vi "Variant_KVP to Strict Variant (Standard).vi"(6 "KVP":variant, 8 "Strict type matching? (F)":bool, 9 "Default Value Name (empty: label)":string, 10 "Default Value":variant, 11 "Parent Name":string) -> (0 "all found?":bool, 1 "any found?":bool, 2 "Value":variant, 3 "name out":string)   [LabVIEW 2020, in "OpenVariant.lvlib"]
doc: "This VI takes a default value as the input and replaces it recursively (cluster, array) with values found in key value pair arrays."
uses:
  OpenVariant.lvlib
  Variant_EmptyCluster.vi
  _built_ppls/OpenDescriptor.lvlibp/TypeDescriptor_SetName.vi
  <vilib>/Utility/GetType.llb/TD_Create Cluster.vi
  <vilib>/Utility/GetType.llb/TD_Get Array Information.vi
  <vilib>/Utility/GetType.llb/Get Type Code from I16 Array And Pos.vi
  _built_ppls/OpenConvert.lvlibp
  _built_ppls/OpenScalar.lvlibp
  _built_ppls/OpenDescriptor.lvlibp
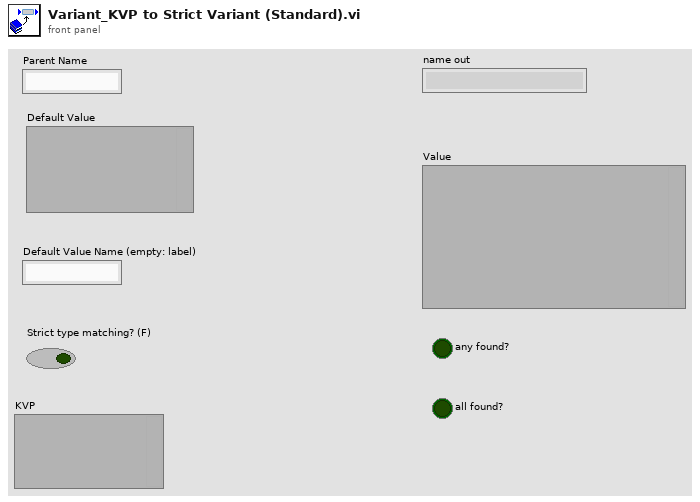
[diagram p1: front panel]
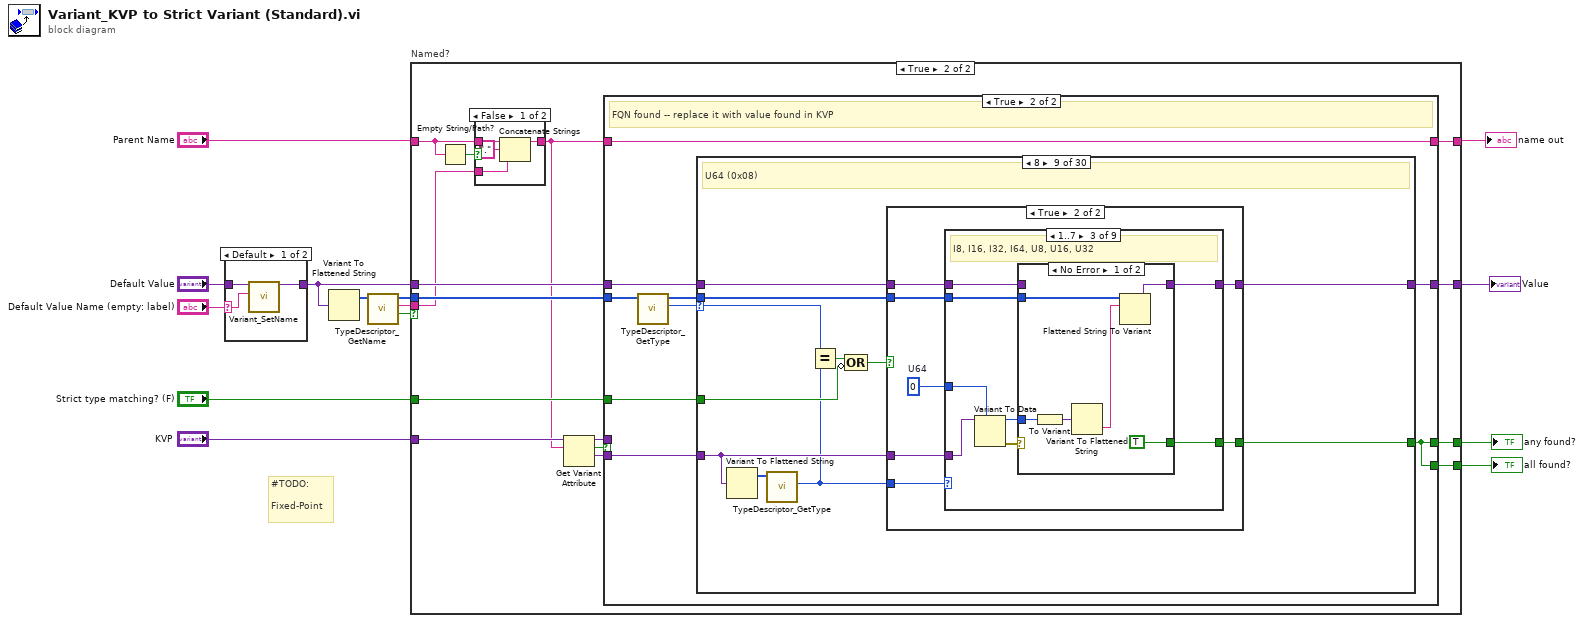
[diagram p0: block diagram]
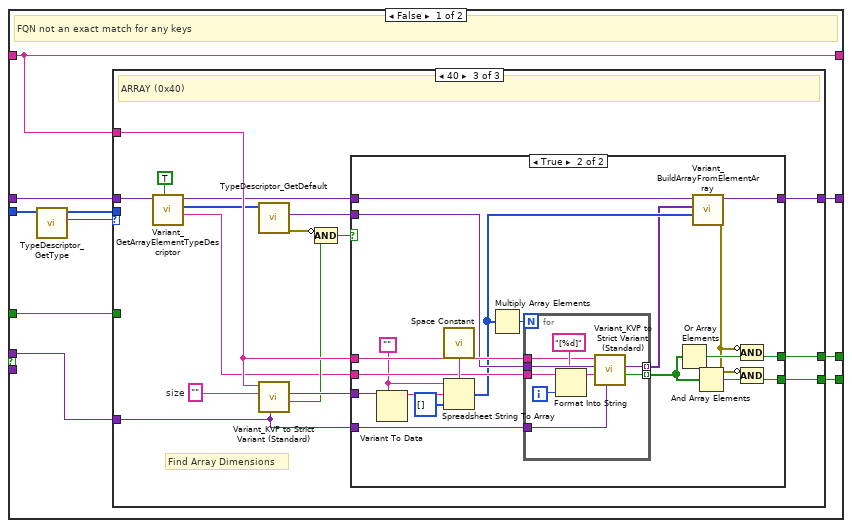
[diagram p5: hidden frame]
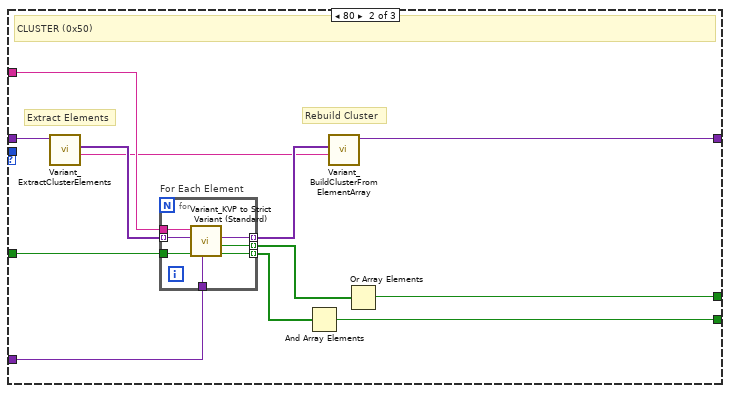
[diagram p7: hidden frame]
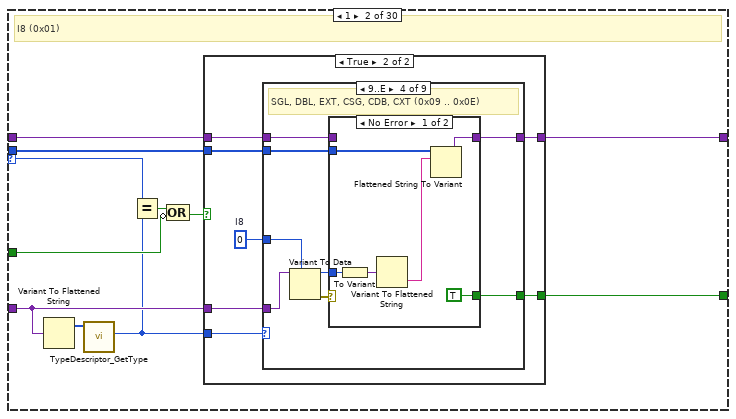
[diagram p10: hidden frame]
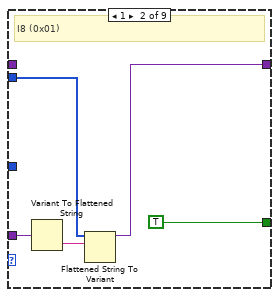
[diagram p13: hidden frame]
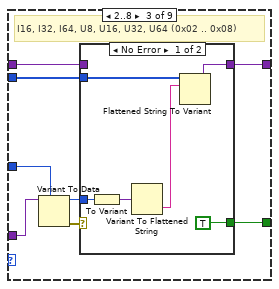
[diagram p14: hidden frame]
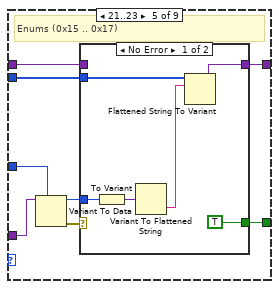
[diagram p17: hidden frame]
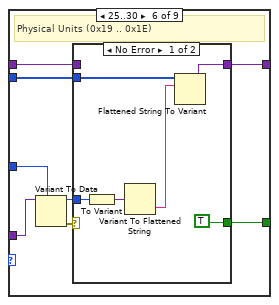
[diagram p19: hidden frame]
diagram:
  # "#TODO: \n\nFixed-Point"
  n1 = case shown="Default" "Default Value Name (empty: label)" {
    selector: "Default Value Name (empty: label)" -> [w16 _]
    tunnel: "Default Value" -> [w17 w18]
    tunnel: [w15 w18] -> w6
    frame Default {
      n2 = call "Variant_SetName.vi"("Name"=w16, "Variant"=w17) -> ("Named Variant"=w15:variant)  [unwired: 9 in]
    }
    frame "" {
    }
  }
  n3 = Variant To Flattened String(Variant=w6) -> (1:w4:i16[])  [unwired: 1 out]
  n4 = call "TypeDescriptor_GetName.vi"("type descriptor"=w4) -> ("found"=w1:bool, "name"=w2:string, "type descriptor dup"=w3:i16[])  [unwired: 8 in]
  n5 = case "Named?" shown="True" w1 {
    tunnel: [w20 w35] -> w13
    tunnel: w6 -> [w20 w34]
    tunnel: w3 -> [_ w30]
    tunnel: w2 -> [_ w26]
    tunnel: "Parent Name" -> [w19 w31]
    tunnel: [w19 w33] -> w14
    tunnel: "Strict type matching? (F)" -> [_ w29]
    tunnel: [_ w28] -> w10
    tunnel: [_ w27] -> w9
    tunnel: "KVP" -> [_ w25]
    frame False {
      # "No Name Found -- no value to replace"
    }
    frame True {
      # "Has Name?"
      n6 = Empty String/Path?(string/path=w31) -> (empty?=w32:bool)
      n7 = case shown="False" w32 {
        tunnel: w26 -> [w37 w40]
        tunnel: [w38 w40] -> w22
        tunnel: w31 -> [w39 _]
        frame False {
          n8 = Concatenate Strings(w39, "." ("string"), w37) -> (w38:string)
        }
        frame True {
        }
      }
      n9 = Get Variant Attribute(Variant=w25, name=w22) -> (duplicate Variant=w24:variant, found=w21:bool, value=w23:variant)  [unwired: 2 in, 1 out]
      n10 = case shown="True" w21 {
        tunnel: [w49 w125] -> w35
        tunnel: w34 -> [w48 w124]
        tunnel: w30 -> [w50 w123]
        tunnel: w22 -> [w46 w120]
        tunnel: [w46 w120] -> w33
        tunnel: w29 -> [w45 w119]
        tunnel: [w44 w118] -> w28
        tunnel: [w43 w118] -> w27
        tunnel: w24 -> [w41 _]
        tunnel: w23 -> [_ w117]
        frame False {
          # "FQN not an exact match for any keys"
          n11 = call "TypeDescriptor_GetType.vi"("type descriptor"=w50) -> ("Type"=w47:u8, "type descriptor dup"=w42:i16[])  [unwired: 9 in]
          n12 = case shown="40" w47 {
            tunnel: [w51 w54 w84] -> w49
            tunnel: w48 -> [w51 w63 w74]
            tunnel: w46 -> [_ w62 w81]
            tunnel: w45 -> [_ w61 _]
            tunnel: [_ w59 w86] -> w44
            tunnel: [_ w57 w85] -> w43
            tunnel: w42 -> [_ _ _]
            tunnel: w41 -> [_ w52 w71]
            frame Default {
              # "No Match"
            }
            frame 80 {
              # "Rebuild Cluster"
              # "Extract Elements"
              # "CLUSTER (0x50)"
              n13 = call "Variant_ExtractClusterElements.vi"("Cluster"=w63) -> ("name"=w53:string, "Elements"=w55:variant[])  [unwired: 8 in, 1 out]
              n14 = for "For Each Element" {
                tunnel: [w70] -> w56 mode=indexing
                tunnel: w52 -> [w69]
                tunnel: w55 -> [w68] mode=indexing
                tunnel: w62 -> [w67]
                tunnel: [w66] -> w60 mode=indexing
                tunnel: [w65] -> w58 mode=indexing
                tunnel: w61 -> [w64]
                n15 = call "Variant_KVP to Strict Variant (Standard).vi"("KVP"=w69, "Strict type matching? (F)"=w64, "Default Value"=w68, "Parent Name"=w67) -> ("all found?"=w66:bool, "any found?"=w65:bool, "Value"=w70:variant)  [unwired: 4 in, 1 out]
              }
              n16 = And Array Elements(Boolean array=w60) -> (logical AND=w59:bool)
              n17 = call "Variant_BuildClusterFromElementArray.vi"("name"=w53, "Elements"=w56) -> ("Cluster"=w54:variant)  [unwired: 9 in]
              n18 = Or Array Elements(Boolean array=w58) -> (logical OR=w57:bool)
            }
            frame 64 {
              w82 = ""  # size
              # "Find Array Dimensions"
              # "ARRAY (0x40)"
              n19 = call "Variant_GetArrayElementTypeDescriptor.vi"("Name Element if empty string (F)"=TRUE, "Array"=w74) -> ("Element Name"=w76:string, "Element Descriptor"=w75:i16[], "Array dup"=w73:variant)  [unwired: 7 in]
              n20 = call "TypeDescriptor_GetDefault.vi"("type descriptor"=w75) -> ("error out"=w72:errorcluster, "Default"=w79:variant)  [unwired: 8 in, 1 out]
              n21 = call "Variant_KVP to Strict Variant (Standard).vi"("KVP"=w71, "Default Value"=w82, "Parent Name"=w81) -> ("any found?"=w78:bool, "Value"=w83:variant)  [unwired: 5 in, 2 out]
              n22 = Compound Arithmetic op=AND(invert w72, w78) -> (w77:bool)
              n23 = case shown="True" w77 {
                tunnel: [_ w91] -> w86
                tunnel: [_ w94] -> w85
                tunnel: [w87 w96] -> w84
                tunnel: w71 -> [_ w103]
                tunnel: w83 -> [_ w102]
                tunnel: w81 -> [_ w100]
                tunnel: w76 -> [_ w99]
                tunnel: w73 -> [w87 w97]
                tunnel: w79 -> [_ w90]
                frame False {
                  # "No Array Dimensions Found in the key value pairs"
                }
                frame True {
                  w98 = "" ("format string")
                  n24 = Variant To Data(type=w98, Variant=w102) -> (data=w101:string)  [unwired: 1 in, 1 out]
                  n25 = call <vilib>:"Space Constant.vi"() -> ("String"=w104:string)
                  n26 = Spreadsheet String To Array(delimiter (Tab)=w104, format string=w98, spreadsheet string=w101, array type (2D Dbl)=u32[] [] ("Dimensions")) -> (array=w89:u32[])
                  n27 = Multiply Array Elements(1:w89) -> (0:w107:u32)
                  n28 = for {
                    N: w107 -> [_]
                    tunnel: w90 -> [w116]
                    tunnel: w103 -> [w113]
                    tunnel: w100 -> [w112]
                    tunnel: [w111] -> w106 mode=indexing
                    tunnel: w99 -> [w110]
                    tunnel: [w108] -> w88 mode=indexing
                    i -> [w109]
                    n29 = Format Into String(format string="[%d]", initial string=w110, w109) -> (resulting string=w114:string)  [unwired: 1 in, 1 out]
                    n30 = call "Variant_KVP to Strict Variant (Standard).vi"("KVP"=w113, "Default Value Name (empty: label)"=w114, "Default Value"=w116, "Parent Name"=w112) -> ("any found?"=w111:bool, "Value"=w108:variant)  [unwired: 4 in, 2 out]
                  }
                  n31 = Or Array Elements(Boolean array=w106) -> (logical OR=w95:bool)
                  n32 = call "Variant_BuildArrayFromElementArray.vi"("Dimensions"=w89, "Elements"=w88, "Default Array"=w97) -> ("error out"=w93:errorcluster, "Output Array"=w96:variant)  [unwired: 7 in]
                  n33 = And Array Elements(Boolean array=w106) -> (logical AND=w92:bool)
                  n34 = Compound Arithmetic op=AND(invert w93, w95) -> (w94:bool)
                  n35 = Compound Arithmetic op=AND(invert w93, w92) -> (w91:bool)
                }
              }
            }
          }
        }
        frame True {
          # "FQN found -- replace it with value found in KVP"
          n36 = call "TypeDescriptor_GetType.vi"("type descriptor"=w123) -> ("Type"=w121:u8, "type descriptor dup"=w122:i16[])  [unwired: 9 in]
          n37 = case shown="8" w121 {
            selector: w121 -> [_ w128 w260 w390 w522 w653 w784 w915 w1046 w1176 w1263 w1350 w1437 w1523 w1608 w1694 w1799 w1903 w2005 w2077 w2146 w2217 w2287 w2356 w2426 w2484 w2779 w2837 _ w2880]
            tunnel: w117 -> [_ w133 w264 w395 w526 w657 w788 w919 w1050 w1181 w1268 w1354 w1441 w1528 w1613 w1699 w1804 w1908 w2011 w2081 w2151 w2221 w2291 w2361 w2431 w2490 w2788 w2828 w2857 w2894]
            tunnel: [w126 w135 w266 w397 w528 w659 w790 w921 w1052 w1183 w1270 w1356 w1443 w1530 w1615 w1701 w1806 w1910 w2013 w2083 w2153 w2223 w2293 w2363 w2433 w2493 w2784 w2840 w2866 w2890] -> w125
            tunnel: w124 -> [w126 w136 w267 w398 w529 w660 w791 w922 w1053 w1184 w1271 w1357 w1444 w1526 w1616 w1702 w1807 w1911 w2014 w2084 w2154 w2224 w2294 w2364 w2434 w2494 w2785 w2841 w2868 w2891]
            tunnel: w122 -> [_ w134 w265 w396 w527 w658 w789 w920 w1051 w1182 w1269 w1355 w1442 w1529 w1614 w1700 w1805 w1909 w2012 w2082 w2152 w2222 w2292 w2362 w2432 w2492 w2783 w2827 _ w2887]
            tunnel: [_ w132 w263 w394 w525 w656 w787 w918 w1049 w1180 w1267 w1353 w1440 w1527 w1612 w1698 w1803 w1907 w2010 w2080 w2150 w2220 w2290 w2360 w2430 w2487 w2781 w2839 w2867 w2885] -> w118
            tunnel: w119 -> [_ w129 w258 w391 w520 w651 w783 w913 w1045 w1177 w1264 w1348 w1435 w1522 w1609 w1695 w1800 w1904 w2007 w2075 w2147 w2216 w2285 w2357 w2427 w2482 w2777 w2830 w2865 w2882]
            frame Default {
            }
            frame 1 {
              # "I8 (0x01)"
              n38 = Variant To Flattened String(Variant=w133) -> (1:w137:i16[])  [unwired: 1 out]
              n39 = call "TypeDescriptor_GetType.vi"("type descriptor"=w137) -> ("Type"=w127:u8)  [unwired: 9 in, 1 out]
              n40 = Equal?(x=w128, y=w127) -> (x = y?=w131:bool)
              n41 = Compound Arithmetic op=OR(w131, invert w129) -> (w130:bool)
              n42 = case shown="True" w130 {
                tunnel: w136 -> [w138 w145]
                tunnel: [w138 w144] -> w135
                tunnel: w134 -> [_ w143]
                tunnel: w127 -> [_ w142]
                tunnel: w133 -> [_ w140]
                tunnel: [_ w139] -> w132
                frame False {
                }
                frame True {
                  w141 = i8 0  # I8
                  n43 = case shown="9..E" w142 {
                    tunnel: w145 -> [w146 _ w156 w171 w186 w201 w213 w235 _]
                    tunnel: [w146 w148 w158 w173 w188 w203 w219 w237 w256] -> w144
                    tunnel: w143 -> [_ w149 w159 w174 w189 w204 w220 w239 w257]
                    tunnel: w141 -> [_ _ w154 w169 w184 w199 w214 w233 w255]
                    tunnel: w140 -> [_ w151 w153 w168 w183 w198 w218 w232 w251]
                    tunnel: [_ TRUE w152 w167 w182 w197 w212 w231 TRUE] -> w139
                    frame Default {
                      # "INCOMPATIBLE DATATYPES"
                    }
                    frame 1 {
                      # "I8 (0x01)"
                      n44 = Variant To Flattened String(Variant=w151) -> (data string=w150:string)  [unwired: 1 out]
                      n45 = Flattened String To Variant(6:w150, 7:w149) -> (3:w148:variant)  [unwired: 1 in, 1 out]
                    }
                    frame 2..8 {
                      # "I16, I32, I64, U8, U16, U32, U64 (0x02 .. 0x08)"
                      n46 = Variant To Data(type=w154, Variant=w153) -> (data=w155:i8, error out=w157:errorcluster)  [unwired: 1 in]
                      n47 = case shown="No Error" w157 {
                        tunnel: w159 -> [w165 _]
                        tunnel: [w164 w166] -> w158
                        tunnel: w156 -> [_ w166]
                        tunnel: w155 -> [w162 _]
                        tunnel: [TRUE _] -> w152
                        frame No Error {
                          n48 = To Variant(anything=w162) -> (Variant=w161:variant)
                          n49 = Variant To Flattened String(Variant=w161) -> (data string=w163:string)  [unwired: 1 out]
                          n50 = Flattened String To Variant(6:w163, 7:w165) -> (3:w164:variant)  [unwired: 1 in, 1 out]
                        }
                        frame Error {
                        }
                      }
                    }
                    frame 9..14 {
                      # "SGL, DBL, EXT, CSG, CDB, CXT (0x09 .. 0x0E)"
                      n51 = Variant To Data(type=w169, Variant=w168) -> (data=w170:i8, error out=w172:errorcluster)  [unwired: 1 in]
                      n52 = case shown="No Error" w172 {
                        tunnel: w174 -> [w180 _]
                        tunnel: [w179 w181] -> w173
                        tunnel: w171 -> [_ w181]
                        tunnel: w170 -> [w177 _]
                        tunnel: [TRUE _] -> w167
                        frame No Error {
                          n53 = To Variant(anything=w177) -> (Variant=w176:variant)
                          n54 = Variant To Flattened String(Variant=w176) -> (data string=w178:string)  [unwired: 1 out]
                          n55 = Flattened String To Variant(6:w178, 7:w180) -> (3:w179:variant)  [unwired: 1 in, 1 out]
                        }
                        frame Error {
                        }
                      }
                    }
                    frame 21..23 {
                      # "Enums (0x15 .. 0x17)"
                      n56 = Variant To Data(type=w184, Variant=w183) -> (data=w185:i8, error out=w187:errorcluster)  [unwired: 1 in]
                      n57 = case shown="No Error" w187 {
                        tunnel: w189 -> [w195 _]
                        tunnel: [w194 w196] -> w188
                        tunnel: w186 -> [_ w196]
                        tunnel: w185 -> [w192 _]
                        tunnel: [TRUE _] -> w182
                        frame No Error {
                          n58 = To Variant(anything=w192) -> (Variant=w191:variant)
                          n59 = Variant To Flattened String(Variant=w191) -> (data string=w193:string)  [unwired: 1 out]
                          n60 = Flattened String To Variant(6:w193, 7:w195) -> (3:w194:variant)  [unwired: 1 in, 1 out]
                        }
                        frame Error {
                        }
                      }
                    }
                    frame 25..30 {
                      # "Physical Units (0x19 .. 0x1E)"
                      n61 = Variant To Data(type=w199, Variant=w198) -> (data=w200:i8, error out=w202:errorcluster)  [unwired: 1 in]
                      n62 = case shown="No Error" w202 {
                        tunnel: w204 -> [w210 _]
                        tunnel: [w209 w211] -> w203
                        tunnel: w201 -> [_ w211]
                        tunnel: w200 -> [w207 _]
                        tunnel: [TRUE _] -> w197
                        frame No Error {
                          n63 = To Variant(anything=w207) -> (Variant=w206:variant)
                          n64 = Variant To Flattened String(Variant=w206) -> (data string=w208:string)  [unwired: 1 out]
                          n65 = Flattened String To Variant(6:w208, 7:w210) -> (3:w209:variant)  [unwired: 1 in, 1 out]
                        }
                        frame Error {
                        }
                      }
                    }
                    frame 33 {
                      # "Boolean (0x21)"
                      n66 = Variant To Data(type=FALSE, Variant=w218) -> (data=w215:bool, error out=w216:errorcluster)  [unwired: 1 in]
                      n67 = case shown="No Error" w216 {
                        tunnel: w220 -> [w229 _]
                        tunnel: [w228 w230] -> w219
                        tunnel: w215 -> [w225 _]
                        tunnel: w214 -> [w223 _]
                        tunnel: w213 -> [_ w230]
                        tunnel: [TRUE _] -> w212
                        frame No Error {
                          n68 = Boolean To (0,1)(Boolean=w225) -> (0, 1=w224:i16)
                          n69 = Variant To Data(type=w223, Variant=w224) -> (data=w222:i8)  [unwired: 1 in, 1 out]
                          n70 = To Variant(anything=w222) -> (Variant=w226:variant)
                          n71 = Variant To Flattened String(Variant=w226) -> (data string=w227:string)  [unwired: 1 out]
                          n72 = Flattened String To Variant(6:w227, 7:w229) -> (3:w228:variant)  [unwired: 1 in, 1 out]
                        }
                        frame Error {
                        }
                      }
                    }
                    frame 48 {
                      # "STRING (0x30)"
                      n73 = Variant To Data(type="", Variant=w232) -> (data=w234:string, error out=w236:errorcluster)  [unwired: 1 in]
                      n74 = case shown="No Error" w236 {
                        tunnel: w239 -> [w247 _]
                        tunnel: [w246 w248] -> w237
                        tunnel: w235 -> [_ w248]
                        tunnel: w234 -> [w243 _]
                        tunnel: w233 -> [w241 _]
                        tunnel: [TRUE _] -> w231
                        frame No Error {
                          n75 = Fract/Exp String To Number(string=w243, default (0 dbl)=w241) -> (number=w242:i8)  [unwired: 2 in, 1 out]
                          n76 = To Variant(anything=w242) -> (Variant=w245:variant)
                          n77 = Variant To Flattened String(Variant=w245) -> (data string=w244:string)  [unwired: 1 out]
                          n78 = Flattened String To Variant(6:w244, 7:w247) -> (3:w246:variant)  [unwired: 1 in, 1 out]
                        }
                        frame Error {
                        }
                      }
                    }
                    frame 112 {
                      # "Refnum (0x70)"
                      n79 = Variant To Flattened String(Variant=w251) -> (data string=w250:string)  [unwired: 1 out]
                      n80 = Type Cast(type=w255, x=w250) -> (*(type *) &x=w254:i8)
                      n81 = To Variant(anything=w254) -> (Variant=w253:variant)
                      n82 = Variant To Flattened String(Variant=w253) -> (data string=w252:string)  [unwired: 1 out]
                      n83 = Flattened String To Variant(6:w252, 7:w257) -> (3:w256:variant)  [unwired: 1 in, 1 out]
                    }
                  }
                }
              }
            }
            frame 2 {
              # "I16 (0x02)"
              n84 = Variant To Flattened String(Variant=w264) -> (1:w268:i16[])  [unwired: 1 out]
              n85 = call "TypeDescriptor_GetType.vi"("type descriptor"=w268) -> ("Type"=w259:u8)  [unwired: 9 in, 1 out]
              n86 = Equal?(x=w260, y=w259) -> (x = y?=w262:bool)
              n87 = Compound Arithmetic op=OR(w262, invert w258) -> (w261:bool)
              n88 = case shown="True" w261 {
                tunnel: w267 -> [w269 w276]
                tunnel: [w269 w275] -> w266
                tunnel: w265 -> [_ w274]
                tunnel: w259 -> [_ w273]
                tunnel: w264 -> [_ w271]
                tunnel: [_ w270] -> w263
                frame False {
                }
                frame True {
                  w272 = i16 0  # I16
                  n89 = case shown="2" w273 {
                    tunnel: w276 -> [w277 _ w287 w302 w317 w332 w344 w366 _]
                    tunnel: [w277 w279 w289 w304 w319 w334 w350 w368 w387] -> w275
                    tunnel: w274 -> [_ w280 w290 w305 w320 w335 w351 w370 w388]
                    tunnel: w272 -> [_ _ w285 w300 w315 w330 w345 w364 w386]
                    tunnel: w271 -> [_ w282 w284 w299 w314 w329 w349 w363 w382]
                    tunnel: [_ TRUE w283 w298 w313 w328 w343 w362 TRUE] -> w270
                    frame Default {
                      # "INCOMPATIBLE DATATYPES"
                    }
                    frame 2 {
                      # "I16 (0x02)"
                      n90 = Variant To Flattened String(Variant=w282) -> (data string=w281:string)  [unwired: 1 out]
                      n91 = Flattened String To Variant(6:w281, 7:w280) -> (3:w279:variant)  [unwired: 1 in, 1 out]
                    }
                    frame 1, 3..8 {
                      # "I8, I32, I64, U8, U16, U32, U64 (0x02 .. 0x08)"
                      n92 = Variant To Data(type=w285, Variant=w284) -> (data=w286:i16, error out=w288:errorcluster)  [unwired: 1 in]
                      n93 = case shown="No Error" w288 {
                        tunnel: w290 -> [w296 _]
                        tunnel: [w295 w297] -> w289
                        tunnel: w287 -> [_ w297]
                        tunnel: w286 -> [w293 _]
                        tunnel: [TRUE _] -> w283
                        frame No Error {
                          n94 = To Variant(anything=w293) -> (Variant=w292:variant)
                          n95 = Variant To Flattened String(Variant=w292) -> (data string=w294:string)  [unwired: 1 out]
                          n96 = Flattened String To Variant(6:w294, 7:w296) -> (3:w295:variant)  [unwired: 1 in, 1 out]
                        }
                        frame Error {
                        }
                      }
                    }
                    frame 9..14 {
                      # "SGL, DBL, EXT, CSG, CDB, CXT (0x09 .. 0x0E)"
                      n97 = Variant To Data(type=w300, Variant=w299) -> (data=w301:i16, error out=w303:errorcluster)  [unwired: 1 in]
                      n98 = case shown="No Error" w303 {
                        tunnel: w305 -> [w311 _]
                        tunnel: [w310 w312] -> w304
                        tunnel: w302 -> [_ w312]
                        tunnel: w301 -> [w308 _]
                        tunnel: [TRUE _] -> w298
                        frame No Error {
                          n99 = To Variant(anything=w308) -> (Variant=w307:variant)
                          n100 = Variant To Flattened String(Variant=w307) -> (data string=w309:string)  [unwired: 1 out]
                          n101 = Flattened String To Variant(6:w309, 7:w311) -> (3:w310:variant)  [unwired: 1 in, 1 out]
                        }
                        frame Error {
                        }
                      }
                    }
                    frame 21..23 {
                      # "Enums (0x15 .. 0x17)"
                      n102 = Variant To Data(type=w315, Variant=w314) -> (data=w316:i16, error out=w318:errorcluster)  [unwired: 1 in]
                      n103 = case shown="No Error" w318 {
                        tunnel: w320 -> [w326 _]
                        tunnel: [w325 w327] -> w319
                        tunnel: w317 -> [_ w327]
                        tunnel: w316 -> [w323 _]
                        tunnel: [TRUE _] -> w313
                        frame No Error {
                          n104 = To Variant(anything=w323) -> (Variant=w322:variant)
                          n105 = Variant To Flattened String(Variant=w322) -> (data string=w324:string)  [unwired: 1 out]
                          n106 = Flattened String To Variant(6:w324, 7:w326) -> (3:w325:variant)  [unwired: 1 in, 1 out]
                        }
                        frame Error {
                        }
                      }
                    }
                    frame 25..30 {
                      # "Physical Units (0x19 .. 0x1E)"
                      n107 = Variant To Data(type=w330, Variant=w329) -> (data=w331:i16, error out=w333:errorcluster)  [unwired: 1 in]
                      n108 = case shown="No Error" w333 {
                        tunnel: w335 -> [w341 _]
                        tunnel: [w340 w342] -> w334
                        tunnel: w332 -> [_ w342]
                        tunnel: w331 -> [w338 _]
                        tunnel: [TRUE _] -> w328
                        frame No Error {
                          n109 = To Variant(anything=w338) -> (Variant=w337:variant)
                          n110 = Variant To Flattened String(Variant=w337) -> (data string=w339:string)  [unwired: 1 out]
                          n111 = Flattened String To Variant(6:w339, 7:w341) -> (3:w340:variant)  [unwired: 1 in, 1 out]
                        }
                        frame Error {
                        }
                      }
                    }
                    frame 33 {
                      # "Boolean (0x21)"
                      n112 = Variant To Data(type=FALSE, Variant=w349) -> (data=w346:bool, error out=w347:errorcluster)  [unwired: 1 in]
                      n113 = case shown="No Error" w347 {
                        tunnel: w351 -> [w360 _]
                        tunnel: [w359 w361] -> w350
                        tunnel: w346 -> [w356 _]
                        tunnel: w345 -> [w354 _]
                        tunnel: w344 -> [_ w361]
                        tunnel: [TRUE _] -> w343
                        frame No Error {
                          n114 = Boolean To (0,1)(Boolean=w356) -> (0, 1=w355:i16)
                          n115 = Variant To Data(type=w354, Variant=w355) -> (data=w353:i16)  [unwired: 1 in, 1 out]
                          n116 = To Variant(anything=w353) -> (Variant=w357:variant)
                          n117 = Variant To Flattened String(Variant=w357) -> (data string=w358:string)  [unwired: 1 out]
                          n118 = Flattened String To Variant(6:w358, 7:w360) -> (3:w359:variant)  [unwired: 1 in, 1 out]
                        }
                        frame Error {
                        }
                      }
                    }
                    frame 48 {
                      # "STRING (0x30)"
                      n119 = Variant To Data(type="", Variant=w363) -> (data=w365:string, error out=w367:errorcluster)  [unwired: 1 in]
                      n120 = case shown="No Error" w367 {
                        tunnel: w370 -> [w378 _]
                        tunnel: [w377 w379] -> w368
                        tunnel: w366 -> [_ w379]
                        tunnel: w365 -> [w374 _]
                        tunnel: w364 -> [w372 _]
                        tunnel: [TRUE _] -> w362
                        frame No Error {
                          n121 = Fract/Exp String To Number(string=w374, default (0 dbl)=w372) -> (number=w373:i16)  [unwired: 2 in, 1 out]
                          n122 = To Variant(anything=w373) -> (Variant=w376:variant)
                          n123 = Variant To Flattened String(Variant=w376) -> (data string=w375:string)  [unwired: 1 out]
                          n124 = Flattened String To Variant(6:w375, 7:w378) -> (3:w377:variant)  [unwired: 1 in, 1 out]
                        }
                        frame Error {
                        }
                      }
                    }
                    frame 112 {
                      # "Refnum (0x70)"
                      n125 = Variant To Flattened String(Variant=w382) -> (data string=w381:string)  [unwired: 1 out]
                      n126 = Type Cast(type=w386, x=w381) -> (*(type *) &x=w385:i16)
                      n127 = To Variant(anything=w385) -> (Variant=w384:variant)
                      n128 = Variant To Flattened String(Variant=w384) -> (data string=w383:string)  [unwired: 1 out]
                      n129 = Flattened String To Variant(6:w383, 7:w388) -> (3:w387:variant)  [unwired: 1 in, 1 out]
                    }
                  }
                }
              }
            }
            frame 3 {
              # "I32 (0x03)"
              n130 = Variant To Flattened String(Variant=w395) -> (1:w399:i16[])  [unwired: 1 out]
              n131 = call "TypeDescriptor_GetType.vi"("type descriptor"=w399) -> ("Type"=w389:u8)  [unwired: 9 in, 1 out]
              n132 = Equal?(x=w390, y=w389) -> (x = y?=w393:bool)
              n133 = Compound Arithmetic op=OR(w393, invert w391) -> (w392:bool)
              n134 = case shown="True" w392 {
                tunnel: w398 -> [w400 w407]
                tunnel: [w400 w406] -> w397
                tunnel: w396 -> [_ w405]
                tunnel: w389 -> [_ w404]
                tunnel: w395 -> [_ w402]
                tunnel: [_ w401] -> w394
                frame False {
                }
                frame True {
                  w403 = 0  # I32
                  n135 = case shown="21" w404 {
                    tunnel: w407 -> [w408 _ w418 w433 w448 w463 w475 w497 _]
                    tunnel: [w408 w410 w420 w435 w450 w465 w481 w499 w518] -> w406
                    tunnel: w405 -> [_ w411 w421 w436 w451 w466 w482 w501 w519]
                    tunnel: w403 -> [_ _ w416 w431 w446 w461 w476 w495 w517]
                    tunnel: w402 -> [_ w413 w415 w430 w445 w460 w480 w494 w513]
                    tunnel: [_ TRUE w414 w429 w444 w459 w474 w493 TRUE] -> w401
                    frame Default {
                      # "INCOMPATIBLE DATATYPES"
                    }
                    frame 3 {
                      # "I32 (0x03)"
                      n136 = Variant To Flattened String(Variant=w413) -> (data string=w412:string)  [unwired: 1 out]
                      n137 = Flattened String To Variant(6:w412, 7:w411) -> (3:w410:variant)  [unwired: 1 in, 1 out]
                    }
                    frame 1, 2, 4..8 {
                      # "I8, I16, I64, U8, U16, U32, U64 (0x02 .. 0x08)"
                      n138 = Variant To Data(type=w416, Variant=w415) -> (data=w417:i32, error out=w419:errorcluster)  [unwired: 1 in]
                      n139 = case shown="No Error" w419 {
                        tunnel: w421 -> [w427 _]
                        tunnel: [w426 w428] -> w420
                        tunnel: w418 -> [_ w428]
                        tunnel: w417 -> [w424 _]
                        tunnel: [TRUE _] -> w414
                        frame No Error {
                          n140 = To Variant(anything=w424) -> (Variant=w423:variant)
                          n141 = Variant To Flattened String(Variant=w423) -> (data string=w425:string)  [unwired: 1 out]
                          n142 = Flattened String To Variant(6:w425, 7:w427) -> (3:w426:variant)  [unwired: 1 in, 1 out]
                        }
                        frame Error {
                        }
                      }
                    }
                    frame 9..14 {
                      # "SGL, DBL, EXT, CSG, CDB, CXT (0x09 .. 0x0E)"
                      n143 = Variant To Data(type=w431, Variant=w430) -> (data=w432:i32, error out=w434:errorcluster)  [unwired: 1 in]
                      n144 = case shown="No Error" w434 {
                        tunnel: w436 -> [w442 _]
                        tunnel: [w441 w443] -> w435
                        tunnel: w433 -> [_ w443]
                        tunnel: w432 -> [w439 _]
                        tunnel: [TRUE _] -> w429
                        frame No Error {
                          n145 = To Variant(anything=w439) -> (Variant=w438:variant)
                          n146 = Variant To Flattened String(Variant=w438) -> (data string=w440:string)  [unwired: 1 out]
                          n147 = Flattened String To Variant(6:w440, 7:w442) -> (3:w441:variant)  [unwired: 1 in, 1 out]
                        }
                        frame Error {
                        }
                      }
                    }
                    frame 21..23 {
                      # "Enums (0x15 .. 0x17)"
                      n148 = Variant To Data(type=w446, Variant=w445) -> (data=w447:i32, error out=w449:errorcluster)  [unwired: 1 in]
                      n149 = case shown="No Error" w449 {
                        tunnel: w451 -> [w457 _]
                        tunnel: [w456 w458] -> w450
                        tunnel: w448 -> [_ w458]
                        tunnel: w447 -> [w454 _]
                        tunnel: [TRUE _] -> w444
                        frame No Error {
                          n150 = To Variant(anything=w454) -> (Variant=w453:variant)
                          n151 = Variant To Flattened String(Variant=w453) -> (data string=w455:string)  [unwired: 1 out]
                          n152 = Flattened String To Variant(6:w455, 7:w457) -> (3:w456:variant)  [unwired: 1 in, 1 out]
                        }
                        frame Error {
                        }
                      }
                    }
                    frame 25..30 {
                      # "Physical Units (0x19 .. 0x1E)"
                      n153 = Variant To Data(type=w461, Variant=w460) -> (data=w462:i32, error out=w464:errorcluster)  [unwired: 1 in]
                      n154 = case shown="No Error" w464 {
                        tunnel: w466 -> [w472 _]
                        tunnel: [w471 w473] -> w465
                        tunnel: w463 -> [_ w473]
                        tunnel: w462 -> [w469 _]
                        tunnel: [TRUE _] -> w459
                        frame No Error {
                          n155 = To Variant(anything=w469) -> (Variant=w468:variant)
                          n156 = Variant To Flattened String(Variant=w468) -> (data string=w470:string)  [unwired: 1 out]
                          n157 = Flattened String To Variant(6:w470, 7:w472) -> (3:w471:variant)  [unwired: 1 in, 1 out]
                        }
                        frame Error {
                        }
                      }
                    }
                    frame 33 {
                      # "Boolean (0x21)"
                      n158 = Variant To Data(type=FALSE, Variant=w480) -> (data=w477:bool, error out=w478:errorcluster)  [unwired: 1 in]
                      n159 = case shown="No Error" w478 {
                        tunnel: w482 -> [w491 _]
                        tunnel: [w490 w492] -> w481
                        tunnel: w477 -> [w487 _]
                        tunnel: w476 -> [w485 _]
                        tunnel: w475 -> [_ w492]
                        tunnel: [TRUE _] -> w474
                        frame No Error {
                          n160 = Boolean To (0,1)(Boolean=w487) -> (0, 1=w486:i16)
                          n161 = Variant To Data(type=w485, Variant=w486) -> (data=w484:i32)  [unwired: 1 in, 1 out]
                          n162 = To Variant(anything=w484) -> (Variant=w488:variant)
                          n163 = Variant To Flattened String(Variant=w488) -> (data string=w489:string)  [unwired: 1 out]
                          n164 = Flattened String To Variant(6:w489, 7:w491) -> (3:w490:variant)  [unwired: 1 in, 1 out]
                        }
                        frame Error {
                        }
                      }
                    }
                    frame 48 {
                      # "STRING (0x30)"
                      n165 = Variant To Data(type="", Variant=w494) -> (data=w496:string, error out=w498:errorcluster)  [unwired: 1 in]
                      n166 = case shown="No Error" w498 {
                        tunnel: w501 -> [w509 _]
                        tunnel: [w508 w510] -> w499
                        tunnel: w497 -> [_ w510]
                        tunnel: w496 -> [w505 _]
                        tunnel: w495 -> [w503 _]
                        tunnel: [TRUE _] -> w493
                        frame No Error {
                          n167 = Fract/Exp String To Number(string=w505, default (0 dbl)=w503) -> (number=w504:i32)  [unwired: 2 in, 1 out]
                          n168 = To Variant(anything=w504) -> (Variant=w507:variant)
                          n169 = Variant To Flattened String(Variant=w507) -> (data string=w506:string)  [unwired: 1 out]
                          n170 = Flattened String To Variant(6:w506, 7:w509) -> (3:w508:variant)  [unwired: 1 in, 1 out]
                        }
                        frame Error {
                        }
                      }
                    }
                    frame 112 {
                      # "Refnum (0x70)"
                      n171 = Variant To Flattened String(Variant=w513) -> (data string=w512:string)  [unwired: 1 out]
                      n172 = Type Cast(type=w517, x=w512) -> (*(type *) &x=w516:i32)
                      n173 = To Variant(anything=w516) -> (Variant=w515:variant)
                      n174 = Variant To Flattened String(Variant=w515) -> (data string=w514:string)  [unwired: 1 out]
                      n175 = Flattened String To Variant(6:w514, 7:w519) -> (3:w518:variant)  [unwired: 1 in, 1 out]
                    }
                  }
                }
              }
            }
            frame 4 {
              # "I64 (0x04)"
              n176 = Variant To Flattened String(Variant=w526) -> (1:w530:i16[])  [unwired: 1 out]
              n177 = call "TypeDescriptor_GetType.vi"("type descriptor"=w530) -> ("Type"=w521:u8)  [unwired: 9 in, 1 out]
              n178 = Equal?(x=w522, y=w521) -> (x = y?=w524:bool)
              n179 = Compound Arithmetic op=OR(w524, invert w520) -> (w523:bool)
              n180 = case shown="True" w523 {
                tunnel: w529 -> [w531 w538]
                tunnel: [w531 w537] -> w528
                tunnel: w527 -> [_ w536]
                tunnel: w521 -> [_ w535]
                tunnel: w526 -> [_ w533]
                tunnel: [_ w532] -> w525
                frame False {
                }
                frame True {
                  w534 = i64 0  # I64
                  n181 = case shown="1..3, 5..8" w535 {
                    tunnel: w538 -> [w539 _ w549 w564 w579 w594 w606 w628 _]
                    tunnel: [w539 w541 w551 w566 w581 w596 w612 w630 w649] -> w537
                    tunnel: w536 -> [_ w542 w552 w567 w582 w597 w613 w632 w650]
                    tunnel: w534 -> [_ _ w547 w562 w577 w592 w607 w626 w648]
                    tunnel: w533 -> [_ w544 w546 w561 w576 w591 w611 w625 w644]
                    tunnel: [_ TRUE w545 w560 w575 w590 w605 w624 TRUE] -> w532
                    frame Default {
                      # "INCOMPATIBLE DATATYPES"
                    }
                    frame 4 {
                      # "I64 (0x04)"
                      n182 = Variant To Flattened String(Variant=w544) -> (data string=w543:string)  [unwired: 1 out]
                      n183 = Flattened String To Variant(6:w543, 7:w542) -> (3:w541:variant)  [unwired: 1 in, 1 out]
                    }
                    frame 1..3, 5..8 {
                      # "I8, I16, I32, U8, U16, U32, U64"
                      n184 = Variant To Data(type=w547, Variant=w546) -> (data=w548:i64, error out=w550:errorcluster)  [unwired: 1 in]
                      n185 = case shown="No Error" w550 {
                        tunnel: w552 -> [w558 _]
                        tunnel: [w557 w559] -> w551
                        tunnel: w549 -> [_ w559]
                        tunnel: w548 -> [w555 _]
                        tunnel: [TRUE _] -> w545
                        frame No Error {
                          n186 = To Variant(anything=w555) -> (Variant=w554:variant)
                          n187 = Variant To Flattened String(Variant=w554) -> (data string=w556:string)  [unwired: 1 out]
                          n188 = Flattened String To Variant(6:w556, 7:w558) -> (3:w557:variant)  [unwired: 1 in, 1 out]
                        }
                        frame Error {
                        }
                      }
                    }
                    frame 9..14 {
                      # "SGL, DBL, EXT, CSG, CDB, CXT (0x09 .. 0x0E)"
                      n189 = Variant To Data(type=w562, Variant=w561) -> (data=w563:i64, error out=w565:errorcluster)  [unwired: 1 in]
                      n190 = case shown="No Error" w565 {
                        tunnel: w567 -> [w573 _]
                        tunnel: [w572 w574] -> w566
                        tunnel: w564 -> [_ w574]
                        tunnel: w563 -> [w570 _]
                        tunnel: [TRUE _] -> w560
                        frame No Error {
                          n191 = To Variant(anything=w570) -> (Variant=w569:variant)
                          n192 = Variant To Flattened String(Variant=w569) -> (data string=w571:string)  [unwired: 1 out]
                          n193 = Flattened String To Variant(6:w571, 7:w573) -> (3:w572:variant)  [unwired: 1 in, 1 out]
                        }
                        frame Error {
                        }
                      }
                    }
                    frame 21..23 {
                      # "Enums (0x15 .. 0x17)"
                      n194 = Variant To Data(type=w577, Variant=w576) -> (data=w578:i64, error out=w580:errorcluster)  [unwired: 1 in]
                      n195 = case shown="No Error" w580 {
                        tunnel: w582 -> [w588 _]
                        tunnel: [w587 w589] -> w581
                        tunnel: w579 -> [_ w589]
                        tunnel: w578 -> [w585 _]
                        tunnel: [TRUE _] -> w575
                        frame No Error {
                          n196 = To Variant(anything=w585) -> (Variant=w584:variant)
                          n197 = Variant To Flattened String(Variant=w584) -> (data string=w586:string)  [unwired: 1 out]
                          n198 = Flattened String To Variant(6:w586, 7:w588) -> (3:w587:variant)  [unwired: 1 in, 1 out]
                        }
                        frame Error {
                        }
                      }
                    }
                    frame 25..30 {
                      # "Physical Units (0x19 .. 0x1E)"
                      n199 = Variant To Data(type=w592, Variant=w591) -> (data=w593:i64, error out=w595:errorcluster)  [unwired: 1 in]
                      n200 = case shown="No Error" w595 {
                        tunnel: w597 -> [w603 _]
                        tunnel: [w602 w604] -> w596
                        tunnel: w594 -> [_ w604]
                        tunnel: w593 -> [w600 _]
                        tunnel: [TRUE _] -> w590
                        frame No Error {
                          n201 = To Variant(anything=w600) -> (Variant=w599:variant)
                          n202 = Variant To Flattened String(Variant=w599) -> (data string=w601:string)  [unwired: 1 out]
                          n203 = Flattened String To Variant(6:w601, 7:w603) -> (3:w602:variant)  [unwired: 1 in, 1 out]
                        }
                        frame Error {
                        }
                      }
                    }
                    frame 33 {
                      # "Boolean (0x21)"
                      n204 = Variant To Data(type=FALSE, Variant=w611) -> (data=w608:bool, error out=w609:errorcluster)  [unwired: 1 in]
                      n205 = case shown="No Error" w609 {
                        tunnel: w613 -> [w622 _]
                        tunnel: [w621 w623] -> w612
                        tunnel: w608 -> [w618 _]
                        tunnel: w607 -> [w616 _]
                        tunnel: w606 -> [_ w623]
                        tunnel: [TRUE _] -> w605
                        frame No Error {
                          n206 = Boolean To (0,1)(Boolean=w618) -> (0, 1=w617:i16)
                          n207 = Variant To Data(type=w616, Variant=w617) -> (data=w615:i64)  [unwired: 1 in, 1 out]
                          n208 = To Variant(anything=w615) -> (Variant=w619:variant)
                          n209 = Variant To Flattened String(Variant=w619) -> (data string=w620:string)  [unwired: 1 out]
                          n210 = Flattened String To Variant(6:w620, 7:w622) -> (3:w621:variant)  [unwired: 1 in, 1 out]
                        }
                        frame Error {
                        }
                      }
                    }
                    frame 48 {
                      # "STRING (0x30)"
                      n211 = Variant To Data(type="", Variant=w625) -> (data=w627:string, error out=w629:errorcluster)  [unwired: 1 in]
                      n212 = case shown="No Error" w629 {
                        tunnel: w632 -> [w640 _]
                        tunnel: [w639 w641] -> w630
                        tunnel: w628 -> [_ w641]
                        tunnel: w627 -> [w636 _]
                        tunnel: w626 -> [w634 _]
                        tunnel: [TRUE _] -> w624
                        frame No Error {
                          n213 = Fract/Exp String To Number(string=w636, default (0 dbl)=w634) -> (number=w635:i64)  [unwired: 2 in, 1 out]
                          n214 = To Variant(anything=w635) -> (Variant=w638:variant)
                          n215 = Variant To Flattened String(Variant=w638) -> (data string=w637:string)  [unwired: 1 out]
                          n216 = Flattened String To Variant(6:w637, 7:w640) -> (3:w639:variant)  [unwired: 1 in, 1 out]
                        }
                        frame Error {
                        }
                      }
                    }
                    frame 112 {
                      # "Refnum (0x70)"
                      n217 = Variant To Flattened String(Variant=w644) -> (data string=w643:string)  [unwired: 1 out]
                      n218 = Type Cast(type=w648, x=w643) -> (*(type *) &x=w647:i64)
                      n219 = To Variant(anything=w647) -> (Variant=w646:variant)
                      n220 = Variant To Flattened String(Variant=w646) -> (data string=w645:string)  [unwired: 1 out]
                      n221 = Flattened String To Variant(6:w645, 7:w650) -> (3:w649:variant)  [unwired: 1 in, 1 out]
                    }
                  }
                }
              }
            }
            frame 5 {
              # "U8 (0x05)"
              n222 = Variant To Flattened String(Variant=w657) -> (1:w661:i16[])  [unwired: 1 out]
              n223 = call "TypeDescriptor_GetType.vi"("type descriptor"=w661) -> ("Type"=w652:u8)  [unwired: 9 in, 1 out]
              n224 = Equal?(x=w653, y=w652) -> (x = y?=w655:bool)
              n225 = Compound Arithmetic op=OR(w655, invert w651) -> (w654:bool)
              n226 = case shown="True" w654 {
                tunnel: w660 -> [w662 w669]
                tunnel: [w662 w668] -> w659
                tunnel: w658 -> [_ w667]
                tunnel: w652 -> [_ w666]
                tunnel: w657 -> [_ w664]
                tunnel: [_ w663] -> w656
                frame False {
                }
                frame True {
                  w665 = u8 0  # U8
                  n227 = case shown="1..4, 6..8" w666 {
                    tunnel: w669 -> [w670 _ w680 w695 w710 w725 w737 w759 _]
                    tunnel: [w670 w672 w682 w697 w712 w727 w743 w761 w780] -> w668
                    tunnel: w667 -> [_ w673 w683 w698 w713 w728 w744 w763 w781]
                    tunnel: w665 -> [_ _ w678 w693 w708 w723 w738 w757 w779]
                    tunnel: w664 -> [_ w675 w677 w692 w707 w722 w742 w756 w775]
                    tunnel: [_ TRUE w676 w691 w706 w721 w736 w755 TRUE] -> w663
                    frame Default {
                      # "INCOMPATIBLE DATATYPES"
                    }
                    frame 5 {
                      # "U8 (0x05)"
                      n228 = Variant To Flattened String(Variant=w675) -> (data string=w674:string)  [unwired: 1 out]
                      n229 = Flattened String To Variant(6:w674, 7:w673) -> (3:w672:variant)  [unwired: 1 in, 1 out]
                    }
                    frame 1..4, 6..8 {
                      # "I8, I16, I32, I64, U16, U32, U64"
                      n230 = Variant To Data(type=w678, Variant=w677) -> (data=w679:u8, error out=w681:errorcluster)  [unwired: 1 in]
                      n231 = case shown="No Error" w681 {
                        tunnel: w683 -> [w689 _]
                        tunnel: [w688 w690] -> w682
                        tunnel: w680 -> [_ w690]
                        tunnel: w679 -> [w686 _]
                        tunnel: [TRUE _] -> w676
                        frame No Error {
                          n232 = To Variant(anything=w686) -> (Variant=w685:variant)
                          n233 = Variant To Flattened String(Variant=w685) -> (data string=w687:string)  [unwired: 1 out]
                          n234 = Flattened String To Variant(6:w687, 7:w689) -> (3:w688:variant)  [unwired: 1 in, 1 out]
                        }
                        frame Error {
                        }
                      }
                    }
                    frame 9..14 {
                      # "SGL, DBL, EXT, CSG, CDB, CXT (0x09 .. 0x0E)"
                      n235 = Variant To Data(type=w693, Variant=w692) -> (data=w694:u8, error out=w696:errorcluster)  [unwired: 1 in]
                      n236 = case shown="No Error" w696 {
                        tunnel: w698 -> [w704 _]
                        tunnel: [w703 w705] -> w697
                        tunnel: w695 -> [_ w705]
                        tunnel: w694 -> [w701 _]
                        tunnel: [TRUE _] -> w691
                        frame No Error {
                          n237 = To Variant(anything=w701) -> (Variant=w700:variant)
                          n238 = Variant To Flattened String(Variant=w700) -> (data string=w702:string)  [unwired: 1 out]
                          n239 = Flattened String To Variant(6:w702, 7:w704) -> (3:w703:variant)  [unwired: 1 in, 1 out]
                        }
                        frame Error {
                        }
                      }
                    }
                    frame 21..23 {
                      # "Enums (0x15 .. 0x17)"
                      n240 = Variant To Data(type=w708, Variant=w707) -> (data=w709:u8, error out=w711:errorcluster)  [unwired: 1 in]
                      n241 = case shown="No Error" w711 {
                        tunnel: w713 -> [w719 _]
                        tunnel: [w718 w720] -> w712
                        tunnel: w710 -> [_ w720]
                        tunnel: w709 -> [w716 _]
                        tunnel: [TRUE _] -> w706
                        frame No Error {
                          n242 = To Variant(anything=w716) -> (Variant=w715:variant)
                          n243 = Variant To Flattened String(Variant=w715) -> (data string=w717:string)  [unwired: 1 out]
                          n244 = Flattened String To Variant(6:w717, 7:w719) -> (3:w718:variant)  [unwired: 1 in, 1 out]
                        }
                        frame Error {
                        }
                      }
                    }
                    frame 25..30 {
                      # "Physical Units (0x19 .. 0x1E)"
                      n245 = Variant To Data(type=w723, Variant=w722) -> (data=w724:u8, error out=w726:errorcluster)  [unwired: 1 in]
                      n246 = case shown="No Error" w726 {
                        tunnel: w728 -> [w734 _]
                        tunnel: [w733 w735] -> w727
                        tunnel: w725 -> [_ w735]
                        tunnel: w724 -> [w731 _]
                        tunnel: [TRUE _] -> w721
                        frame No Error {
                          n247 = To Variant(anything=w731) -> (Variant=w730:variant)
                          n248 = Variant To Flattened String(Variant=w730) -> (data string=w732:string)  [unwired: 1 out]
                          n249 = Flattened String To Variant(6:w732, 7:w734) -> (3:w733:variant)  [unwired: 1 in, 1 out]
                        }
                        frame Error {
                        }
                      }
                    }
                    frame 33 {
                      # "Boolean (0x21)"
                      n250 = Variant To Data(type=FALSE, Variant=w742) -> (data=w739:bool, error out=w740:errorcluster)  [unwired: 1 in]
                      n251 = case shown="No Error" w740 {
                        tunnel: w744 -> [w753 _]
                        tunnel: [w752 w754] -> w743
                        tunnel: w739 -> [w749 _]
                        tunnel: w738 -> [w747 _]
                        tunnel: w737 -> [_ w754]
                        tunnel: [TRUE _] -> w736
                        frame No Error {
                          n252 = Boolean To (0,1)(Boolean=w749) -> (0, 1=w748:i16)
                          n253 = Variant To Data(type=w747, Variant=w748) -> (data=w746:u8)  [unwired: 1 in, 1 out]
                          n254 = To Variant(anything=w746) -> (Variant=w750:variant)
                          n255 = Variant To Flattened String(Variant=w750) -> (data string=w751:string)  [unwired: 1 out]
                          n256 = Flattened String To Variant(6:w751, 7:w753) -> (3:w752:variant)  [unwired: 1 in, 1 out]
                        }
                        frame Error {
                        }
                      }
                    }
                    frame 48 {
                      # "STRING (0x30)"
                      n257 = Variant To Data(type="", Variant=w756) -> (data=w758:string, error out=w760:errorcluster)  [unwired: 1 in]
                      n258 = case shown="No Error" w760 {
                        tunnel: w763 -> [w771 _]
                        tunnel: [w770 w772] -> w761
                        tunnel: w759 -> [_ w772]
                        tunnel: w758 -> [w767 _]
                        tunnel: w757 -> [w765 _]
                        tunnel: [TRUE _] -> w755
                        frame No Error {
                          n259 = Fract/Exp String To Number(string=w767, default (0 dbl)=w765) -> (number=w766:u8)  [unwired: 2 in, 1 out]
                          n260 = To Variant(anything=w766) -> (Variant=w769:variant)
                          n261 = Variant To Flattened String(Variant=w769) -> (data string=w768:string)  [unwired: 1 out]
                          n262 = Flattened String To Variant(6:w768, 7:w771) -> (3:w770:variant)  [unwired: 1 in, 1 out]
                        }
                        frame Error {
                        }
                      }
                    }
                    frame 112 {
                      # "Refnum (0x70)"
                      n263 = Variant To Flattened String(Variant=w775) -> (data string=w774:string)  [unwired: 1 out]
                      n264 = Type Cast(type=w779, x=w774) -> (*(type *) &x=w778:u8)
                      n265 = To Variant(anything=w778) -> (Variant=w777:variant)
                      n266 = Variant To Flattened String(Variant=w777) -> (data string=w776:string)  [unwired: 1 out]
                      n267 = Flattened String To Variant(6:w776, 7:w781) -> (3:w780:variant)  [unwired: 1 in, 1 out]
                    }
                  }
                }
              }
            }
            frame 6 {
              # "U16 (0x06)"
              n268 = Variant To Flattened String(Variant=w788) -> (1:w792:i16[])  [unwired: 1 out]
              n269 = call "TypeDescriptor_GetType.vi"("type descriptor"=w792) -> ("Type"=w782:u8)  [unwired: 9 in, 1 out]
              n270 = Equal?(x=w784, y=w782) -> (x = y?=w786:bool)
              n271 = Compound Arithmetic op=OR(w786, invert w783) -> (w785:bool)
              n272 = case shown="True" w785 {
                tunnel: w791 -> [w793 w800]
                tunnel: [w793 w799] -> w790
                tunnel: w789 -> [_ w798]
                tunnel: w782 -> [_ w797]
                tunnel: w788 -> [_ w795]
                tunnel: [_ w794] -> w787
                frame False {
                }
                frame True {
                  w796 = u16 0  # U16
                  n273 = case shown="1..5, 7, 8" w797 {
                    tunnel: w800 -> [w801 _ w811 w826 w841 w856 w868 w890 _]
                    tunnel: [w801 w803 w813 w828 w843 w858 w874 w892 w911] -> w799
                    tunnel: w798 -> [_ w804 w814 w829 w844 w859 w875 w894 w912]
                    tunnel: w796 -> [_ _ w809 w824 w839 w854 w869 w888 w910]
                    tunnel: w795 -> [_ w806 w808 w823 w838 w853 w873 w887 w906]
                    tunnel: [_ TRUE w807 w822 w837 w852 w867 w886 TRUE] -> w794
                    frame Default {
                      # "INCOMPATIBLE DATATYPES"
                    }
                    frame 6 {
                      # "U16 (0x06)"
                      n274 = Variant To Flattened String(Variant=w806) -> (data string=w805:string)  [unwired: 1 out]
                      n275 = Flattened String To Variant(6:w805, 7:w804) -> (3:w803:variant)  [unwired: 1 in, 1 out]
                    }
                    frame 1..5, 7, 8 {
                      # "I8, I16, I32, I64, U8, U32, U64"
                      n276 = Variant To Data(type=w809, Variant=w808) -> (data=w810:u16, error out=w812:errorcluster)  [unwired: 1 in]
                      n277 = case shown="No Error" w812 {
                        tunnel: w814 -> [w820 _]
                        tunnel: [w819 w821] -> w813
                        tunnel: w811 -> [_ w821]
                        tunnel: w810 -> [w817 _]
                        tunnel: [TRUE _] -> w807
                        frame No Error {
                          n278 = To Variant(anything=w817) -> (Variant=w816:variant)
                          n279 = Variant To Flattened String(Variant=w816) -> (data string=w818:string)  [unwired: 1 out]
                          n280 = Flattened String To Variant(6:w818, 7:w820) -> (3:w819:variant)  [unwired: 1 in, 1 out]
                        }
                        frame Error {
                        }
                      }
                    }
                    frame 9..14 {
                      # "SGL, DBL, EXT, CSG, CDB, CXT (0x09 .. 0x0E)"
                      n281 = Variant To Data(type=w824, Variant=w823) -> (data=w825:u16, error out=w827:errorcluster)  [unwired: 1 in]
                      n282 = case shown="No Error" w827 {
                        tunnel: w829 -> [w835 _]
                        tunnel: [w834 w836] -> w828
                        tunnel: w826 -> [_ w836]
                        tunnel: w825 -> [w832 _]
                        tunnel: [TRUE _] -> w822
                        frame No Error {
                          n283 = To Variant(anything=w832) -> (Variant=w831:variant)
                          n284 = Variant To Flattened String(Variant=w831) -> (data string=w833:string)  [unwired: 1 out]
                          n285 = Flattened String To Variant(6:w833, 7:w835) -> (3:w834:variant)  [unwired: 1 in, 1 out]
                        }
                        frame Error {
                        }
                      }
                    }
                    frame 21..23 {
                      # "Enums (0x15 .. 0x17)"
                      n286 = Variant To Data(type=w839, Variant=w838) -> (data=w840:u16, error out=w842:errorcluster)  [unwired: 1 in]
                      n287 = case shown="No Error" w842 {
                        tunnel: w844 -> [w850 _]
                        tunnel: [w849 w851] -> w843
                        tunnel: w841 -> [_ w851]
                        tunnel: w840 -> [w847 _]
                        tunnel: [TRUE _] -> w837
                        frame No Error {
                          n288 = To Variant(anything=w847) -> (Variant=w846:variant)
                          n289 = Variant To Flattened String(Variant=w846) -> (data string=w848:string)  [unwired: 1 out]
                          n290 = Flattened String To Variant(6:w848, 7:w850) -> (3:w849:variant)  [unwired: 1 in, 1 out]
                        }
                        frame Error {
                        }
                      }
                    }
                    frame 25..30 {
                      # "Physical Units (0x19 .. 0x1E)"
                      n291 = Variant To Data(type=w854, Variant=w853) -> (data=w855:u16, error out=w857:errorcluster)  [unwired: 1 in]
                      n292 = case shown="No Error" w857 {
                        tunnel: w859 -> [w865 _]
                        tunnel: [w864 w866] -> w858
                        tunnel: w856 -> [_ w866]
                        tunnel: w855 -> [w862 _]
                        tunnel: [TRUE _] -> w852
                        frame No Error {
                          n293 = To Variant(anything=w862) -> (Variant=w861:variant)
                          n294 = Variant To Flattened String(Variant=w861) -> (data string=w863:string)  [unwired: 1 out]
                          n295 = Flattened String To Variant(6:w863, 7:w865) -> (3:w864:variant)  [unwired: 1 in, 1 out]
                        }
                        frame Error {
                        }
                      }
                    }
                    frame 33 {
                      # "Boolean (0x21)"
                      n296 = Variant To Data(type=FALSE, Variant=w873) -> (data=w870:bool, error out=w871:errorcluster)  [unwired: 1 in]
                      n297 = case shown="No Error" w871 {
                        tunnel: w875 -> [w884 _]
                        tunnel: [w883 w885] -> w874
                        tunnel: w870 -> [w880 _]
                        tunnel: w869 -> [w878 _]
                        tunnel: w868 -> [_ w885]
                        tunnel: [TRUE _] -> w867
                        frame No Error {
                          n298 = Boolean To (0,1)(Boolean=w880) -> (0, 1=w879:i16)
                          n299 = Variant To Data(type=w878, Variant=w879) -> (data=w877:u16)  [unwired: 1 in, 1 out]
                          n300 = To Variant(anything=w877) -> (Variant=w881:variant)
                          n301 = Variant To Flattened String(Variant=w881) -> (data string=w882:string)  [unwired: 1 out]
                          n302 = Flattened String To Variant(6:w882, 7:w884) -> (3:w883:variant)  [unwired: 1 in, 1 out]
                        }
                        frame Error {
                        }
                      }
                    }
                    frame 48 {
                      # "STRING (0x30)"
                      n303 = Variant To Data(type="", Variant=w887) -> (data=w889:string, error out=w891:errorcluster)  [unwired: 1 in]
                      n304 = case shown="No Error" w891 {
                        tunnel: w894 -> [w902 _]
                        tunnel: [w901 w903] -> w892
                        tunnel: w890 -> [_ w903]
                        tunnel: w889 -> [w898 _]
                        tunnel: w888 -> [w896 _]
                        tunnel: [TRUE _] -> w886
                        frame No Error {
                          n305 = Fract/Exp String To Number(string=w898, default (0 dbl)=w896) -> (number=w897:u16)  [unwired: 2 in, 1 out]
                          n306 = To Variant(anything=w897) -> (Variant=w900:variant)
                          n307 = Variant To Flattened String(Variant=w900) -> (data string=w899:string)  [unwired: 1 out]
                          n308 = Flattened String To Variant(6:w899, 7:w902) -> (3:w901:variant)  [unwired: 1 in, 1 out]
                        }
                        frame Error {
                        }
                      }
                    }
                    frame 112 {
                      # "Refnum (0x70)"
                      n309 = Variant To Flattened String(Variant=w906) -> (data string=w905:string)  [unwired: 1 out]
                      n310 = Type Cast(type=w910, x=w905) -> (*(type *) &x=w909:u16)
                      n311 = To Variant(anything=w909) -> (Variant=w908:variant)
                      n312 = Variant To Flattened String(Variant=w908) -> (data string=w907:string)  [unwired: 1 out]
                      n313 = Flattened String To Variant(6:w907, 7:w912) -> (3:w911:variant)  [unwired: 1 in, 1 out]
                    }
                  }
                }
              }
            }
            frame 7 {
              # "U32 (0x07)"
              n314 = Variant To Flattened String(Variant=w919) -> (1:w923:i16[])  [unwired: 1 out]
              n315 = call "TypeDescriptor_GetType.vi"("type descriptor"=w923) -> ("Type"=w914:u8)  [unwired: 9 in, 1 out]
              n316 = Equal?(x=w915, y=w914) -> (x = y?=w917:bool)
              n317 = Compound Arithmetic op=OR(w917, invert w913) -> (w916:bool)
              n318 = case shown="True" w916 {
                tunnel: w922 -> [w924 w931]
                tunnel: [w924 w930] -> w921
                tunnel: w920 -> [_ w929]
                tunnel: w914 -> [_ w928]
                tunnel: w919 -> [_ w926]
                tunnel: [_ w925] -> w918
                frame False {
                }
                frame True {
                  w927 = u32 0  # U32
                  n319 = case shown="1..6, 8" w928 {
                    tunnel: w931 -> [w932 _ w942 w957 w972 w987 w999 w1021 _]
                    tunnel: [w932 w934 w944 w959 w974 w989 w1005 w1023 w1042] -> w930
                    tunnel: w929 -> [_ w935 w945 w960 w975 w990 w1006 w1025 w1043]
                    tunnel: w927 -> [_ _ w940 w955 w970 w985 w1000 w1019 w1041]
                    tunnel: w926 -> [_ w937 w939 w954 w969 w984 w1004 w1018 w1037]
                    tunnel: [_ TRUE w938 w953 w968 w983 w998 w1017 TRUE] -> w925
                    frame Default {
                      # "INCOMPATIBLE DATATYPES"
                    }
                    frame 7 {
                      # "U32 (0x07)"
                      n320 = Variant To Flattened String(Variant=w937) -> (data string=w936:string)  [unwired: 1 out]
                      n321 = Flattened String To Variant(6:w936, 7:w935) -> (3:w934:variant)  [unwired: 1 in, 1 out]
                    }
                    frame 1..6, 8 {
                      # "I8, I16, I32, I64, U8, U16, U64"
                      n322 = Variant To Data(type=w940, Variant=w939) -> (data=w941:u32, error out=w943:errorcluster)  [unwired: 1 in]
                      n323 = case shown="No Error" w943 {
                        tunnel: w945 -> [w951 _]
                        tunnel: [w950 w952] -> w944
                        tunnel: w942 -> [_ w952]
                        tunnel: w941 -> [w948 _]
                        tunnel: [TRUE _] -> w938
                        frame No Error {
                          n324 = To Variant(anything=w948) -> (Variant=w947:variant)
                          n325 = Variant To Flattened String(Variant=w947) -> (data string=w949:string)  [unwired: 1 out]
                          n326 = Flattened String To Variant(6:w949, 7:w951) -> (3:w950:variant)  [unwired: 1 in, 1 out]
                        }
                        frame Error {
                        }
                      }
                    }
                    frame 9..14 {
                      # "SGL, DBL, EXT, CSG, CDB, CXT (0x09 .. 0x0E)"
                      n327 = Variant To Data(type=w955, Variant=w954) -> (data=w956:u32, error out=w958:errorcluster)  [unwired: 1 in]
                      n328 = case shown="No Error" w958 {
                        tunnel: w960 -> [w966 _]
                        tunnel: [w965 w967] -> w959
                        tunnel: w957 -> [_ w967]
                        tunnel: w956 -> [w963 _]
                        tunnel: [TRUE _] -> w953
                        frame No Error {
                          n329 = To Variant(anything=w963) -> (Variant=w962:variant)
                          n330 = Variant To Flattened String(Variant=w962) -> (data string=w964:string)  [unwired: 1 out]
                          n331 = Flattened String To Variant(6:w964, 7:w966) -> (3:w965:variant)  [unwired: 1 in, 1 out]
                        }
                        frame Error {
                        }
                      }
                    }
                    frame 21..23 {
                      # "Enums (0x15 .. 0x17)"
                      n332 = Variant To Data(type=w970, Variant=w969) -> (data=w971:u32, error out=w973:errorcluster)  [unwired: 1 in]
                      n333 = case shown="No Error" w973 {
                        tunnel: w975 -> [w981 _]
                        tunnel: [w980 w982] -> w974
                        tunnel: w972 -> [_ w982]
                        tunnel: w971 -> [w978 _]
                        tunnel: [TRUE _] -> w968
                        frame No Error {
                          n334 = To Variant(anything=w978) -> (Variant=w977:variant)
                          n335 = Variant To Flattened String(Variant=w977) -> (data string=w979:string)  [unwired: 1 out]
                          n336 = Flattened String To Variant(6:w979, 7:w981) -> (3:w980:variant)  [unwired: 1 in, 1 out]
                        }
                        frame Error {
                        }
                      }
                    }
                    frame 25..30 {
                      # "Physical Units (0x19 .. 0x1E)"
                      n337 = Variant To Data(type=w985, Variant=w984) -> (data=w986:u32, error out=w988:errorcluster)  [unwired: 1 in]
                      n338 = case shown="No Error" w988 {
                        tunnel: w990 -> [w996 _]
                        tunnel: [w995 w997] -> w989
                        tunnel: w987 -> [_ w997]
                        tunnel: w986 -> [w993 _]
                        tunnel: [TRUE _] -> w983
                        frame No Error {
                          n339 = To Variant(anything=w993) -> (Variant=w992:variant)
                          n340 = Variant To Flattened String(Variant=w992) -> (data string=w994:string)  [unwired: 1 out]
                          n341 = Flattened String To Variant(6:w994, 7:w996) -> (3:w995:variant)  [unwired: 1 in, 1 out]
                        }
                        frame Error {
                        }
                      }
                    }
                    frame 33 {
                      # "Boolean (0x21)"
                      n342 = Variant To Data(type=FALSE, Variant=w1004) -> (data=w1001:bool, error out=w1002:errorcluster)  [unwired: 1 in]
                      n343 = case shown="No Error" w1002 {
                        tunnel: w1006 -> [w1015 _]
                        tunnel: [w1014 w1016] -> w1005
                        tunnel: w1001 -> [w1011 _]
                        tunnel: w1000 -> [w1009 _]
                        tunnel: w999 -> [_ w1016]
                        tunnel: [TRUE _] -> w998
                        frame No Error {
                          n344 = Boolean To (0,1)(Boolean=w1011) -> (0, 1=w1010:i16)
                          n345 = Variant To Data(type=w1009, Variant=w1010) -> (data=w1008:u32)  [unwired: 1 in, 1 out]
                          n346 = To Variant(anything=w1008) -> (Variant=w1012:variant)
                          n347 = Variant To Flattened String(Variant=w1012) -> (data string=w1013:string)  [unwired: 1 out]
                          n348 = Flattened String To Variant(6:w1013, 7:w1015) -> (3:w1014:variant)  [unwired: 1 in, 1 out]
                        }
                        frame Error {
                        }
                      }
                    }
                    frame 48 {
                      # "STRING (0x30)"
                      n349 = Variant To Data(type="", Variant=w1018) -> (data=w1020:string, error out=w1022:errorcluster)  [unwired: 1 in]
                      n350 = case shown="No Error" w1022 {
                        tunnel: w1025 -> [w1033 _]
                        tunnel: [w1032 w1034] -> w1023
                        tunnel: w1021 -> [_ w1034]
                        tunnel: w1020 -> [w1029 _]
                        tunnel: w1019 -> [w1027 _]
                        tunnel: [TRUE _] -> w1017
                        frame No Error {
                          n351 = Fract/Exp String To Number(string=w1029, default (0 dbl)=w1027) -> (number=w1028:u32)  [unwired: 2 in, 1 out]
                          n352 = To Variant(anything=w1028) -> (Variant=w1031:variant)
                          n353 = Variant To Flattened String(Variant=w1031) -> (data string=w1030:string)  [unwired: 1 out]
                          n354 = Flattened String To Variant(6:w1030, 7:w1033) -> (3:w1032:variant)  [unwired: 1 in, 1 out]
                        }
                        frame Error {
                        }
                      }
                    }
                    frame 112 {
                      # "Refnum (0x70)"
                      n355 = Variant To Flattened String(Variant=w1037) -> (data string=w1036:string)  [unwired: 1 out]
                      n356 = Type Cast(type=w1041, x=w1036) -> (*(type *) &x=w1040:u32)
                      n357 = To Variant(anything=w1040) -> (Variant=w1039:variant)
                      n358 = Variant To Flattened String(Variant=w1039) -> (data string=w1038:string)  [unwired: 1 out]
                      n359 = Flattened String To Variant(6:w1038, 7:w1043) -> (3:w1042:variant)  [unwired: 1 in, 1 out]
                    }
                  }
                }
              }
            }
            frame 8 {
              # "U64 (0x08)"
              n360 = Variant To Flattened String(Variant=w1050) -> (1:w1054:i16[])  [unwired: 1 out]
              n361 = call "TypeDescriptor_GetType.vi"("type descriptor"=w1054) -> ("Type"=w1044:u8)  [unwired: 9 in, 1 out]
              n362 = Equal?(x=w1046, y=w1044) -> (x = y?=w1048:bool)
              n363 = Compound Arithmetic op=OR(w1048, invert w1045) -> (w1047:bool)
              n364 = case shown="True" w1047 {
                tunnel: w1053 -> [w1055 w1062]
                tunnel: [w1055 w1061] -> w1052
                tunnel: w1051 -> [_ w1060]
                tunnel: w1044 -> [_ w1059]
                tunnel: w1050 -> [_ w1057]
                tunnel: [_ w1056] -> w1049
                frame False {
                }
                frame True {
                  w1058 = u64 0  # U64
                  n365 = case shown="1..7" w1059 {
                    tunnel: w1062 -> [w1063 _ w1073 w1088 w1103 w1118 w1130 w1152 _]
                    tunnel: [w1063 w1065 w1075 w1090 w1105 w1120 w1136 w1154 w1173] -> w1061
                    tunnel: w1060 -> [_ w1066 w1076 w1091 w1106 w1121 w1137 w1156 w1174]
                    tunnel: w1058 -> [_ _ w1071 w1086 w1101 w1116 w1131 w1150 w1172]
                    tunnel: w1057 -> [_ w1068 w1070 w1085 w1100 w1115 w1135 w1149 w1168]
                    tunnel: [_ TRUE w1069 w1084 w1099 w1114 w1129 w1148 TRUE] -> w1056
                    frame Default {
                      # "INCOMPATIBLE DATATYPES"
                    }
                    frame 8 {
                      # "U64 (0x08)"
                      n366 = Variant To Flattened String(Variant=w1068) -> (data string=w1067:string)  [unwired: 1 out]
                      n367 = Flattened String To Variant(6:w1067, 7:w1066) -> (3:w1065:variant)  [unwired: 1 in, 1 out]
                    }
                    frame 1..7 {
                      # "I8, I16, I32, I64, U8, U16, U32"
                      n368 = Variant To Data(type=w1071, Variant=w1070) -> (data=w1072:u64, error out=w1074:errorcluster)  [unwired: 1 in]
                      n369 = case shown="No Error" w1074 {
                        tunnel: w1076 -> [w1082 _]
                        tunnel: [w1081 w1083] -> w1075
                        tunnel: w1073 -> [_ w1083]
                        tunnel: w1072 -> [w1079 _]
                        tunnel: [TRUE _] -> w1069
                        frame No Error {
                          n370 = To Variant(anything=w1079) -> (Variant=w1078:variant)
                          n371 = Variant To Flattened String(Variant=w1078) -> (data string=w1080:string)  [unwired: 1 out]
                          n372 = Flattened String To Variant(6:w1080, 7:w1082) -> (3:w1081:variant)  [unwired: 1 in, 1 out]
                        }
                        frame Error {
                        }
                      }
                    }
                    frame 9..14 {
                      # "SGL, DBL, EXT, CSG, CDB, CXT (0x09 .. 0x0E)"
                      n373 = Variant To Data(type=w1086, Variant=w1085) -> (data=w1087:u64, error out=w1089:errorcluster)  [unwired: 1 in]
                      n374 = case shown="No Error" w1089 {
                        tunnel: w1091 -> [w1097 _]
                        tunnel: [w1096 w1098] -> w1090
                        tunnel: w1088 -> [_ w1098]
                        tunnel: w1087 -> [w1094 _]
                        tunnel: [TRUE _] -> w1084
                        frame No Error {
                          n375 = To Variant(anything=w1094) -> (Variant=w1093:variant)
                          n376 = Variant To Flattened String(Variant=w1093) -> (data string=w1095:string)  [unwired: 1 out]
                          n377 = Flattened String To Variant(6:w1095, 7:w1097) -> (3:w1096:variant)  [unwired: 1 in, 1 out]
                        }
                        frame Error {
                        }
                      }
                    }
                    frame 21..23 {
                      # "Enums (0x15 .. 0x17)"
                      n378 = Variant To Data(type=w1101, Variant=w1100) -> (data=w1102:u64, error out=w1104:errorcluster)  [unwired: 1 in]
                      n379 = case shown="No Error" w1104 {
                        tunnel: w1106 -> [w1112 _]
                        tunnel: [w1111 w1113] -> w1105
                        tunnel: w1103 -> [_ w1113]
                        tunnel: w1102 -> [w1109 _]
                        tunnel: [TRUE _] -> w1099
                        frame No Error {
                          n380 = To Variant(anything=w1109) -> (Variant=w1108:variant)
                          n381 = Variant To Flattened String(Variant=w1108) -> (data string=w1110:string)  [unwired: 1 out]
                          n382 = Flattened String To Variant(6:w1110, 7:w1112) -> (3:w1111:variant)  [unwired: 1 in, 1 out]
                        }
                        frame Error {
                        }
                      }
                    }
                    frame 25..30 {
                      # "Physical Units (0x19 .. 0x1E)"
                      n383 = Variant To Data(type=w1116, Variant=w1115) -> (data=w1117:u64, error out=w1119:errorcluster)  [unwired: 1 in]
                      n384 = case shown="No Error" w1119 {
                        tunnel: w1121 -> [w1127 _]
                        tunnel: [w1126 w1128] -> w1120
                        tunnel: w1118 -> [_ w1128]
                        tunnel: w1117 -> [w1124 _]
                        tunnel: [TRUE _] -> w1114
                        frame No Error {
                          n385 = To Variant(anything=w1124) -> (Variant=w1123:variant)
                          n386 = Variant To Flattened String(Variant=w1123) -> (data string=w1125:string)  [unwired: 1 out]
                          n387 = Flattened String To Variant(6:w1125, 7:w1127) -> (3:w1126:variant)  [unwired: 1 in, 1 out]
                        }
                        frame Error {
                        }
                      }
                    }
                    frame 33 {
                      # "Boolean (0x21)"
                      n388 = Variant To Data(type=FALSE, Variant=w1135) -> (data=w1132:bool, error out=w1133:errorcluster)  [unwired: 1 in]
                      n389 = case shown="No Error" w1133 {
                        tunnel: w1137 -> [w1146 _]
                        tunnel: [w1145 w1147] -> w1136
                        tunnel: w1132 -> [w1142 _]
                        tunnel: w1131 -> [w1140 _]
                        tunnel: w1130 -> [_ w1147]
                        tunnel: [TRUE _] -> w1129
                        frame No Error {
                          n390 = Boolean To (0,1)(Boolean=w1142) -> (0, 1=w1141:i16)
                          n391 = Variant To Data(type=w1140, Variant=w1141) -> (data=w1139:u64)  [unwired: 1 in, 1 out]
                          n392 = To Variant(anything=w1139) -> (Variant=w1143:variant)
                          n393 = Variant To Flattened String(Variant=w1143) -> (data string=w1144:string)  [unwired: 1 out]
                          n394 = Flattened String To Variant(6:w1144, 7:w1146) -> (3:w1145:variant)  [unwired: 1 in, 1 out]
                        }
                        frame Error {
                        }
                      }
                    }
                    frame 48 {
                      # "STRING (0x30)"
                      n395 = Variant To Data(type="", Variant=w1149) -> (data=w1151:string, error out=w1153:errorcluster)  [unwired: 1 in]
                      n396 = case shown="No Error" w1153 {
                        tunnel: w1156 -> [w1164 _]
                        tunnel: [w1163 w1165] -> w1154
                        tunnel: w1152 -> [_ w1165]
                        tunnel: w1151 -> [w1160 _]
                        tunnel: w1150 -> [w1158 _]
                        tunnel: [TRUE _] -> w1148
                        frame No Error {
                          n397 = Fract/Exp String To Number(string=w1160, default (0 dbl)=w1158) -> (number=w1159:u64)  [unwired: 2 in, 1 out]
                          n398 = To Variant(anything=w1159) -> (Variant=w1162:variant)
                          n399 = Variant To Flattened String(Variant=w1162) -> (data string=w1161:string)  [unwired: 1 out]
                          n400 = Flattened String To Variant(6:w1161, 7:w1164) -> (3:w1163:variant)  [unwired: 1 in, 1 out]
                        }
                        frame Error {
                        }
                      }
                    }
                    frame 112 {
                      # "Refnum (0x70)"
                      n401 = Variant To Flattened String(Variant=w1168) -> (data string=w1167:string)  [unwired: 1 out]
                      n402 = Type Cast(type=w1172, x=w1167) -> (*(type *) &x=w1171:u64)
                      n403 = To Variant(anything=w1171) -> (Variant=w1170:variant)
                      n404 = Variant To Flattened String(Variant=w1170) -> (data string=w1169:string)  [unwired: 1 out]
                      n405 = Flattened String To Variant(6:w1169, 7:w1174) -> (3:w1173:variant)  [unwired: 1 in, 1 out]
                    }
                  }
                }
              }
            }
            frame 9 {
              # "SGL (0x09)"
              n406 = Variant To Flattened String(Variant=w1181) -> (1:w1185:i16[])  [unwired: 1 out]
              n407 = call "TypeDescriptor_GetType.vi"("type descriptor"=w1185) -> ("Type"=w1175:u8)  [unwired: 9 in, 1 out]
              n408 = Equal?(x=w1176, y=w1175) -> (x = y?=w1179:bool)
              n409 = Compound Arithmetic op=OR(w1179, invert w1177) -> (w1178:bool)
              n410 = case shown="True" w1178 {
                tunnel: w1184 -> [w1186 w1193]
                tunnel: [w1186 w1192] -> w1183
                tunnel: w1182 -> [_ w1191]
                tunnel: w1175 -> [_ w1190]
                tunnel: w1181 -> [_ w1188]
                tunnel: [_ w1187] -> w1180
                frame False {
                }
                frame True {
                  w1189 = sgl 0.0  # SGL
                  n411 = case shown="30" w1190 {
                    tunnel: w1193 -> [w1194 _ w1204 w1219 w1234 w1249]
                    tunnel: [w1194 w1195 w1206 w1221 w1236 w1251] -> w1192
                    tunnel: w1191 -> [_ w1197 w1207 w1222 w1237 w1253]
                    tunnel: w1189 -> [_ _ w1202 w1217 w1232 w1247]
                    tunnel: w1188 -> [_ w1199 w1201 w1216 w1231 w1246]
                    tunnel: [_ TRUE w1200 w1215 w1230 w1245] -> w1187
                    frame Default {
                      # "INCOMPATIBLE DATATYPES"
                    }
                    frame 9 {
                      # "SGL (0x09)"
                      n412 = Variant To Flattened String(Variant=w1199) -> (data string=w1198:string)  [unwired: 1 out]
                      n413 = Flattened String To Variant(6:w1198, 7:w1197) -> (3:w1195:variant)  [unwired: 1 in, 1 out]
                    }
                    frame 1..8 {
                      # "I8, I16, I32, I64, U8, U16, U32, U64"
                      n414 = Variant To Data(type=w1202, Variant=w1201) -> (data=w1203:sgl, error out=w1205:errorcluster)  [unwired: 1 in]
                      n415 = case shown="No Error" w1205 {
                        tunnel: w1207 -> [w1213 _]
                        tunnel: [w1212 w1214] -> w1206
                        tunnel: w1204 -> [_ w1214]
                        tunnel: w1203 -> [w1210 _]
                        tunnel: [TRUE _] -> w1200
                        frame No Error {
                          n416 = To Variant(anything=w1210) -> (Variant=w1209:variant)
                          n417 = Variant To Flattened String(Variant=w1209) -> (data string=w1211:string)  [unwired: 1 out]
                          n418 = Flattened String To Variant(6:w1211, 7:w1213) -> (3:w1212:variant)  [unwired: 1 in, 1 out]
                        }
                        frame Error {
                        }
                      }
                    }
                    frame 10..14 {
                      # "DBL, EXT, CSG, CDB, CXT (0x10 .. 0x0E)"
                      n419 = Variant To Data(type=w1217, Variant=w1216) -> (data=w1218:sgl, error out=w1220:errorcluster)  [unwired: 1 in]
                      n420 = case shown="No Error" w1220 {
                        tunnel: w1222 -> [w1228 _]
                        tunnel: [w1227 w1229] -> w1221
                        tunnel: w1219 -> [_ w1229]
                        tunnel: w1218 -> [w1225 _]
                        tunnel: [TRUE _] -> w1215
                        frame No Error {
                          n421 = To Variant(anything=w1225) -> (Variant=w1224:variant)
                          n422 = Variant To Flattened String(Variant=w1224) -> (data string=w1226:string)  [unwired: 1 out]
                          n423 = Flattened String To Variant(6:w1226, 7:w1228) -> (3:w1227:variant)  [unwired: 1 in, 1 out]
                        }
                        frame Error {
                        }
                      }
                    }
                    frame 25..30 {
                      # "Physical Units (0x19 .. 0x1E)"
                      n424 = Variant To Data(type=w1232, Variant=w1231) -> (data=w1233:sgl, error out=w1235:errorcluster)  [unwired: 1 in]
                      n425 = case shown="No Error" w1235 {
                        tunnel: w1237 -> [w1243 _]
                        tunnel: [w1242 w1244] -> w1236
                        tunnel: w1234 -> [_ w1244]
                        tunnel: w1233 -> [w1240 _]
                        tunnel: [TRUE _] -> w1230
                        frame No Error {
                          n426 = To Variant(anything=w1240) -> (Variant=w1239:variant)
                          n427 = Variant To Flattened String(Variant=w1239) -> (data string=w1241:string)  [unwired: 1 out]
                          n428 = Flattened String To Variant(6:w1241, 7:w1243) -> (3:w1242:variant)  [unwired: 1 in, 1 out]
                        }
                        frame Error {
                        }
                      }
                    }
                    frame 48 {
                      # "STRING (0x30)"
                      n429 = Variant To Data(type="", Variant=w1246) -> (data=w1248:string, error out=w1250:errorcluster)  [unwired: 1 in]
                      n430 = case shown="No Error" w1250 {
                        tunnel: w1253 -> [w1260 _]
                        tunnel: [w1259 w1261] -> w1251
                        tunnel: w1249 -> [_ w1261]
                        tunnel: w1248 -> [w1255 _]
                        tunnel: w1247 -> [_ _]
                        tunnel: [TRUE _] -> w1245
                        frame No Error {
                          n431 = call "String to SingleFloat (Scalar).vi"("Value (String)"=w1255) -> ("Value (Single)"=w1254:sgl)  [unwired: 8 in, 2 out]
                          n432 = To Variant(anything=w1254) -> (Variant=w1258:variant)
                          n433 = Variant To Flattened String(Variant=w1258) -> (data string=w1257:string)  [unwired: 1 out]
                          n434 = Flattened String To Variant(6:w1257, 7:w1260) -> (3:w1259:variant)  [unwired: 1 in, 1 out]
                        }
                        frame Error {
                        }
                      }
                    }
                  }
                }
              }
            }
            frame 10 {
              # "DBL (0xA)"
              n435 = Variant To Flattened String(Variant=w1268) -> (1:w1272:i16[])  [unwired: 1 out]
              n436 = call "TypeDescriptor_GetType.vi"("type descriptor"=w1272) -> ("Type"=w1262:u8)  [unwired: 9 in, 1 out]
              n437 = Equal?(x=w1263, y=w1262) -> (x = y?=w1266:bool)
              n438 = Compound Arithmetic op=OR(w1266, invert w1264) -> (w1265:bool)
              n439 = case shown="True" w1265 {
                tunnel: w1271 -> [w1273 w1280]
                tunnel: [w1273 w1279] -> w1270
                tunnel: w1269 -> [_ w1278]
                tunnel: w1262 -> [_ w1277]
                tunnel: w1268 -> [_ w1275]
                tunnel: [_ w1274] -> w1267
                frame False {
                }
                frame True {
                  w1276 = 0.0  # DBL
                  n440 = case shown="1..8" w1277 {
                    tunnel: w1280 -> [w1281 _ w1291 w1306 w1321 w1335]
                    tunnel: [w1281 w1283 w1293 w1308 w1323 w1337] -> w1279
                    tunnel: w1278 -> [_ w1284 w1294 w1309 w1324 w1339]
                    tunnel: w1276 -> [_ _ w1289 w1304 w1319 _]
                    tunnel: w1275 -> [_ w1286 w1288 w1303 w1318 w1333]
                    tunnel: [_ TRUE w1287 w1302 w1317 w1332] -> w1274
                    frame Default {
                      # "INCOMPATIBLE DATATYPES"
                    }
                    frame 10 {
                      # "DBL (0x0A)"
                      n441 = Variant To Flattened String(Variant=w1286) -> (data string=w1285:string)  [unwired: 1 out]
                      n442 = Flattened String To Variant(6:w1285, 7:w1284) -> (3:w1283:variant)  [unwired: 1 in, 1 out]
                    }
                    frame 1..8 {
                      # "I8, I16, I32, I64, U8, U16, U32, U64"
                      n443 = Variant To Data(type=w1289, Variant=w1288) -> (data=w1290:dbl, error out=w1292:errorcluster)  [unwired: 1 in]
                      n444 = case shown="No Error" w1292 {
                        tunnel: w1294 -> [w1300 _]
                        tunnel: [w1299 w1301] -> w1293
                        tunnel: w1291 -> [_ w1301]
                        tunnel: w1290 -> [w1297 _]
                        tunnel: [TRUE _] -> w1287
                        frame No Error {
                          n445 = To Variant(anything=w1297) -> (Variant=w1296:variant)
                          n446 = Variant To Flattened String(Variant=w1296) -> (data string=w1298:string)  [unwired: 1 out]
                          n447 = Flattened String To Variant(6:w1298, 7:w1300) -> (3:w1299:variant)  [unwired: 1 in, 1 out]
                        }
                        frame Error {
                        }
                      }
                    }
                    frame 9, 11..14 {
                      # "SGL, EXT, CSG, CDB, CXT (0x09 .. 0x0E)"
                      n448 = Variant To Data(type=w1304, Variant=w1303) -> (data=w1305:dbl, error out=w1307:errorcluster)  [unwired: 1 in]
                      n449 = case shown="No Error" w1307 {
                        tunnel: w1309 -> [w1315 _]
                        tunnel: [w1314 w1316] -> w1308
                        tunnel: w1306 -> [_ w1316]
                        tunnel: w1305 -> [w1312 _]
                        tunnel: [TRUE _] -> w1302
                        frame No Error {
                          n450 = To Variant(anything=w1312) -> (Variant=w1311:variant)
                          n451 = Variant To Flattened String(Variant=w1311) -> (data string=w1313:string)  [unwired: 1 out]
                          n452 = Flattened String To Variant(6:w1313, 7:w1315) -> (3:w1314:variant)  [unwired: 1 in, 1 out]
                        }
                        frame Error {
                        }
                      }
                    }
                    frame 25..30 {
                      # "Physical Units (0x19 .. 0x1E)"
                      n453 = Variant To Data(type=w1319, Variant=w1318) -> (data=w1320:dbl, error out=w1322:errorcluster)  [unwired: 1 in]
                      n454 = case shown="No Error" w1322 {
                        tunnel: w1324 -> [w1330 _]
                        tunnel: [w1329 w1331] -> w1323
                        tunnel: w1321 -> [_ w1331]
                        tunnel: w1320 -> [w1327 _]
                        tunnel: [TRUE _] -> w1317
                        frame No Error {
                          n455 = To Variant(anything=w1327) -> (Variant=w1326:variant)
                          n456 = Variant To Flattened String(Variant=w1326) -> (data string=w1328:string)  [unwired: 1 out]
                          n457 = Flattened String To Variant(6:w1328, 7:w1330) -> (3:w1329:variant)  [unwired: 1 in, 1 out]
                        }
                        frame Error {
                        }
                      }
                    }
                    frame 48 {
                      # "STRING (0x30)"
                      n458 = Variant To Data(type="", Variant=w1333) -> (data=w1334:string, error out=w1336:errorcluster)  [unwired: 1 in]
                      n459 = case shown="No Error" w1336 {
                        tunnel: w1339 -> [w1346 _]
                        tunnel: [w1345 w1347] -> w1337
                        tunnel: w1335 -> [_ w1347]
                        tunnel: w1334 -> [w1341 _]
                        tunnel: [TRUE _] -> w1332
                        frame No Error {
                          n460 = call "String to DoubleFloat (Scalar).vi"("Value (String)"=w1341) -> ("Value (Double)"=w1340:dbl)  [unwired: 8 in, 2 out]
                          n461 = To Variant(anything=w1340) -> (Variant=w1344:variant)
                          n462 = Variant To Flattened String(Variant=w1344) -> (data string=w1343:string)  [unwired: 1 out]
                          n463 = Flattened String To Variant(6:w1343, 7:w1346) -> (3:w1345:variant)  [unwired: 1 in, 1 out]
                        }
                        frame Error {
                        }
                      }
                    }
                  }
                }
              }
            }
            frame 11 {
              # "EXT (0x0B)"
              n464 = Variant To Flattened String(Variant=w1354) -> (1:w1358:i16[])  [unwired: 1 out]
              n465 = call "TypeDescriptor_GetType.vi"("type descriptor"=w1358) -> ("Type"=w1349:u8)  [unwired: 9 in, 1 out]
              n466 = Equal?(x=w1350, y=w1349) -> (x = y?=w1352:bool)
              n467 = Compound Arithmetic op=OR(w1352, invert w1348) -> (w1351:bool)
              n468 = case shown="True" w1351 {
                tunnel: w1357 -> [w1359 w1366]
                tunnel: [w1359 w1365] -> w1356
                tunnel: w1355 -> [_ w1364]
                tunnel: w1349 -> [_ w1363]
                tunnel: w1354 -> [_ w1361]
                tunnel: [_ w1360] -> w1353
                frame False {
                }
                frame True {
                  w1362 = ext 0.0  # EXT
                  n469 = case shown="30" w1363 {
                    tunnel: w1366 -> [w1367 _ w1377 w1392 w1407 w1422]
                    tunnel: [w1367 w1368 w1379 w1394 w1409 w1424] -> w1365
                    tunnel: w1364 -> [_ w1370 w1380 w1395 w1410 w1426]
                    tunnel: w1362 -> [_ _ w1375 w1390 w1405 w1420]
                    tunnel: w1361 -> [_ w1372 w1374 w1389 w1404 w1419]
                    tunnel: [_ TRUE w1373 w1388 w1403 w1418] -> w1360
                    frame Default {
                      # "INCOMPATIBLE DATATYPES"
                    }
                    frame 11 {
                      # "EXT (0x0B)"
                      n470 = Variant To Flattened String(Variant=w1372) -> (data string=w1371:string)  [unwired: 1 out]
                      n471 = Flattened String To Variant(6:w1371, 7:w1370) -> (3:w1368:variant)  [unwired: 1 in, 1 out]
                    }
                    frame 1..8 {
                      # "I8, I16, I32, I64, U8, U16, U32, U64"
                      n472 = Variant To Data(type=w1375, Variant=w1374) -> (data=w1376:ext, error out=w1378:errorcluster)  [unwired: 1 in]
                      n473 = case shown="No Error" w1378 {
                        tunnel: w1380 -> [w1386 _]
                        tunnel: [w1385 w1387] -> w1379
                        tunnel: w1377 -> [_ w1387]
                        tunnel: w1376 -> [w1383 _]
                        tunnel: [TRUE _] -> w1373
                        frame No Error {
                          n474 = To Variant(anything=w1383) -> (Variant=w1382:variant)
                          n475 = Variant To Flattened String(Variant=w1382) -> (data string=w1384:string)  [unwired: 1 out]
                          n476 = Flattened String To Variant(6:w1384, 7:w1386) -> (3:w1385:variant)  [unwired: 1 in, 1 out]
                        }
                        frame Error {
                        }
                      }
                    }
                    frame 9, 10, 12..14 {
                      # "SGL, DBL, CSG, CDB, CXT (0x09 .. 0x0E)"
                      n477 = Variant To Data(type=w1390, Variant=w1389) -> (data=w1391:ext, error out=w1393:errorcluster)  [unwired: 1 in]
                      n478 = case shown="No Error" w1393 {
                        tunnel: w1395 -> [w1401 _]
                        tunnel: [w1400 w1402] -> w1394
                        tunnel: w1392 -> [_ w1402]
                        tunnel: w1391 -> [w1398 _]
                        tunnel: [TRUE _] -> w1388
                        frame No Error {
                          n479 = To Variant(anything=w1398) -> (Variant=w1397:variant)
                          n480 = Variant To Flattened String(Variant=w1397) -> (data string=w1399:string)  [unwired: 1 out]
                          n481 = Flattened String To Variant(6:w1399, 7:w1401) -> (3:w1400:variant)  [unwired: 1 in, 1 out]
                        }
                        frame Error {
                        }
                      }
                    }
                    frame 25..30 {
                      # "Physical Units (0x19 .. 0x1E)"
                      n482 = Variant To Data(type=w1405, Variant=w1404) -> (data=w1406:ext, error out=w1408:errorcluster)  [unwired: 1 in]
                      n483 = case shown="No Error" w1408 {
                        tunnel: w1410 -> [w1416 _]
                        tunnel: [w1415 w1417] -> w1409
                        tunnel: w1407 -> [_ w1417]
                        tunnel: w1406 -> [w1413 _]
                        tunnel: [TRUE _] -> w1403
                        frame No Error {
                          n484 = To Variant(anything=w1413) -> (Variant=w1412:variant)
                          n485 = Variant To Flattened String(Variant=w1412) -> (data string=w1414:string)  [unwired: 1 out]
                          n486 = Flattened String To Variant(6:w1414, 7:w1416) -> (3:w1415:variant)  [unwired: 1 in, 1 out]
                        }
                        frame Error {
                        }
                      }
                    }
                    frame 48 {
                      # "STRING (0x30)"
                      n487 = Variant To Data(type="", Variant=w1419) -> (data=w1421:string, error out=w1423:errorcluster)  [unwired: 1 in]
                      n488 = case shown="No Error" w1423 {
                        tunnel: w1426 -> [w1433 _]
                        tunnel: [w1432 w1434] -> w1424
                        tunnel: w1422 -> [_ w1434]
                        tunnel: w1421 -> [w1428 _]
                        tunnel: w1420 -> [_ _]
                        tunnel: [TRUE _] -> w1418
                        frame No Error {
                          n489 = call "String to ExtendedFloat (Scalar).vi"("Value (String)"=w1428) -> ("Value (Extended)"=w1427:ext)  [unwired: 8 in, 2 out]
                          n490 = To Variant(anything=w1427) -> (Variant=w1431:variant)
                          n491 = Variant To Flattened String(Variant=w1431) -> (data string=w1430:string)  [unwired: 1 out]
                          n492 = Flattened String To Variant(6:w1430, 7:w1433) -> (3:w1432:variant)  [unwired: 1 in, 1 out]
                        }
                        frame Error {
                        }
                      }
                    }
                  }
                }
              }
            }
            frame 12 {
              # "CSG (0x0C)"
              n493 = Variant To Flattened String(Variant=w1441) -> (1:w1445:i16[])  [unwired: 1 out]
              n494 = call "TypeDescriptor_GetType.vi"("type descriptor"=w1445) -> ("Type"=w1436:u8)  [unwired: 9 in, 1 out]
              n495 = Equal?(x=w1437, y=w1436) -> (x = y?=w1439:bool)
              n496 = Compound Arithmetic op=OR(w1439, invert w1435) -> (w1438:bool)
              n497 = case shown="True" w1438 {
                tunnel: w1444 -> [w1446 w1453]
                tunnel: [w1446 w1452] -> w1443
                tunnel: w1442 -> [_ w1451]
                tunnel: w1436 -> [_ w1450]
                tunnel: w1441 -> [_ w1448]
                tunnel: [_ w1447] -> w1440
                frame False {
                }
                frame True {
                  w1449 = csg 0.0+0.0i  # CSG
                  n498 = case shown="30" w1450 {
                    tunnel: w1453 -> [w1454 _ w1464 w1479 w1494 w1509]
                    tunnel: [w1454 w1455 w1466 w1481 w1496 w1511] -> w1452
                    tunnel: w1451 -> [_ w1457 w1467 w1482 w1497 w1512]
                    tunnel: w1449 -> [_ _ w1462 w1477 w1492 _]
                    tunnel: w1448 -> [_ w1459 w1461 w1476 w1491 w1507]
                    tunnel: [_ TRUE w1460 w1475 w1490 w1506] -> w1447
                    frame Default {
                      # "INCOMPATIBLE DATATYPES"
                    }
                    frame 12 {
                      # "CSG (0x0C)"
                      n499 = Variant To Flattened String(Variant=w1459) -> (data string=w1458:string)  [unwired: 1 out]
                      n500 = Flattened String To Variant(6:w1458, 7:w1457) -> (3:w1455:variant)  [unwired: 1 in, 1 out]
                    }
                    frame 1..8 {
                      # "I8, I16, I32, I64, U8, U16, U32, U64"
                      n501 = Variant To Data(type=w1462, Variant=w1461) -> (data=w1463:csg, error out=w1465:errorcluster)  [unwired: 1 in]
                      n502 = case shown="No Error" w1465 {
                        tunnel: w1467 -> [w1473 _]
                        tunnel: [w1472 w1474] -> w1466
                        tunnel: w1464 -> [_ w1474]
                        tunnel: w1463 -> [w1470 _]
                        tunnel: [TRUE _] -> w1460
                        frame No Error {
                          n503 = To Variant(anything=w1470) -> (Variant=w1469:variant)
                          n504 = Variant To Flattened String(Variant=w1469) -> (data string=w1471:string)  [unwired: 1 out]
                          n505 = Flattened String To Variant(6:w1471, 7:w1473) -> (3:w1472:variant)  [unwired: 1 in, 1 out]
                        }
                        frame Error {
                        }
                      }
                    }
                    frame 9..11, 13, 14 {
                      # "SGL, DBL, EXT, CDB, CXT (0x09 .. 0x0E)"
                      n506 = Variant To Data(type=w1477, Variant=w1476) -> (data=w1478:csg, error out=w1480:errorcluster)  [unwired: 1 in]
                      n507 = case shown="No Error" w1480 {
                        tunnel: w1482 -> [w1488 _]
                        tunnel: [w1487 w1489] -> w1481
                        tunnel: w1479 -> [_ w1489]
                        tunnel: w1478 -> [w1485 _]
                        tunnel: [TRUE _] -> w1475
                        frame No Error {
                          n508 = To Variant(anything=w1485) -> (Variant=w1484:variant)
                          n509 = Variant To Flattened String(Variant=w1484) -> (data string=w1486:string)  [unwired: 1 out]
                          n510 = Flattened String To Variant(6:w1486, 7:w1488) -> (3:w1487:variant)  [unwired: 1 in, 1 out]
                        }
                        frame Error {
                        }
                      }
                    }
                    frame 25..30 {
                      # "Physical Units (0x19 .. 0x1E)"
                      n511 = Variant To Data(type=w1492, Variant=w1491) -> (data=w1493:csg, error out=w1495:errorcluster)  [unwired: 1 in]
                      n512 = case shown="No Error" w1495 {
                        tunnel: w1497 -> [w1503 _]
                        tunnel: [w1502 w1504] -> w1496
                        tunnel: w1494 -> [_ w1504]
                        tunnel: w1493 -> [w1500 _]
                        tunnel: [TRUE _] -> w1490
                        frame No Error {
                          n513 = To Variant(anything=w1500) -> (Variant=w1499:variant)
                          n514 = Variant To Flattened String(Variant=w1499) -> (data string=w1501:string)  [unwired: 1 out]
                          n515 = Flattened String To Variant(6:w1501, 7:w1503) -> (3:w1502:variant)  [unwired: 1 in, 1 out]
                        }
                        frame Error {
                        }
                      }
                    }
                    frame 48 {
                      # "String (0x30)"
                      n516 = Variant To Data(type="", Variant=w1507) -> (data=w1508:string, error out=w1510:errorcluster)  [unwired: 1 in]
                      n517 = case shown="No Error" w1510 {
                        tunnel: w1512 -> [w1519 _]
                        tunnel: [w1518 w1520] -> w1511
                        tunnel: w1509 -> [_ w1520]
                        tunnel: w1508 -> [w1514 _]
                        tunnel: [TRUE _] -> w1506
                        frame No Error {
                          n518 = call "String to SingleComplex (Scalar).vi"("Value (String)"=w1514) -> ("Value (CSG)"=w1513:csg)  [unwired: 8 in, 2 out]
                          n519 = To Variant(anything=w1513) -> (Variant=w1516:variant)
                          n520 = Variant To Flattened String(Variant=w1516) -> (data string=w1517:string)  [unwired: 1 out]
                          n521 = Flattened String To Variant(6:w1517, 7:w1519) -> (3:w1518:variant)  [unwired: 1 in, 1 out]
                        }
                        frame Error {
                        }
                      }
                    }
                  }
                }
              }
            }
            frame 13 {
              # "CDB (0x0D)"
              n522 = Variant To Flattened String(Variant=w1528) -> (1:w1531:i16[])  [unwired: 1 out]
              n523 = call "TypeDescriptor_GetType.vi"("type descriptor"=w1531) -> ("Type"=w1521:u8)  [unwired: 9 in, 1 out]
              n524 = Equal?(x=w1523, y=w1521) -> (x = y?=w1525:bool)
              n525 = Compound Arithmetic op=OR(w1525, invert w1522) -> (w1524:bool)
              n526 = case shown="True" w1524 {
                tunnel: [w1532 w1538] -> w1530
                tunnel: w1529 -> [_ w1537]
                tunnel: w1521 -> [_ w1536]
                tunnel: w1528 -> [_ w1534]
                tunnel: [_ w1533] -> w1527
                tunnel: w1526 -> [w1532 w1539]
                frame False {
                }
                frame True {
                  w1535 = cdb 0.0+0.0i  # CDB
                  n527 = case shown="30" w1536 {
                    tunnel: w1539 -> [w1540 _ w1550 w1565 w1580 w1595]
                    tunnel: [w1540 w1541 w1552 w1567 w1582 w1597] -> w1538
                    tunnel: w1537 -> [_ w1543 w1553 w1568 w1583 w1598]
                    tunnel: w1535 -> [_ _ w1548 w1563 w1578 _]
                    tunnel: w1534 -> [_ w1545 w1547 w1562 w1577 w1593]
                    tunnel: [_ TRUE w1546 w1561 w1576 w1592] -> w1533
                    frame Default {
                      # "INCOMPATIBLE DATATYPES"
                    }
                    frame 13 {
                      # "CDB (0x0D)"
                      n528 = Variant To Flattened String(Variant=w1545) -> (data string=w1544:string)  [unwired: 1 out]
                      n529 = Flattened String To Variant(6:w1544, 7:w1543) -> (3:w1541:variant)  [unwired: 1 in, 1 out]
                    }
                    frame 1..8 {
                      # "I8, I16, I32, I64, U8, U16, U32, U64"
                      n530 = Variant To Data(type=w1548, Variant=w1547) -> (data=w1549:cdb, error out=w1551:errorcluster)  [unwired: 1 in]
                      n531 = case shown="No Error" w1551 {
                        tunnel: w1553 -> [w1559 _]
                        tunnel: [w1558 w1560] -> w1552
                        tunnel: w1550 -> [_ w1560]
                        tunnel: w1549 -> [w1556 _]
                        tunnel: [TRUE _] -> w1546
                        frame No Error {
                          n532 = To Variant(anything=w1556) -> (Variant=w1555:variant)
                          n533 = Variant To Flattened String(Variant=w1555) -> (data string=w1557:string)  [unwired: 1 out]
                          n534 = Flattened String To Variant(6:w1557, 7:w1559) -> (3:w1558:variant)  [unwired: 1 in, 1 out]
                        }
                        frame Error {
                        }
                      }
                    }
                    frame 9..12, 14 {
                      # "SGL, DBL, EXT, CSG, CXT (0x09 .. 0x0E)"
                      n535 = Variant To Data(type=w1563, Variant=w1562) -> (data=w1564:cdb, error out=w1566:errorcluster)  [unwired: 1 in]
                      n536 = case shown="No Error" w1566 {
                        tunnel: w1568 -> [w1574 _]
                        tunnel: [w1573 w1575] -> w1567
                        tunnel: w1565 -> [_ w1575]
                        tunnel: w1564 -> [w1571 _]
                        tunnel: [TRUE _] -> w1561
                        frame No Error {
                          n537 = To Variant(anything=w1571) -> (Variant=w1570:variant)
                          n538 = Variant To Flattened String(Variant=w1570) -> (data string=w1572:string)  [unwired: 1 out]
                          n539 = Flattened String To Variant(6:w1572, 7:w1574) -> (3:w1573:variant)  [unwired: 1 in, 1 out]
                        }
                        frame Error {
                        }
                      }
                    }
                    frame 25..30 {
                      # "Physical Units (0x19 .. 0x1E)"
                      n540 = Variant To Data(type=w1578, Variant=w1577) -> (data=w1579:cdb, error out=w1581:errorcluster)  [unwired: 1 in]
                      n541 = case shown="No Error" w1581 {
                        tunnel: w1583 -> [w1589 _]
                        tunnel: [w1588 w1590] -> w1582
                        tunnel: w1580 -> [_ w1590]
                        tunnel: w1579 -> [w1586 _]
                        tunnel: [TRUE _] -> w1576
                        frame No Error {
                          n542 = To Variant(anything=w1586) -> (Variant=w1585:variant)
                          n543 = Variant To Flattened String(Variant=w1585) -> (data string=w1587:string)  [unwired: 1 out]
                          n544 = Flattened String To Variant(6:w1587, 7:w1589) -> (3:w1588:variant)  [unwired: 1 in, 1 out]
                        }
                        frame Error {
                        }
                      }
                    }
                    frame 48 {
                      # "String (0x30)"
                      n545 = Variant To Data(type="", Variant=w1593) -> (data=w1594:string, error out=w1596:errorcluster)  [unwired: 1 in]
                      n546 = case shown="No Error" w1596 {
                        tunnel: w1598 -> [w1605 _]
                        tunnel: [w1604 w1606] -> w1597
                        tunnel: w1595 -> [_ w1606]
                        tunnel: w1594 -> [w1600 _]
                        tunnel: [TRUE _] -> w1592
                        frame No Error {
                          n547 = call "String to DoubleComplex (Scalar).vi"("Value (String)"=w1600) -> ("Value (CDB)"=w1599:cdb)  [unwired: 8 in, 2 out]
                          n548 = To Variant(anything=w1599) -> (Variant=w1602:variant)
                          n549 = Variant To Flattened String(Variant=w1602) -> (data string=w1603:string)  [unwired: 1 out]
                          n550 = Flattened String To Variant(6:w1603, 7:w1605) -> (3:w1604:variant)  [unwired: 1 in, 1 out]
                        }
                        frame Error {
                        }
                      }
                    }
                  }
                }
              }
            }
            frame 14 {
              # "CXT (0x0E)"
              n551 = Variant To Flattened String(Variant=w1613) -> (1:w1617:i16[])  [unwired: 1 out]
              n552 = call "TypeDescriptor_GetType.vi"("type descriptor"=w1617) -> ("Type"=w1607:u8)  [unwired: 9 in, 1 out]
              n553 = Equal?(x=w1608, y=w1607) -> (x = y?=w1611:bool)
              n554 = Compound Arithmetic op=OR(w1611, invert w1609) -> (w1610:bool)
              n555 = case shown="True" w1610 {
                tunnel: w1616 -> [w1618 w1625]
                tunnel: [w1618 w1624] -> w1615
                tunnel: w1614 -> [_ w1623]
                tunnel: w1607 -> [_ w1622]
                tunnel: w1613 -> [_ w1620]
                tunnel: [_ w1619] -> w1612
                frame False {
                }
                frame True {
                  w1621 = cxt 0.0+0.0i  # CXT
                  n556 = case shown="30" w1622 {
                    tunnel: w1625 -> [w1626 _ w1636 w1651 w1666 w1681]
                    tunnel: [w1626 w1627 w1638 w1653 w1668 w1683] -> w1624
                    tunnel: w1623 -> [_ w1629 w1639 w1654 w1669 w1684]
                    tunnel: w1621 -> [_ _ w1634 w1649 w1664 _]
                    tunnel: w1620 -> [_ w1631 w1633 w1648 w1663 w1679]
                    tunnel: [_ TRUE w1632 w1647 w1662 w1678] -> w1619
                    frame Default {
                      # "INCOMPATIBLE DATATYPES"
                    }
                    frame 14 {
                      # "CXT (0x0E)"
                      n557 = Variant To Flattened String(Variant=w1631) -> (data string=w1630:string)  [unwired: 1 out]
                      n558 = Flattened String To Variant(6:w1630, 7:w1629) -> (3:w1627:variant)  [unwired: 1 in, 1 out]
                    }
                    frame 1..8 {
                      # "I8, I16, I32, I64, U8, U16, U32, U64"
                      n559 = Variant To Data(type=w1634, Variant=w1633) -> (data=w1635:cxt, error out=w1637:errorcluster)  [unwired: 1 in]
                      n560 = case shown="No Error" w1637 {
                        tunnel: w1639 -> [w1645 _]
                        tunnel: [w1644 w1646] -> w1638
                        tunnel: w1636 -> [_ w1646]
                        tunnel: w1635 -> [w1642 _]
                        tunnel: [TRUE _] -> w1632
                        frame No Error {
                          n561 = To Variant(anything=w1642) -> (Variant=w1641:variant)
                          n562 = Variant To Flattened String(Variant=w1641) -> (data string=w1643:string)  [unwired: 1 out]
                          n563 = Flattened String To Variant(6:w1643, 7:w1645) -> (3:w1644:variant)  [unwired: 1 in, 1 out]
                        }
                        frame Error {
                        }
                      }
                    }
                    frame 9..13 {
                      # "SGL, DBL, EXT, CSG, CDB (0x09 .. 0x0E)"
                      n564 = Variant To Data(type=w1649, Variant=w1648) -> (data=w1650:cxt, error out=w1652:errorcluster)  [unwired: 1 in]
                      n565 = case shown="No Error" w1652 {
                        tunnel: w1654 -> [w1660 _]
                        tunnel: [w1659 w1661] -> w1653
                        tunnel: w1651 -> [_ w1661]
                        tunnel: w1650 -> [w1657 _]
                        tunnel: [TRUE _] -> w1647
                        frame No Error {
                          n566 = To Variant(anything=w1657) -> (Variant=w1656:variant)
                          n567 = Variant To Flattened String(Variant=w1656) -> (data string=w1658:string)  [unwired: 1 out]
                          n568 = Flattened String To Variant(6:w1658, 7:w1660) -> (3:w1659:variant)  [unwired: 1 in, 1 out]
                        }
                        frame Error {
                        }
                      }
                    }
                    frame 25..30 {
                      # "Physical Units (0x19 .. 0x1E)"
                      n569 = Variant To Data(type=w1664, Variant=w1663) -> (data=w1665:cxt, error out=w1667:errorcluster)  [unwired: 1 in]
                      n570 = case shown="No Error" w1667 {
                        tunnel: w1669 -> [w1675 _]
                        tunnel: [w1674 w1676] -> w1668
                        tunnel: w1666 -> [_ w1676]
                        tunnel: w1665 -> [w1672 _]
                        tunnel: [TRUE _] -> w1662
                        frame No Error {
                          n571 = To Variant(anything=w1672) -> (Variant=w1671:variant)
                          n572 = Variant To Flattened String(Variant=w1671) -> (data string=w1673:string)  [unwired: 1 out]
                          n573 = Flattened String To Variant(6:w1673, 7:w1675) -> (3:w1674:variant)  [unwired: 1 in, 1 out]
                        }
                        frame Error {
                        }
                      }
                    }
                    frame 48 {
                      # "String (0x30)"
                      n574 = Variant To Data(type="", Variant=w1679) -> (data=w1680:string, error out=w1682:errorcluster)  [unwired: 1 in]
                      n575 = case shown="No Error" w1682 {
                        tunnel: w1684 -> [w1691 _]
                        tunnel: [w1690 w1692] -> w1683
                        tunnel: w1681 -> [_ w1692]
                        tunnel: w1680 -> [w1686 _]
                        tunnel: [TRUE _] -> w1678
                        frame No Error {
                          n576 = call "String to ExtendedComplex (Scalar).vi"("Value (String)"=w1686) -> ("Value (CXT)"=w1685:cxt)  [unwired: 8 in, 2 out]
                          n577 = To Variant(anything=w1685) -> (Variant=w1688:variant)
                          n578 = Variant To Flattened String(Variant=w1688) -> (data string=w1689:string)  [unwired: 1 out]
                          n579 = Flattened String To Variant(6:w1689, 7:w1691) -> (3:w1690:variant)  [unwired: 1 in, 1 out]
                        }
                        frame Error {
                        }
                      }
                    }
                  }
                }
              }
            }
            frame 23 {
              # "Enum U32 (0x17)"
              n580 = Variant To Flattened String(Variant=w1699) -> (1:w1703:i16[])  [unwired: 1 out]
              n581 = call "TypeDescriptor_GetType.vi"("type descriptor"=w1703) -> ("Type"=w1693:u8)  [unwired: 9 in, 1 out]
              n582 = Equal?(x=w1694, y=w1693) -> (x = y?=w1697:bool)
              n583 = Compound Arithmetic op=OR(w1697, invert w1695) -> (w1696:bool)
              n584 = case shown="True" w1696 {
                tunnel: w1702 -> [w1704 w1706]
                tunnel: [w1704 w1711] -> w1701
                tunnel: w1700 -> [_ w1710]
                tunnel: w1693 -> [_ w1709]
                tunnel: w1699 -> [_ w1705]
                tunnel: [_ w1707] -> w1698
                frame False {
                }
                frame True {
                  w1708 = u32 0  # U32
                  n585 = case shown="16" w1709 {
                    tunnel: w1706 -> [w1712 w1714 _ _ _ w1750 w1772 w1787]
                    tunnel: [w1712 w1720 w1731 w1740 w1748 w1758 w1774 w1789] -> w1711
                    tunnel: w1710 -> [_ w1713 w1732 w1733 w1741 w1755 w1775 w1790]
                    tunnel: w1708 -> [_ w1717 _ _ _ w1752 w1770 w1785]
                    tunnel: w1705 -> [_ w1716 w1729 w1738 w1746 w1756 w1769 w1784]
                    tunnel: [_ w1715 TRUE TRUE TRUE w1749 w1768 w1783] -> w1707
                    frame Default {
                      # "INCOMPATIBLE DATATYPES"
                    }
                    frame 1..8 {
                      # "I8, I16, I32, I64, U8, U16, U32, U64"
                      n586 = Variant To Data(type=w1717, Variant=w1716) -> (data=w1718:u32, error out=w1719:errorcluster)  [unwired: 1 in]
                      n587 = case shown="No Error" w1719 {
                        tunnel: w1713 -> [w1726 _]
                        tunnel: [w1725 w1727] -> w1720
                        tunnel: w1714 -> [_ w1727]
                        tunnel: w1718 -> [w1723 _]
                        tunnel: [TRUE _] -> w1715
                        frame No Error {
                          n588 = To Variant(anything=w1723) -> (Variant=w1722:variant)
                          n589 = Variant To Flattened String(Variant=w1722) -> (data string=w1724:string)  [unwired: 1 out]
                          n590 = Flattened String To Variant(6:w1724, 7:w1726) -> (3:w1725:variant)  [unwired: 1 in, 1 out]
                        }
                        frame Error {
                        }
                      }
                    }
                    frame 23 {
                      # "Enum U32"
                      n591 = Variant To Flattened String(Variant=w1729) -> (data string=w1728:string)  [unwired: 1 out]
                      n592 = Flattened String To Variant(6:w1728, 7:w1732) -> (3:w1731:variant)  [unwired: 1 in, 1 out]
                    }
                    frame 22 {
                      # "Enum U16"
                      n593 = Variant To Flattened String(Variant=w1738) -> (data string=w1737:string)  [unwired: 1 out]
                      n594 = Byte Array To String(unsigned byte array=u8[] [0, 0]) -> (string=w1736:string)
                      n595 = Concatenate Strings(w1736, w1737) -> (w1734:string)
                      n596 = Flattened String To Variant(6:w1734, 7:w1733) -> (3:w1740:variant)  [unwired: 1 in, 1 out]
                    }
                    frame 21 {
                      # "Enum U8"
                      n597 = Variant To Flattened String(Variant=w1746) -> (data string=w1745:string)  [unwired: 1 out]
                      n598 = Byte Array To String(unsigned byte array=u8[] [0, 0, 0]) -> (string=w1744:string)
                      n599 = Concatenate Strings(w1744, w1745) -> (w1742:string)
                      n600 = Flattened String To Variant(6:w1742, 7:w1741) -> (3:w1748:variant)  [unwired: 1 in, 1 out]
                    }
                    frame 48 {
                      # "String (0x30)"
                      n601 = call "TypeDescriptor_ListElementNames.vi"("type descriptor"=w1755) -> ("element names"=w1754:string[])  [unwired: 7 in, 3 out]
                      n602 = Variant To Data(type="", Variant=w1756) -> (data=w1753:string)  [unwired: 1 in, 1 out]
                      n603 = Search 1D Array(1D array=w1754, element=w1753) -> (index of element=w1751:i32)  [unwired: 1 in]
                      n604 = case shown="Default" w1751 {
                        selector: w1751 -> [_ w1761]
                        tunnel: [w1759 w1767] -> w1758
                        tunnel: w1755 -> [_ w1766]
                        tunnel: w1752 -> [_ w1764]
                        tunnel: w1750 -> [w1759 _]
                        tunnel: [_ TRUE] -> w1749
                        frame -1 {
                        }
                        frame Default {
                          n605 = Variant To Data(type=w1764, Variant=w1761) -> (data=w1763:u32)  [unwired: 1 in, 1 out]
                          n606 = To Variant(anything=w1763) -> (Variant=w1765:variant)
                          n607 = Variant To Flattened String(Variant=w1765) -> (data string=w1762:string)  [unwired: 1 out]
                          n608 = Flattened String To Variant(6:w1762, 7:w1766) -> (3:w1767:variant)  [unwired: 1 in, 1 out]
                        }
                      }
                    }
                    frame 9..13 {
                      # "SGL, DBL, EXT, CSG, CDB (0x09 .. 0x0E)"
                      n609 = Variant To Data(type=w1770, Variant=w1769) -> (data=w1771:u32, error out=w1773:errorcluster)  [unwired: 1 in]
                      n610 = case shown="No Error" w1773 {
                        tunnel: w1775 -> [w1781 _]
                        tunnel: [w1780 w1782] -> w1774
                        tunnel: w1772 -> [_ w1782]
                        tunnel: w1771 -> [w1778 _]
                        tunnel: [TRUE _] -> w1768
                        frame No Error {
                          n611 = To Variant(anything=w1778) -> (Variant=w1777:variant)
                          n612 = Variant To Flattened String(Variant=w1777) -> (data string=w1779:string)  [unwired: 1 out]
                          n613 = Flattened String To Variant(6:w1779, 7:w1781) -> (3:w1780:variant)  [unwired: 1 in, 1 out]
                        }
                        frame Error {
                        }
                      }
                    }
                    frame 25..30 {
                      # "Physical Units (0x19 .. 0x1E)"
                      n614 = Variant To Data(type=w1785, Variant=w1784) -> (data=w1786:u32, error out=w1788:errorcluster)  [unwired: 1 in]
                      n615 = case shown="No Error" w1788 {
                        tunnel: w1790 -> [w1796 _]
                        tunnel: [w1795 w1797] -> w1789
                        tunnel: w1787 -> [_ w1797]
                        tunnel: w1786 -> [w1793 _]
                        tunnel: [TRUE _] -> w1783
                        frame No Error {
                          n616 = To Variant(anything=w1793) -> (Variant=w1792:variant)
                          n617 = Variant To Flattened String(Variant=w1792) -> (data string=w1794:string)  [unwired: 1 out]
                          n618 = Flattened String To Variant(6:w1794, 7:w1796) -> (3:w1795:variant)  [unwired: 1 in, 1 out]
                        }
                        frame Error {
                        }
                      }
                    }
                  }
                }
              }
            }
            frame 22 {
              # "Enum U16 (0x16)"
              n619 = Variant To Flattened String(Variant=w1804) -> (1:w1808:i16[])  [unwired: 1 out]
              n620 = call "TypeDescriptor_GetType.vi"("type descriptor"=w1808) -> ("Type"=w1798:u8)  [unwired: 9 in, 1 out]
              n621 = Equal?(x=w1799, y=w1798) -> (x = y?=w1802:bool)
              n622 = Compound Arithmetic op=OR(w1802, invert w1800) -> (w1801:bool)
              n623 = case shown="True" w1801 {
                tunnel: w1807 -> [w1809 w1811]
                tunnel: [w1809 w1816] -> w1806
                tunnel: w1805 -> [_ w1815]
                tunnel: w1798 -> [_ w1814]
                tunnel: w1804 -> [_ w1810]
                tunnel: [_ w1812] -> w1803
                frame False {
                }
                frame True {
                  w1813 = u16 0  # U16
                  n624 = case shown="30" w1814 {
                    tunnel: w1811 -> [w1817 w1819 _ _ _ w1854 w1876 w1891]
                    tunnel: [w1817 w1825 w1836 w1844 w1852 w1862 w1878 w1893] -> w1816
                    tunnel: w1815 -> [_ w1818 w1837 w1841 w1845 w1859 w1879 w1894]
                    tunnel: w1813 -> [_ w1822 _ _ _ w1856 w1874 w1889]
                    tunnel: w1810 -> [_ w1821 w1834 w1842 w1850 w1860 w1873 w1888]
                    tunnel: [_ w1820 TRUE TRUE TRUE w1853 w1872 w1887] -> w1812
                    frame Default {
                      # "INCOMPATIBLE DATATYPES"
                    }
                    frame 1..8 {
                      # "I8, I16, I32, I64, U8, U16, U32, U64"
                      n625 = Variant To Data(type=w1822, Variant=w1821) -> (data=w1823:u16, error out=w1824:errorcluster)  [unwired: 1 in]
                      n626 = case shown="No Error" w1824 {
                        tunnel: w1818 -> [w1831 _]
                        tunnel: [w1830 w1832] -> w1825
                        tunnel: w1819 -> [_ w1832]
                        tunnel: w1823 -> [w1828 _]
                        tunnel: [TRUE _] -> w1820
                        frame No Error {
                          n627 = To Variant(anything=w1828) -> (Variant=w1827:variant)
                          n628 = Variant To Flattened String(Variant=w1827) -> (data string=w1829:string)  [unwired: 1 out]
                          n629 = Flattened String To Variant(6:w1829, 7:w1831) -> (3:w1830:variant)  [unwired: 1 in, 1 out]
                        }
                        frame Error {
                        }
                      }
                    }
                    frame 22 {
                      # "Enum U16"
                      n630 = Variant To Flattened String(Variant=w1834) -> (data string=w1833:string)  [unwired: 1 out]
                      n631 = Flattened String To Variant(6:w1833, 7:w1837) -> (3:w1836:variant)  [unwired: 1 in, 1 out]
                    }
                    frame 23 {
                      # "Enum U32"
                      n632 = Variant To Flattened String(Variant=w1842) -> (data string=w1840:string)  [unwired: 1 out]
                      n633 = String Subset(string=w1840, offset (0)=2) -> (substring=w1838:string)  [unwired: 1 in]
                      n634 = Flattened String To Variant(6:w1838, 7:w1841) -> (3:w1844:variant)  [unwired: 1 in, 1 out]
                    }
                    frame 21 {
                      # "Enum U8"
                      n635 = Variant To Flattened String(Variant=w1850) -> (data string=w1849:string)  [unwired: 1 out]
                      n636 = Byte Array To String(unsigned byte array=u8[] [0]) -> (string=w1848:string)
                      n637 = Concatenate Strings(w1848, w1849) -> (w1846:string)
                      n638 = Flattened String To Variant(6:w1846, 7:w1845) -> (3:w1852:variant)  [unwired: 1 in, 1 out]
                    }
                    frame 48 {
                      # "String (0x30)"
                      n639 = call "TypeDescriptor_ListElementNames.vi"("type descriptor"=w1859) -> ("element names"=w1858:string[])  [unwired: 7 in, 3 out]
                      n640 = Variant To Data(type="", Variant=w1860) -> (data=w1857:string)  [unwired: 1 in, 1 out]
                      n641 = Search 1D Array(1D array=w1858, element=w1857) -> (index of element=w1855:i32)  [unwired: 1 in]
                      n642 = case shown="Default" w1855 {
                        selector: w1855 -> [_ w1865]
                        tunnel: [w1863 w1871] -> w1862
                        tunnel: w1859 -> [_ w1870]
                        tunnel: w1856 -> [_ w1868]
                        tunnel: w1854 -> [w1863 _]
                        tunnel: [_ TRUE] -> w1853
                        frame -1 {
                        }
                        frame Default {
                          n643 = Variant To Data(type=w1868, Variant=w1865) -> (data=w1867:u16)  [unwired: 1 in, 1 out]
                          n644 = To Variant(anything=w1867) -> (Variant=w1869:variant)
                          n645 = Variant To Flattened String(Variant=w1869) -> (data string=w1866:string)  [unwired: 1 out]
                          n646 = Flattened String To Variant(6:w1866, 7:w1870) -> (3:w1871:variant)  [unwired: 1 in, 1 out]
                        }
                      }
                    }
                    frame 9..13 {
                      # "SGL, DBL, EXT, CSG, CDB (0x09 .. 0x0E)"
                      n647 = Variant To Data(type=w1874, Variant=w1873) -> (data=w1875:u16, error out=w1877:errorcluster)  [unwired: 1 in]
                      n648 = case shown="No Error" w1877 {
                        tunnel: w1879 -> [w1885 _]
                        tunnel: [w1884 w1886] -> w1878
                        tunnel: w1876 -> [_ w1886]
                        tunnel: w1875 -> [w1882 _]
                        tunnel: [TRUE _] -> w1872
                        frame No Error {
                          n649 = To Variant(anything=w1882) -> (Variant=w1881:variant)
                          n650 = Variant To Flattened String(Variant=w1881) -> (data string=w1883:string)  [unwired: 1 out]
                          n651 = Flattened String To Variant(6:w1883, 7:w1885) -> (3:w1884:variant)  [unwired: 1 in, 1 out]
                        }
                        frame Error {
                        }
                      }
                    }
                    frame 25..30 {
                      # "Physical Units (0x19 .. 0x1E)"
                      n652 = Variant To Data(type=w1889, Variant=w1888) -> (data=w1890:u16, error out=w1892:errorcluster)  [unwired: 1 in]
                      n653 = case shown="No Error" w1892 {
                        tunnel: w1894 -> [w1900 _]
                        tunnel: [w1899 w1901] -> w1893
                        tunnel: w1891 -> [_ w1901]
                        tunnel: w1890 -> [w1897 _]
                        tunnel: [TRUE _] -> w1887
                        frame No Error {
                          n654 = To Variant(anything=w1897) -> (Variant=w1896:variant)
                          n655 = Variant To Flattened String(Variant=w1896) -> (data string=w1898:string)  [unwired: 1 out]
                          n656 = Flattened String To Variant(6:w1898, 7:w1900) -> (3:w1899:variant)  [unwired: 1 in, 1 out]
                        }
                        frame Error {
                        }
                      }
                    }
                  }
                }
              }
            }
            frame 21 {
              # "Enum U8 (0x15)"
              n657 = Variant To Flattened String(Variant=w1908) -> (1:w1912:i16[])  [unwired: 1 out]
              n658 = call "TypeDescriptor_GetType.vi"("type descriptor"=w1912) -> ("Type"=w1902:u8)  [unwired: 9 in, 1 out]
              n659 = Equal?(x=w1903, y=w1902) -> (x = y?=w1906:bool)
              n660 = Compound Arithmetic op=OR(w1906, invert w1904) -> (w1905:bool)
              n661 = case shown="True" w1905 {
                tunnel: w1911 -> [w1913 w1915]
                tunnel: [w1913 w1920] -> w1910
                tunnel: w1909 -> [_ w1919]
                tunnel: w1902 -> [_ w1918]
                tunnel: w1908 -> [_ w1914]
                tunnel: [_ w1916] -> w1907
                frame False {
                }
                frame True {
                  w1917 = u8 0  # U8
                  n662 = case shown="30" w1918 {
                    tunnel: w1915 -> [w1921 w1923 _ _ _ w1957 w1979 w1994]
                    tunnel: [w1921 w1929 w1940 w1948 w1955 w1965 w1981 w1996] -> w1920
                    tunnel: w1919 -> [_ w1922 w1941 w1945 w1952 w1962 w1982 w1997]
                    tunnel: w1917 -> [_ w1926 _ _ _ w1959 w1977 w1992]
                    tunnel: w1914 -> [_ w1925 w1938 w1946 w1953 w1963 w1976 w1991]
                    tunnel: [_ w1924 TRUE TRUE TRUE w1956 w1975 w1990] -> w1916
                    frame Default {
                      # "INCOMPATIBLE DATATYPES"
                    }
                    frame 1..8 {
                      # "I8, I16, I32, I64, U8, U16, U32, U64"
                      n663 = Variant To Data(type=w1926, Variant=w1925) -> (data=w1927:u8, error out=w1928:errorcluster)  [unwired: 1 in]
                      n664 = case shown="No Error" w1928 {
                        tunnel: w1922 -> [w1935 _]
                        tunnel: [w1934 w1936] -> w1929
                        tunnel: w1923 -> [_ w1936]
                        tunnel: w1927 -> [w1932 _]
                        tunnel: [TRUE _] -> w1924
                        frame No Error {
                          n665 = To Variant(anything=w1932) -> (Variant=w1931:variant)
                          n666 = Variant To Flattened String(Variant=w1931) -> (data string=w1933:string)  [unwired: 1 out]
                          n667 = Flattened String To Variant(6:w1933, 7:w1935) -> (3:w1934:variant)  [unwired: 1 in, 1 out]
                        }
                        frame Error {
                        }
                      }
                    }
                    frame 21 {
                      # "Enum U8"
                      n668 = Variant To Flattened String(Variant=w1938) -> (data string=w1937:string)  [unwired: 1 out]
                      n669 = Flattened String To Variant(6:w1937, 7:w1941) -> (3:w1940:variant)  [unwired: 1 in, 1 out]
                    }
                    frame 23 {
                      # "Enum U32"
                      n670 = Variant To Flattened String(Variant=w1946) -> (data string=w1944:string)  [unwired: 1 out]
                      n671 = String Subset(string=w1944, offset (0)=3) -> (substring=w1942:string)  [unwired: 1 in]
                      n672 = Flattened String To Variant(6:w1942, 7:w1945) -> (3:w1948:variant)  [unwired: 1 in, 1 out]
                    }
                    frame 22 {
                      # "Enum U16"
                      n673 = Variant To Flattened String(Variant=w1953) -> (data string=w1951:string)  [unwired: 1 out]
                      n674 = String Subset(string=w1951, offset (0)=1) -> (substring=w1950:string)  [unwired: 1 in]
                      n675 = Flattened String To Variant(6:w1950, 7:w1952) -> (3:w1955:variant)  [unwired: 1 in, 1 out]
                    }
                    frame 48 {
                      # "String (0x30)"
                      n676 = call "TypeDescriptor_ListElementNames.vi"("type descriptor"=w1962) -> ("element names"=w1961:string[])  [unwired: 7 in, 3 out]
                      n677 = Variant To Data(type="", Variant=w1963) -> (data=w1960:string)  [unwired: 1 in, 1 out]
                      n678 = Search 1D Array(1D array=w1961, element=w1960) -> (index of element=w1958:i32)  [unwired: 1 in]
                      n679 = case shown="Default" w1958 {
                        selector: w1958 -> [_ w1968]
                        tunnel: [w1966 w1974] -> w1965
                        tunnel: w1962 -> [_ w1973]
                        tunnel: w1959 -> [_ w1971]
                        tunnel: w1957 -> [w1966 _]
                        tunnel: [_ TRUE] -> w1956
                        frame -1 {
                        }
                        frame Default {
                          n680 = Variant To Data(type=w1971, Variant=w1968) -> (data=w1970:u8)  [unwired: 1 in, 1 out]
                          n681 = To Variant(anything=w1970) -> (Variant=w1972:variant)
                          n682 = Variant To Flattened String(Variant=w1972) -> (data string=w1969:string)  [unwired: 1 out]
                          n683 = Flattened String To Variant(6:w1969, 7:w1973) -> (3:w1974:variant)  [unwired: 1 in, 1 out]
                        }
                      }
                    }
                    frame 9..13 {
                      # "SGL, DBL, EXT, CSG, CDB (0x09 .. 0x0E)"
                      n684 = Variant To Data(type=w1977, Variant=w1976) -> (data=w1978:u8, error out=w1980:errorcluster)  [unwired: 1 in]
                      n685 = case shown="No Error" w1980 {
                        tunnel: w1982 -> [w1988 _]
                        tunnel: [w1987 w1989] -> w1981
                        tunnel: w1979 -> [_ w1989]
                        tunnel: w1978 -> [w1985 _]
                        tunnel: [TRUE _] -> w1975
                        frame No Error {
                          n686 = To Variant(anything=w1985) -> (Variant=w1984:variant)
                          n687 = Variant To Flattened String(Variant=w1984) -> (data string=w1986:string)  [unwired: 1 out]
                          n688 = Flattened String To Variant(6:w1986, 7:w1988) -> (3:w1987:variant)  [unwired: 1 in, 1 out]
                        }
                        frame Error {
                        }
                      }
                    }
                    frame 25..30 {
                      # "Physical Units (0x19 .. 0x1E)"
                      n689 = Variant To Data(type=w1992, Variant=w1991) -> (data=w1993:u8, error out=w1995:errorcluster)  [unwired: 1 in]
                      n690 = case shown="No Error" w1995 {
                        tunnel: w1997 -> [w2003 _]
                        tunnel: [w2002 w2004] -> w1996
                        tunnel: w1994 -> [_ w2004]
                        tunnel: w1993 -> [w2000 _]
                        tunnel: [TRUE _] -> w1990
                        frame No Error {
                          n691 = To Variant(anything=w2000) -> (Variant=w1999:variant)
                          n692 = Variant To Flattened String(Variant=w1999) -> (data string=w2001:string)  [unwired: 1 out]
                          n693 = Flattened String To Variant(6:w2001, 7:w2003) -> (3:w2002:variant)  [unwired: 1 in, 1 out]
                        }
                        frame Error {
                        }
                      }
                    }
                  }
                }
              }
            }
            frame 25 {
              # "SGL PhysUnit (0x19)"
              n694 = Variant To Flattened String(Variant=w2011) -> (1:w2015:i16[])  [unwired: 1 out]
              n695 = call "TypeDescriptor_GetType.vi"("type descriptor"=w2015) -> ("Type"=w2006:u8)  [unwired: 9 in, 1 out]
              n696 = Equal?(x=w2005, y=w2006) -> (x = y?=w2009:bool)
              n697 = Compound Arithmetic op=OR(w2009, invert w2007) -> (w2008:bool)
              n698 = case shown="True" w2008 {
                tunnel: w2014 -> [w2016 w2023]
                tunnel: [w2016 w2022] -> w2013
                tunnel: w2012 -> [_ w2021]
                tunnel: w2006 -> [_ w2020]
                tunnel: w2011 -> [_ w2018]
                tunnel: [_ w2017] -> w2010
                frame False {
                }
                frame True {
                  w2019 = sgl 0.0  # SGL
                  n699 = case shown="1..8" w2020 {
                    tunnel: w2023 -> [w2024 _ w2034 w2049 w2064]
                    tunnel: [w2024 w2026 w2036 w2051 w2066] -> w2022
                    tunnel: w2021 -> [_ w2027 w2037 w2052 w2067]
                    tunnel: w2019 -> [_ _ w2032 w2047 w2062]
                    tunnel: w2018 -> [_ w2029 w2031 w2046 w2061]
                    tunnel: [_ TRUE w2030 w2045 w2060] -> w2017
                    frame Default {
                      # "INCOMPATIBLE DATATYPES"
                    }
                    frame 25 {
                      # "SGL PhysUnit (0x19)"
                      n700 = Variant To Flattened String(Variant=w2029) -> (data string=w2028:string)  [unwired: 1 out]
                      n701 = Flattened String To Variant(6:w2028, 7:w2027) -> (3:w2026:variant)  [unwired: 1 in, 1 out]
                    }
                    frame 1..8 {
                      # "I8, I16, I32, I64, U8, U16, U32, U64"
                      n702 = Variant To Data(type=w2032, Variant=w2031) -> (data=w2033:sgl, error out=w2035:errorcluster)  [unwired: 1 in]
                      n703 = case shown="No Error" w2035 {
                        tunnel: w2037 -> [w2043 _]
                        tunnel: [w2042 w2044] -> w2036
                        tunnel: w2034 -> [_ w2044]
                        tunnel: w2033 -> [w2040 _]
                        tunnel: [TRUE _] -> w2030
                        frame No Error {
                          n704 = To Variant(anything=w2040) -> (Variant=w2039:variant)
                          n705 = Variant To Flattened String(Variant=w2039) -> (data string=w2041:string)  [unwired: 1 out]
                          n706 = Flattened String To Variant(6:w2041, 7:w2043) -> (3:w2042:variant)  [unwired: 1 in, 1 out]
                        }
                        frame Error {
                        }
                      }
                    }
                    frame 9..14 {
                      # "SGL, DBL, EXT, CSG, CDB (0x09 .. 0x0E)"
                      n707 = Variant To Data(type=w2047, Variant=w2046) -> (data=w2048:sgl, error out=w2050:errorcluster)  [unwired: 1 in]
                      n708 = case shown="No Error" w2050 {
                        tunnel: w2052 -> [w2058 _]
                        tunnel: [w2057 w2059] -> w2051
                        tunnel: w2049 -> [_ w2059]
                        tunnel: w2048 -> [w2055 _]
                        tunnel: [TRUE _] -> w2045
                        frame No Error {
                          n709 = To Variant(anything=w2055) -> (Variant=w2054:variant)
                          n710 = Variant To Flattened String(Variant=w2054) -> (data string=w2056:string)  [unwired: 1 out]
                          n711 = Flattened String To Variant(6:w2056, 7:w2058) -> (3:w2057:variant)  [unwired: 1 in, 1 out]
                        }
                        frame Error {
                        }
                      }
                    }
                    frame 26..30 {
                      # "Physical Units (0x19 .. 0x1E)"
                      n712 = Variant To Data(type=w2062, Variant=w2061) -> (data=w2063:sgl, error out=w2065:errorcluster)  [unwired: 1 in]
                      n713 = case shown="No Error" w2065 {
                        tunnel: w2067 -> [w2073 _]
                        tunnel: [w2072 w2074] -> w2066
                        tunnel: w2064 -> [_ w2074]
                        tunnel: w2063 -> [w2070 _]
                        tunnel: [TRUE _] -> w2060
                        frame No Error {
                          n714 = To Variant(anything=w2070) -> (Variant=w2069:variant)
                          n715 = Variant To Flattened String(Variant=w2069) -> (data string=w2071:string)  [unwired: 1 out]
                          n716 = Flattened String To Variant(6:w2071, 7:w2073) -> (3:w2072:variant)  [unwired: 1 in, 1 out]
                        }
                        frame Error {
                        }
                      }
                    }
                  }
                }
              }
            }
            frame 26 {
              # "DBL PhysUnit (0x1A)"
              n717 = Variant To Flattened String(Variant=w2081) -> (1:w2085:i16[])  [unwired: 1 out]
              n718 = call "TypeDescriptor_GetType.vi"("type descriptor"=w2085) -> ("Type"=w2076:u8)  [unwired: 9 in, 1 out]
              n719 = Equal?(x=w2077, y=w2076) -> (x = y?=w2079:bool)
              n720 = Compound Arithmetic op=OR(w2079, invert w2075) -> (w2078:bool)
              n721 = case shown="True" w2078 {
                tunnel: w2084 -> [w2086 w2093]
                tunnel: [w2086 w2092] -> w2083
                tunnel: w2082 -> [_ w2091]
                tunnel: w2076 -> [_ w2090]
                tunnel: w2081 -> [_ w2088]
                tunnel: [_ w2087] -> w2080
                frame False {
                }
                frame True {
                  w2089 = 0.0  # DBL
                  n722 = case shown="1..8" w2090 {
                    tunnel: w2093 -> [w2094 _ w2104 w2119 w2134]
                    tunnel: [w2094 w2096 w2106 w2121 w2136] -> w2092
                    tunnel: w2091 -> [_ w2097 w2107 w2122 w2137]
                    tunnel: w2089 -> [_ _ w2102 w2117 w2132]
                    tunnel: w2088 -> [_ w2099 w2101 w2116 w2131]
                    tunnel: [_ TRUE w2100 w2115 w2130] -> w2087
                    frame Default {
                      # "INCOMPATIBLE DATATYPES"
                    }
                    frame 26 {
                      # "DBL PhysUnit (0x1A)"
                      n723 = Variant To Flattened String(Variant=w2099) -> (data string=w2098:string)  [unwired: 1 out]
                      n724 = Flattened String To Variant(6:w2098, 7:w2097) -> (3:w2096:variant)  [unwired: 1 in, 1 out]
                    }
                    frame 1..8 {
                      # "I8, I16, I32, I64, U8, U16, U32, U64"
                      n725 = Variant To Data(type=w2102, Variant=w2101) -> (data=w2103:dbl, error out=w2105:errorcluster)  [unwired: 1 in]
                      n726 = case shown="No Error" w2105 {
                        tunnel: w2107 -> [w2113 _]
                        tunnel: [w2112 w2114] -> w2106
                        tunnel: w2104 -> [_ w2114]
                        tunnel: w2103 -> [w2110 _]
                        tunnel: [TRUE _] -> w2100
                        frame No Error {
                          n727 = To Variant(anything=w2110) -> (Variant=w2109:variant)
                          n728 = Variant To Flattened String(Variant=w2109) -> (data string=w2111:string)  [unwired: 1 out]
                          n729 = Flattened String To Variant(6:w2111, 7:w2113) -> (3:w2112:variant)  [unwired: 1 in, 1 out]
                        }
                        frame Error {
                        }
                      }
                    }
                    frame 9..14 {
                      # "SGL, DBL, EXT, CSG, CDB (0x09 .. 0x0E)"
                      n730 = Variant To Data(type=w2117, Variant=w2116) -> (data=w2118:dbl, error out=w2120:errorcluster)  [unwired: 1 in]
                      n731 = case shown="No Error" w2120 {
                        tunnel: w2122 -> [w2128 _]
                        tunnel: [w2127 w2129] -> w2121
                        tunnel: w2119 -> [_ w2129]
                        tunnel: w2118 -> [w2125 _]
                        tunnel: [TRUE _] -> w2115
                        frame No Error {
                          n732 = To Variant(anything=w2125) -> (Variant=w2124:variant)
                          n733 = Variant To Flattened String(Variant=w2124) -> (data string=w2126:string)  [unwired: 1 out]
                          n734 = Flattened String To Variant(6:w2126, 7:w2128) -> (3:w2127:variant)  [unwired: 1 in, 1 out]
                        }
                        frame Error {
                        }
                      }
                    }
                    frame 25, 27..30 {
                      # "Physical Units (0x19 .. 0x1E)"
                      n735 = Variant To Data(type=w2132, Variant=w2131) -> (data=w2133:dbl, error out=w2135:errorcluster)  [unwired: 1 in]
                      n736 = case shown="No Error" w2135 {
                        tunnel: w2137 -> [w2143 _]
                        tunnel: [w2142 w2144] -> w2136
                        tunnel: w2134 -> [_ w2144]
                        tunnel: w2133 -> [w2140 _]
                        tunnel: [TRUE _] -> w2130
                        frame No Error {
                          n737 = To Variant(anything=w2140) -> (Variant=w2139:variant)
                          n738 = Variant To Flattened String(Variant=w2139) -> (data string=w2141:string)  [unwired: 1 out]
                          n739 = Flattened String To Variant(6:w2141, 7:w2143) -> (3:w2142:variant)  [unwired: 1 in, 1 out]
                        }
                        frame Error {
                        }
                      }
                    }
                  }
                }
              }
            }
            frame 27 {
              # "EXT PhysUnit (0x1B)"
              n740 = Variant To Flattened String(Variant=w2151) -> (1:w2155:i16[])  [unwired: 1 out]
              n741 = call "TypeDescriptor_GetType.vi"("type descriptor"=w2155) -> ("Type"=w2145:u8)  [unwired: 9 in, 1 out]
              n742 = Equal?(x=w2146, y=w2145) -> (x = y?=w2149:bool)
              n743 = Compound Arithmetic op=OR(w2149, invert w2147) -> (w2148:bool)
              n744 = case shown="True" w2148 {
                tunnel: w2154 -> [w2156 w2163]
                tunnel: [w2156 w2162] -> w2153
                tunnel: w2152 -> [_ w2161]
                tunnel: w2145 -> [_ w2160]
                tunnel: w2151 -> [_ w2158]
                tunnel: [_ w2157] -> w2150
                frame False {
                }
                frame True {
                  w2159 = ext 0.0  # EXT
                  n745 = case shown="1..8" w2160 {
                    tunnel: w2163 -> [w2164 _ w2174 w2189 w2204]
                    tunnel: [w2164 w2166 w2176 w2191 w2206] -> w2162
                    tunnel: w2161 -> [_ w2167 w2177 w2192 w2207]
                    tunnel: w2159 -> [_ _ w2172 w2187 w2202]
                    tunnel: w2158 -> [_ w2169 w2171 w2186 w2201]
                    tunnel: [_ TRUE w2170 w2185 w2200] -> w2157
                    frame Default {
                      # "INCOMPATIBLE DATATYPES"
                    }
                    frame 27 {
                      # "EXT PhysUnit (0x1B)"
                      n746 = Variant To Flattened String(Variant=w2169) -> (data string=w2168:string)  [unwired: 1 out]
                      n747 = Flattened String To Variant(6:w2168, 7:w2167) -> (3:w2166:variant)  [unwired: 1 in, 1 out]
                    }
                    frame 1..8 {
                      # "I8, I16, I32, I64, U8, U16, U32, U64"
                      n748 = Variant To Data(type=w2172, Variant=w2171) -> (data=w2173:ext, error out=w2175:errorcluster)  [unwired: 1 in]
                      n749 = case shown="No Error" w2175 {
                        tunnel: w2177 -> [w2183 _]
                        tunnel: [w2182 w2184] -> w2176
                        tunnel: w2174 -> [_ w2184]
                        tunnel: w2173 -> [w2180 _]
                        tunnel: [TRUE _] -> w2170
                        frame No Error {
                          n750 = To Variant(anything=w2180) -> (Variant=w2179:variant)
                          n751 = Variant To Flattened String(Variant=w2179) -> (data string=w2181:string)  [unwired: 1 out]
                          n752 = Flattened String To Variant(6:w2181, 7:w2183) -> (3:w2182:variant)  [unwired: 1 in, 1 out]
                        }
                        frame Error {
                        }
                      }
                    }
                    frame 9..14 {
                      # "SGL, DBL, EXT, CSG, CDB (0x09 .. 0x0E)"
                      n753 = Variant To Data(type=w2187, Variant=w2186) -> (data=w2188:ext, error out=w2190:errorcluster)  [unwired: 1 in]
                      n754 = case shown="No Error" w2190 {
                        tunnel: w2192 -> [w2198 _]
                        tunnel: [w2197 w2199] -> w2191
                        tunnel: w2189 -> [_ w2199]
                        tunnel: w2188 -> [w2195 _]
                        tunnel: [TRUE _] -> w2185
                        frame No Error {
                          n755 = To Variant(anything=w2195) -> (Variant=w2194:variant)
                          n756 = Variant To Flattened String(Variant=w2194) -> (data string=w2196:string)  [unwired: 1 out]
                          n757 = Flattened String To Variant(6:w2196, 7:w2198) -> (3:w2197:variant)  [unwired: 1 in, 1 out]
                        }
                        frame Error {
                        }
                      }
                    }
                    frame 25, 26, 28..30 {
                      # "Physical Units (0x19 .. 0x1E)"
                      n758 = Variant To Data(type=w2202, Variant=w2201) -> (data=w2203:ext, error out=w2205:errorcluster)  [unwired: 1 in]
                      n759 = case shown="No Error" w2205 {
                        tunnel: w2207 -> [w2213 _]
                        tunnel: [w2212 w2214] -> w2206
                        tunnel: w2204 -> [_ w2214]
                        tunnel: w2203 -> [w2210 _]
                        tunnel: [TRUE _] -> w2200
                        frame No Error {
                          n760 = To Variant(anything=w2210) -> (Variant=w2209:variant)
                          n761 = Variant To Flattened String(Variant=w2209) -> (data string=w2211:string)  [unwired: 1 out]
                          n762 = Flattened String To Variant(6:w2211, 7:w2213) -> (3:w2212:variant)  [unwired: 1 in, 1 out]
                        }
                        frame Error {
                        }
                      }
                    }
                  }
                }
              }
            }
            frame 28 {
              # "CSG PhysUnit (0x1C)"
              n763 = Variant To Flattened String(Variant=w2221) -> (1:w2225:i16[])  [unwired: 1 out]
              n764 = call "TypeDescriptor_GetType.vi"("type descriptor"=w2225) -> ("Type"=w2218:u8)  [unwired: 9 in, 1 out]
              n765 = Equal?(x=w2217, y=w2218) -> (x = y?=w2219:bool)
              n766 = Compound Arithmetic op=OR(w2219, invert w2216) -> (w2215:bool)
              n767 = case shown="True" w2215 {
                tunnel: w2224 -> [w2226 w2233]
                tunnel: [w2226 w2232] -> w2223
                tunnel: w2222 -> [_ w2231]
                tunnel: w2221 -> [_ w2229]
                tunnel: [_ w2228] -> w2220
                tunnel: w2218 -> [_ w2227]
                frame False {
                }
                frame True {
                  w2230 = csg 0.0+0.0i  # CSG
                  n768 = case shown="1..8" w2227 {
                    tunnel: w2233 -> [w2234 _ w2244 w2259 w2274]
                    tunnel: [w2234 w2236 w2246 w2261 w2276] -> w2232
                    tunnel: w2231 -> [_ w2237 w2247 w2262 w2277]
                    tunnel: w2230 -> [_ _ w2242 w2257 w2272]
                    tunnel: w2229 -> [_ w2239 w2241 w2256 w2271]
                    tunnel: [_ TRUE w2240 w2255 w2270] -> w2228
                    frame Default {
                      # "INCOMPATIBLE DATATYPES"
                    }
                    frame 28 {
                      # "CSG PhysUnit (0x1C)"
                      n769 = Variant To Flattened String(Variant=w2239) -> (data string=w2238:string)  [unwired: 1 out]
                      n770 = Flattened String To Variant(6:w2238, 7:w2237) -> (3:w2236:variant)  [unwired: 1 in, 1 out]
                    }
                    frame 1..8 {
                      # "I8, I16, I32, I64, U8, U16, U32, U64"
                      n771 = Variant To Data(type=w2242, Variant=w2241) -> (data=w2243:csg, error out=w2245:errorcluster)  [unwired: 1 in]
                      n772 = case shown="No Error" w2245 {
                        tunnel: w2247 -> [w2253 _]
                        tunnel: [w2252 w2254] -> w2246
                        tunnel: w2244 -> [_ w2254]
                        tunnel: w2243 -> [w2250 _]
                        tunnel: [TRUE _] -> w2240
                        frame No Error {
                          n773 = To Variant(anything=w2250) -> (Variant=w2249:variant)
                          n774 = Variant To Flattened String(Variant=w2249) -> (data string=w2251:string)  [unwired: 1 out]
                          n775 = Flattened String To Variant(6:w2251, 7:w2253) -> (3:w2252:variant)  [unwired: 1 in, 1 out]
                        }
                        frame Error {
                        }
                      }
                    }
                    frame 9..14 {
                      # "SGL, DBL, EXT, CSG, CDB (0x09 .. 0x0E)"
                      n776 = Variant To Data(type=w2257, Variant=w2256) -> (data=w2258:csg, error out=w2260:errorcluster)  [unwired: 1 in]
                      n777 = case shown="No Error" w2260 {
                        tunnel: w2262 -> [w2268 _]
                        tunnel: [w2267 w2269] -> w2261
                        tunnel: w2259 -> [_ w2269]
                        tunnel: w2258 -> [w2265 _]
                        tunnel: [TRUE _] -> w2255
                        frame No Error {
                          n778 = To Variant(anything=w2265) -> (Variant=w2264:variant)
                          n779 = Variant To Flattened String(Variant=w2264) -> (data string=w2266:string)  [unwired: 1 out]
                          n780 = Flattened String To Variant(6:w2266, 7:w2268) -> (3:w2267:variant)  [unwired: 1 in, 1 out]
                        }
                        frame Error {
                        }
                      }
                    }
                    frame 25..27, 29, 30 {
                      # "Physical Units (0x19 .. 0x1E)"
                      n781 = Variant To Data(type=w2272, Variant=w2271) -> (data=w2273:csg, error out=w2275:errorcluster)  [unwired: 1 in]
                      n782 = case shown="No Error" w2275 {
                        tunnel: w2277 -> [w2283 _]
                        tunnel: [w2282 w2284] -> w2276
                        tunnel: w2274 -> [_ w2284]
                        tunnel: w2273 -> [w2280 _]
                        tunnel: [TRUE _] -> w2270
                        frame No Error {
                          n783 = To Variant(anything=w2280) -> (Variant=w2279:variant)
                          n784 = Variant To Flattened String(Variant=w2279) -> (data string=w2281:string)  [unwired: 1 out]
                          n785 = Flattened String To Variant(6:w2281, 7:w2283) -> (3:w2282:variant)  [unwired: 1 in, 1 out]
                        }
                        frame Error {
                        }
                      }
                    }
                  }
                }
              }
            }
            frame 29 {
              # "CDB PhysUnit (0x1D)"
              n786 = Variant To Flattened String(Variant=w2291) -> (1:w2295:i16[])  [unwired: 1 out]
              n787 = call "TypeDescriptor_GetType.vi"("type descriptor"=w2295) -> ("Type"=w2286:u8)  [unwired: 9 in, 1 out]
              n788 = Equal?(x=w2287, y=w2286) -> (x = y?=w2289:bool)
              n789 = Compound Arithmetic op=OR(w2289, invert w2285) -> (w2288:bool)
              n790 = case shown="True" w2288 {
                tunnel: w2294 -> [w2296 w2303]
                tunnel: [w2296 w2302] -> w2293
                tunnel: w2292 -> [_ w2301]
                tunnel: w2286 -> [_ w2300]
                tunnel: w2291 -> [_ w2298]
                tunnel: [_ w2297] -> w2290
                frame False {
                }
                frame True {
                  w2299 = cdb 0.0+0.0i  # CDB
                  n791 = case shown="19..1C, 1E" w2300 {
                    tunnel: w2303 -> [w2304 _ w2314 w2329 w2344]
                    tunnel: [w2304 w2305 w2316 w2331 w2346] -> w2302
                    tunnel: w2301 -> [_ w2307 w2317 w2332 w2347]
                    tunnel: w2299 -> [_ _ w2312 w2327 w2342]
                    tunnel: w2298 -> [_ w2309 w2311 w2326 w2341]
                    tunnel: [_ TRUE w2310 w2325 w2340] -> w2297
                    frame Default {
                      # "INCOMPATIBLE DATATYPES"
                    }
                    frame 29 {
                      # "CDB PhysUnit (0x1D)"
                      n792 = Variant To Flattened String(Variant=w2309) -> (data string=w2308:string)  [unwired: 1 out]
                      n793 = Flattened String To Variant(6:w2308, 7:w2307) -> (3:w2305:variant)  [unwired: 1 in, 1 out]
                    }
                    frame 1..8 {
                      # "I8, I16, I32, I64, U8, U16, U32, U64"
                      n794 = Variant To Data(type=w2312, Variant=w2311) -> (data=w2313:cdb, error out=w2315:errorcluster)  [unwired: 1 in]
                      n795 = case shown="No Error" w2315 {
                        tunnel: w2317 -> [w2323 _]
                        tunnel: [w2322 w2324] -> w2316
                        tunnel: w2314 -> [_ w2324]
                        tunnel: w2313 -> [w2320 _]
                        tunnel: [TRUE _] -> w2310
                        frame No Error {
                          n796 = To Variant(anything=w2320) -> (Variant=w2319:variant)
                          n797 = Variant To Flattened String(Variant=w2319) -> (data string=w2321:string)  [unwired: 1 out]
                          n798 = Flattened String To Variant(6:w2321, 7:w2323) -> (3:w2322:variant)  [unwired: 1 in, 1 out]
                        }
                        frame Error {
                        }
                      }
                    }
                    frame 9..14 {
                      # "SGL, DBL, EXT, CSG, CDB (0x09 .. 0x0E)"
                      n799 = Variant To Data(type=w2327, Variant=w2326) -> (data=w2328:cdb, error out=w2330:errorcluster)  [unwired: 1 in]
                      n800 = case shown="No Error" w2330 {
                        tunnel: w2332 -> [w2338 _]
                        tunnel: [w2337 w2339] -> w2331
                        tunnel: w2329 -> [_ w2339]
                        tunnel: w2328 -> [w2335 _]
                        tunnel: [TRUE _] -> w2325
                        frame No Error {
                          n801 = To Variant(anything=w2335) -> (Variant=w2334:variant)
                          n802 = Variant To Flattened String(Variant=w2334) -> (data string=w2336:string)  [unwired: 1 out]
                          n803 = Flattened String To Variant(6:w2336, 7:w2338) -> (3:w2337:variant)  [unwired: 1 in, 1 out]
                        }
                        frame Error {
                        }
                      }
                    }
                    frame 25..28, 30 {
                      # "Physical Units (0x19 .. 0x1E)"
                      n804 = Variant To Data(type=w2342, Variant=w2341) -> (data=w2343:cdb, error out=w2345:errorcluster)  [unwired: 1 in]
                      n805 = case shown="No Error" w2345 {
                        tunnel: w2347 -> [w2353 _]
                        tunnel: [w2352 w2354] -> w2346
                        tunnel: w2344 -> [_ w2354]
                        tunnel: w2343 -> [w2350 _]
                        tunnel: [TRUE _] -> w2340
                        frame No Error {
                          n806 = To Variant(anything=w2350) -> (Variant=w2349:variant)
                          n807 = Variant To Flattened String(Variant=w2349) -> (data string=w2351:string)  [unwired: 1 out]
                          n808 = Flattened String To Variant(6:w2351, 7:w2353) -> (3:w2352:variant)  [unwired: 1 in, 1 out]
                        }
                        frame Error {
                        }
                      }
                    }
                  }
                }
              }
            }
            frame 30 {
              # "CXT PhysUnit (0x1E)"
              n809 = Variant To Flattened String(Variant=w2361) -> (1:w2365:i16[])  [unwired: 1 out]
              n810 = call "TypeDescriptor_GetType.vi"("type descriptor"=w2365) -> ("Type"=w2355:u8)  [unwired: 9 in, 1 out]
              n811 = Equal?(x=w2356, y=w2355) -> (x = y?=w2359:bool)
              n812 = Compound Arithmetic op=OR(w2359, invert w2357) -> (w2358:bool)
              n813 = case shown="True" w2358 {
                tunnel: w2364 -> [w2366 w2373]
                tunnel: [w2366 w2372] -> w2363
                tunnel: w2362 -> [_ w2371]
                tunnel: w2355 -> [_ w2370]
                tunnel: w2361 -> [_ w2368]
                tunnel: [_ w2367] -> w2360
                frame False {
                }
                frame True {
                  w2369 = cxt 0.0+0.0i  # CXT
                  n814 = case shown="1..8" w2370 {
                    tunnel: w2373 -> [w2374 _ w2384 w2399 w2414]
                    tunnel: [w2374 w2376 w2386 w2401 w2416] -> w2372
                    tunnel: w2371 -> [_ w2377 w2387 w2402 w2417]
                    tunnel: w2369 -> [_ _ w2382 w2397 w2412]
                    tunnel: w2368 -> [_ w2379 w2381 w2396 w2411]
                    tunnel: [_ TRUE w2380 w2395 w2410] -> w2367
                    frame Default {
                      # "INCOMPATIBLE DATATYPES"
                    }
                    frame 30 {
                      # "CXT PhysUnit (0x1E)"
                      n815 = Variant To Flattened String(Variant=w2379) -> (data string=w2378:string)  [unwired: 1 out]
                      n816 = Flattened String To Variant(6:w2378, 7:w2377) -> (3:w2376:variant)  [unwired: 1 in, 1 out]
                    }
                    frame 1..8 {
                      # "I8, I16, I32, I64, U8, U16, U32, U64"
                      n817 = Variant To Data(type=w2382, Variant=w2381) -> (data=w2383:cxt, error out=w2385:errorcluster)  [unwired: 1 in]
                      n818 = case shown="No Error" w2385 {
                        tunnel: w2387 -> [w2393 _]
                        tunnel: [w2392 w2394] -> w2386
                        tunnel: w2384 -> [_ w2394]
                        tunnel: w2383 -> [w2390 _]
                        tunnel: [TRUE _] -> w2380
                        frame No Error {
                          n819 = To Variant(anything=w2390) -> (Variant=w2389:variant)
                          n820 = Variant To Flattened String(Variant=w2389) -> (data string=w2391:string)  [unwired: 1 out]
                          n821 = Flattened String To Variant(6:w2391, 7:w2393) -> (3:w2392:variant)  [unwired: 1 in, 1 out]
                        }
                        frame Error {
                        }
                      }
                    }
                    frame 9..14 {
                      # "SGL, DBL, EXT, CSG, CDB (0x09 .. 0x0E)"
                      n822 = Variant To Data(type=w2397, Variant=w2396) -> (data=w2398:cxt, error out=w2400:errorcluster)  [unwired: 1 in]
                      n823 = case shown="No Error" w2400 {
                        tunnel: w2402 -> [w2408 _]
                        tunnel: [w2407 w2409] -> w2401
                        tunnel: w2399 -> [_ w2409]
                        tunnel: w2398 -> [w2405 _]
                        tunnel: [TRUE _] -> w2395
                        frame No Error {
                          n824 = To Variant(anything=w2405) -> (Variant=w2404:variant)
                          n825 = Variant To Flattened String(Variant=w2404) -> (data string=w2406:string)  [unwired: 1 out]
                          n826 = Flattened String To Variant(6:w2406, 7:w2408) -> (3:w2407:variant)  [unwired: 1 in, 1 out]
                        }
                        frame Error {
                        }
                      }
                    }
                    frame 25..29 {
                      # "Physical Units (0x19 .. 0x1E)"
                      n827 = Variant To Data(type=w2412, Variant=w2411) -> (data=w2413:cxt, error out=w2415:errorcluster)  [unwired: 1 in]
                      n828 = case shown="No Error" w2415 {
                        tunnel: w2417 -> [w2423 _]
                        tunnel: [w2422 w2424] -> w2416
                        tunnel: w2414 -> [_ w2424]
                        tunnel: w2413 -> [w2420 _]
                        tunnel: [TRUE _] -> w2410
                        frame No Error {
                          n829 = To Variant(anything=w2420) -> (Variant=w2419:variant)
                          n830 = Variant To Flattened String(Variant=w2419) -> (data string=w2421:string)  [unwired: 1 out]
                          n831 = Flattened String To Variant(6:w2421, 7:w2423) -> (3:w2422:variant)  [unwired: 1 in, 1 out]
                        }
                        frame Error {
                        }
                      }
                    }
                  }
                }
              }
            }
            frame 33 {
              # "Boolean (0x21)"
              n832 = Variant To Flattened String(Variant=w2431) -> (1:w2435:i16[])  [unwired: 1 out]
              n833 = call "TypeDescriptor_GetType.vi"("type descriptor"=w2435) -> ("Type"=w2425:u8)  [unwired: 9 in, 1 out]
              n834 = Equal?(x=w2426, y=w2425) -> (x = y?=w2429:bool)
              n835 = Compound Arithmetic op=OR(w2429, invert w2427) -> (w2428:bool)
              n836 = case shown="True" w2428 {
                tunnel: w2434 -> [w2436 w2442]
                tunnel: [w2436 w2441] -> w2433
                tunnel: w2432 -> [_ w2440]
                tunnel: w2425 -> [_ w2439]
                tunnel: w2431 -> [_ w2438]
                tunnel: [_ w2437] -> w2430
                frame False {
                }
                frame True {
                  n837 = case shown="30" w2439 {
                    tunnel: w2442 -> [w2443 _ _ w2463]
                    tunnel: [w2443 w2453 w2458 w2465] -> w2441
                    tunnel: w2440 -> [_ w2454 w2459 w2467]
                    tunnel: w2438 -> [_ w2452 w2456 w2461]
                    tunnel: [_ TRUE TRUE w2460] -> w2437
                    frame Default {
                      # "INCOMPATIBLE DATATYPES"
                    }
                    frame 1..8 {
                      # "I8, I16, I32, I64, U8, U16, U32"
                      n838 = Variant To Flattened String(Variant=w2452) -> (data string=w2451:string)  [unwired: 1 out]
                      n839 = String To Byte Array(string=w2451) -> (unsigned byte array=w2449:u8[])
                      n840 = Not Equal To 0?(x=w2449) -> (x != 0?=w2450:bool[])
                      n841 = Or Array Elements(Boolean array=w2450) -> (logical OR=w2448:bool)
                      n842 = Select(t="\u0001" ("string"), s=w2448, f="\u0000" ("string")) -> (s? t:f=w2445:string)
                      n843 = Flattened String To Variant(6:w2445, 7:w2454) -> (3:w2453:variant)  [unwired: 1 in, 1 out]
                    }
                    frame 33 {
                      # "Boolean (0x21)"
                      n844 = Variant To Flattened String(Variant=w2456) -> (data string=w2457:string)  [unwired: 1 out]
                      n845 = Flattened String To Variant(6:w2457, 7:w2459) -> (3:w2458:variant)  [unwired: 1 in, 1 out]
                    }
                    frame 48 {
                      # "STRING (0x30)"
                      n846 = Variant To Data(type="", Variant=w2461) -> (data=w2462:string, error out=w2464:errorcluster)  [unwired: 1 in]
                      n847 = case shown="No Error" w2464 {
                        tunnel: w2467 -> [w2469 _]
                        tunnel: [w2470 w2481] -> w2465
                        tunnel: w2463 -> [w2471 w2481]
                        tunnel: w2462 -> [w2473 _]
                        tunnel: [TRUE _] -> w2460
                        frame No Error {
                          n848 = To Lower Case(string=w2473) -> (all lower case string=w2472:string)
                          n849 = case shown="\"true\"" w2472 {
                            tunnel: w2471 -> [w2474 _ _]
                            tunnel: [w2474 w2475 w2478] -> w2470
                            tunnel: w2469 -> [_ w2477 w2480]
                            frame Default {
                            }
                            frame "true" {
                              n850 = Flattened String To Variant(6:"\u0001" ("data string"), 7:w2477) -> (3:w2475:variant)  [unwired: 1 in, 1 out]
                            }
                            frame "false" {
                              n851 = Flattened String To Variant(6:"\u0000" ("data string"), 7:w2480) -> (3:w2478:variant)  [unwired: 1 in, 1 out]
                            }
                          }
                        }
                        frame Error {
                        }
                      }
                    }
                  }
                }
              }
            }
            frame 48 {
              # "STRING (0x30)"
              n852 = Variant To Flattened String(Variant=w2490) -> (data string=w2489:string, 1:w2488:i16[])
              n853 = call "TypeDescriptor_GetType.vi"("type descriptor"=w2488) -> ("Type"=w2483:u8, "type descriptor dup"=w2491:i16[])  [unwired: 9 in]
              n854 = Equal?(x=w2484, y=w2483) -> (x = y?=w2486:bool)
              n855 = Compound Arithmetic op=OR(w2486, invert w2482) -> (w2485:bool)
              n856 = case shown="True" w2485 {
                tunnel: w2494 -> [w2495 w2503]
                tunnel: [w2495 w2502] -> w2493
                tunnel: w2492 -> [_ w2501]
                tunnel: w2483 -> [_ w2500]
                tunnel: w2491 -> [_ w2499]
                tunnel: w2490 -> [_ w2498]
                tunnel: w2489 -> [_ w2497]
                tunnel: [_ w2496] -> w2487
                frame False {
                }
                frame True {
                  n857 = case shown="9" w2500 {
                    tunnel: w2497 -> [_ w2508 _ _ _ _ _ _ _ _ _ _ _ _ _ _ _ _ w2773]
                    tunnel: w2503 -> [w2504 _ w2512 w2528 w2545 w2561 w2577 w2593 w2609 w2625 w2641 w2657 w2673 w2689 w2705 w2721 w2737 w2753 _]
                    tunnel: [w2504 w2507 w2514 w2530 w2547 w2563 w2579 w2595 w2611 w2627 w2643 w2659 w2675 w2691 w2707 w2723 w2739 w2755 w2774] -> w2502
                    tunnel: w2501 -> [_ w2506 w2516 w2532 w2548 w2564 w2580 w2596 w2612 w2628 w2644 w2660 w2676 w2692 w2708 w2724 w2740 w2756 w2775]
                    tunnel: w2499 -> [_ _ _ _ _ _ _ _ _ _ _ _ _ _ _ _ _ _ w2769]
                    tunnel: w2498 -> [_ _ w2510 w2526 w2542 w2558 w2574 w2590 w2606 w2622 w2638 w2654 w2670 w2686 w2702 w2718 w2734 w2750 _]
                    tunnel: [_ TRUE w2509 w2525 w2541 w2557 w2573 w2589 w2605 w2621 w2637 w2653 w2669 w2685 w2701 w2717 w2733 w2749 TRUE] -> w2496
                    frame Default {
                      # "INCOMPATIBLE DATATYPES"
                    }
                    frame 48 {
                      # "STRING (0x30)"
                      n858 = Flattened String To Variant(6:w2508, 7:w2506) -> (3:w2507:variant)  [unwired: 1 in, 1 out]
                    }
                    frame 50 {
                      # "PATH (0x32)"
                      n859 = Variant To Data(type=path "", Variant=w2510) -> (data=w2511:path, error out=w2513:errorcluster)  [unwired: 1 in]
                      n860 = case shown="No Error" w2513 {
                        tunnel: w2516 -> [w2523 _]
                        tunnel: [w2522 w2524] -> w2514
                        tunnel: w2512 -> [_ w2524]
                        tunnel: w2511 -> [w2519 _]
                        tunnel: [TRUE _] -> w2509
                        frame No Error {
                          n861 = Path To String(path=w2519) -> (string=w2521:string)
                          n862 = To Variant(anything=w2521) -> (Variant=w2520:variant)
                          n863 = Variant To Flattened String(Variant=w2520) -> (data string=w2518:string)  [unwired: 1 out]
                          n864 = Flattened String To Variant(6:w2518, 7:w2523) -> (3:w2522:variant)  [unwired: 1 in, 1 out]
                        }
                        frame Error {
                        }
                      }
                    }
                    frame 33 {
                      # "BOOLEAN (0x21)"
                      n865 = Variant To Data(type=FALSE, Variant=w2526) -> (data=w2527:bool, error out=w2529:errorcluster)  [unwired: 1 in]
                      n866 = case shown="No Error" w2529 {
                        tunnel: w2532 -> [w2539 _]
                        tunnel: [w2538 w2540] -> w2530
                        tunnel: w2528 -> [_ w2540]
                        tunnel: w2527 -> [w2535 _]
                        tunnel: [TRUE _] -> w2525
                        frame No Error {
                          n867 = Format Into String(w2535) -> (resulting string=w2534:string)  [unwired: 3 in, 1 out]
                          n868 = To Variant(anything=w2534) -> (Variant=w2537:variant)
                          n869 = Variant To Flattened String(Variant=w2537) -> (data string=w2536:string)  [unwired: 1 out]
                          n870 = Flattened String To Variant(6:w2536, 7:w2539) -> (3:w2538:variant)  [unwired: 1 in, 1 out]
                        }
                        frame Error {
                        }
                      }
                    }
                    frame 1 {
                      # "I8 (0x01)"
                      n871 = Variant To Data(type=i8 0, Variant=w2542) -> (data=w2544:i8, error out=w2546:errorcluster)  [unwired: 1 in]
                      n872 = case shown="No Error" w2546 {
                        tunnel: w2548 -> [w2555 _]
                        tunnel: [w2554 w2556] -> w2547
                        tunnel: w2545 -> [_ w2556]
                        tunnel: w2544 -> [w2551 _]
                        tunnel: [TRUE _] -> w2541
                        frame No Error {
                          n873 = Format Into String(w2551) -> (resulting string=w2550:string)  [unwired: 3 in, 1 out]
                          n874 = To Variant(anything=w2550) -> (Variant=w2553:variant)
                          n875 = Variant To Flattened String(Variant=w2553) -> (data string=w2552:string)  [unwired: 1 out]
                          n876 = Flattened String To Variant(6:w2552, 7:w2555) -> (3:w2554:variant)  [unwired: 1 in, 1 out]
                        }
                        frame Error {
                        }
                      }
                    }
                    frame 2 {
                      # "I16 (0x02)"
                      n877 = Variant To Data(type=i16 0, Variant=w2558) -> (data=w2560:i16, error out=w2562:errorcluster)  [unwired: 1 in]
                      n878 = case shown="No Error" w2562 {
                        tunnel: w2564 -> [w2571 _]
                        tunnel: [w2570 w2572] -> w2563
                        tunnel: w2561 -> [_ w2572]
                        tunnel: w2560 -> [w2567 _]
                        tunnel: [TRUE _] -> w2557
                        frame No Error {
                          n879 = Format Into String(w2567) -> (resulting string=w2566:string)  [unwired: 3 in, 1 out]
                          n880 = To Variant(anything=w2566) -> (Variant=w2569:variant)
                          n881 = Variant To Flattened String(Variant=w2569) -> (data string=w2568:string)  [unwired: 1 out]
                          n882 = Flattened String To Variant(6:w2568, 7:w2571) -> (3:w2570:variant)  [unwired: 1 in, 1 out]
                        }
                        frame Error {
                        }
                      }
                    }
                    frame 3 {
                      # "I32 (0x03)"
                      n883 = Variant To Data(type=0, Variant=w2574) -> (data=w2576:i32, error out=w2578:errorcluster)  [unwired: 1 in]
                      n884 = case shown="No Error" w2578 {
                        tunnel: w2580 -> [w2587 _]
                        tunnel: [w2586 w2588] -> w2579
                        tunnel: w2577 -> [_ w2588]
                        tunnel: w2576 -> [w2583 _]
                        tunnel: [TRUE _] -> w2573
                        frame No Error {
                          n885 = Format Into String(w2583) -> (resulting string=w2582:string)  [unwired: 3 in, 1 out]
                          n886 = To Variant(anything=w2582) -> (Variant=w2585:variant)
                          n887 = Variant To Flattened String(Variant=w2585) -> (data string=w2584:string)  [unwired: 1 out]
                          n888 = Flattened String To Variant(6:w2584, 7:w2587) -> (3:w2586:variant)  [unwired: 1 in, 1 out]
                        }
                        frame Error {
                        }
                      }
                    }
                    frame 4 {
                      # "I64 (0x04)"
                      n889 = Variant To Data(type=i64 0, Variant=w2590) -> (data=w2592:i64, error out=w2594:errorcluster)  [unwired: 1 in]
                      n890 = case shown="No Error" w2594 {
                        tunnel: w2596 -> [w2603 _]
                        tunnel: [w2602 w2604] -> w2595
                        tunnel: w2593 -> [_ w2604]
                        tunnel: w2592 -> [w2599 _]
                        tunnel: [TRUE _] -> w2589
                        frame No Error {
                          n891 = Format Into String(w2599) -> (resulting string=w2598:string)  [unwired: 3 in, 1 out]
                          n892 = To Variant(anything=w2598) -> (Variant=w2601:variant)
                          n893 = Variant To Flattened String(Variant=w2601) -> (data string=w2600:string)  [unwired: 1 out]
                          n894 = Flattened String To Variant(6:w2600, 7:w2603) -> (3:w2602:variant)  [unwired: 1 in, 1 out]
                        }
                        frame Error {
                        }
                      }
                    }
                    frame 5 {
                      # "U8 (0x05)"
                      n895 = Variant To Data(type=u8 0, Variant=w2606) -> (data=w2608:u8, error out=w2610:errorcluster)  [unwired: 1 in]
                      n896 = case shown="No Error" w2610 {
                        tunnel: w2612 -> [w2619 _]
                        tunnel: [w2618 w2620] -> w2611
                        tunnel: w2609 -> [_ w2620]
                        tunnel: w2608 -> [w2615 _]
                        tunnel: [TRUE _] -> w2605
                        frame No Error {
                          n897 = Format Into String(w2615) -> (resulting string=w2614:string)  [unwired: 3 in, 1 out]
                          n898 = To Variant(anything=w2614) -> (Variant=w2617:variant)
                          n899 = Variant To Flattened String(Variant=w2617) -> (data string=w2616:string)  [unwired: 1 out]
                          n900 = Flattened String To Variant(6:w2616, 7:w2619) -> (3:w2618:variant)  [unwired: 1 in, 1 out]
                        }
                        frame Error {
                        }
                      }
                    }
                    frame 6 {
                      # "U16 (0x06)"
                      n901 = Variant To Data(type=u16 0, Variant=w2622) -> (data=w2624:u16, error out=w2626:errorcluster)  [unwired: 1 in]
                      n902 = case shown="No Error" w2626 {
                        tunnel: w2628 -> [w2635 _]
                        tunnel: [w2634 w2636] -> w2627
                        tunnel: w2625 -> [_ w2636]
                        tunnel: w2624 -> [w2631 _]
                        tunnel: [TRUE _] -> w2621
                        frame No Error {
                          n903 = Format Into String(w2631) -> (resulting string=w2630:string)  [unwired: 3 in, 1 out]
                          n904 = To Variant(anything=w2630) -> (Variant=w2633:variant)
                          n905 = Variant To Flattened String(Variant=w2633) -> (data string=w2632:string)  [unwired: 1 out]
                          n906 = Flattened String To Variant(6:w2632, 7:w2635) -> (3:w2634:variant)  [unwired: 1 in, 1 out]
                        }
                        frame Error {
                        }
                      }
                    }
                    frame 7 {
                      # "U32 (0x07)"
                      n907 = Variant To Data(type=u32 0, Variant=w2638) -> (data=w2640:u32, error out=w2642:errorcluster)  [unwired: 1 in]
                      n908 = case shown="No Error" w2642 {
                        tunnel: w2644 -> [w2651 _]
                        tunnel: [w2650 w2652] -> w2643
                        tunnel: w2641 -> [_ w2652]
                        tunnel: w2640 -> [w2647 _]
                        tunnel: [TRUE _] -> w2637
                        frame No Error {
                          n909 = Format Into String(w2647) -> (resulting string=w2646:string)  [unwired: 3 in, 1 out]
                          n910 = To Variant(anything=w2646) -> (Variant=w2649:variant)
                          n911 = Variant To Flattened String(Variant=w2649) -> (data string=w2648:string)  [unwired: 1 out]
                          n912 = Flattened String To Variant(6:w2648, 7:w2651) -> (3:w2650:variant)  [unwired: 1 in, 1 out]
                        }
                        frame Error {
                        }
                      }
                    }
                    frame 8 {
                      # "U64 (0x08)"
                      n913 = Variant To Data(type=u64 0, Variant=w2654) -> (data=w2656:u64, error out=w2658:errorcluster)  [unwired: 1 in]
                      n914 = case shown="No Error" w2658 {
                        tunnel: w2660 -> [w2667 _]
                        tunnel: [w2666 w2668] -> w2659
                        tunnel: w2657 -> [_ w2668]
                        tunnel: w2656 -> [w2663 _]
                        tunnel: [TRUE _] -> w2653
                        frame No Error {
                          n915 = Format Into String(w2663) -> (resulting string=w2662:string)  [unwired: 3 in, 1 out]
                          n916 = To Variant(anything=w2662) -> (Variant=w2665:variant)
                          n917 = Variant To Flattened String(Variant=w2665) -> (data string=w2664:string)  [unwired: 1 out]
                          n918 = Flattened String To Variant(6:w2664, 7:w2667) -> (3:w2666:variant)  [unwired: 1 in, 1 out]
                        }
                        frame Error {
                        }
                      }
                    }
                    frame 9 {
                      # "SGL (0x09)"
                      n919 = Variant To Data(type=sgl 0.0, Variant=w2670) -> (data=w2672:sgl, error out=w2674:errorcluster)  [unwired: 1 in]
                      n920 = case shown="No Error" w2674 {
                        tunnel: w2676 -> [w2683 _]
                        tunnel: [w2682 w2684] -> w2675
                        tunnel: w2673 -> [_ w2684]
                        tunnel: w2672 -> [w2678 _]
                        tunnel: [TRUE _] -> w2669
                        frame No Error {
                          n921 = call "SingleFloat (Scalar) to String.vi"("Value (Single)"=w2678) -> ("Value (String)"=w2677:string)  [unwired: 10 in]
                          n922 = To Variant(anything=w2677) -> (Variant=w2681:variant)
                          n923 = Variant To Flattened String(Variant=w2681) -> (data string=w2680:string)  [unwired: 1 out]
                          n924 = Flattened String To Variant(6:w2680, 7:w2683) -> (3:w2682:variant)  [unwired: 1 in, 1 out]
                        }
                        frame Error {
                        }
                      }
                    }
                    frame 10 {
                      # "DBL (0x0A)"
                      n925 = Variant To Data(type=0.0, Variant=w2686) -> (data=w2688:dbl, error out=w2690:errorcluster)  [unwired: 1 in]
                      n926 = case shown="No Error" w2690 {
                        tunnel: w2692 -> [w2699 _]
                        tunnel: [w2698 w2700] -> w2691
                        tunnel: w2689 -> [_ w2700]
                        tunnel: w2688 -> [w2694 _]
                        tunnel: [TRUE _] -> w2685
                        frame No Error {
                          n927 = call "DoubleFloat (Scalar) to String.vi"("Value (Double)"=w2694) -> ("Value (String)"=w2693:string)  [unwired: 10 in]
                          n928 = To Variant(anything=w2693) -> (Variant=w2697:variant)
                          n929 = Variant To Flattened String(Variant=w2697) -> (data string=w2696:string)  [unwired: 1 out]
                          n930 = Flattened String To Variant(6:w2696, 7:w2699) -> (3:w2698:variant)  [unwired: 1 in, 1 out]
                        }
                        frame Error {
                        }
                      }
                    }
                    frame 11 {
                      # "EXT (0x0B)"
                      n931 = Variant To Data(type=ext 0.0, Variant=w2702) -> (data=w2704:ext, error out=w2706:errorcluster)  [unwired: 1 in]
                      n932 = case shown="No Error" w2706 {
                        tunnel: w2708 -> [w2715 _]
                        tunnel: [w2714 w2716] -> w2707
                        tunnel: w2705 -> [_ w2716]
                        tunnel: w2704 -> [w2710 _]
                        tunnel: [TRUE _] -> w2701
                        frame No Error {
                          n933 = call "ExtendedFloat (Scalar) to String.vi"("Value (Extended)"=w2710) -> ("Value (String)"=w2709:string)  [unwired: 10 in]
                          n934 = To Variant(anything=w2709) -> (Variant=w2713:variant)
                          n935 = Variant To Flattened String(Variant=w2713) -> (data string=w2712:string)  [unwired: 1 out]
                          n936 = Flattened String To Variant(6:w2712, 7:w2715) -> (3:w2714:variant)  [unwired: 1 in, 1 out]
                        }
                        frame Error {
                        }
                      }
                    }
                    frame 12 {
                      # "CSG (0x0C)"
                      n937 = Variant To Data(type=csg 0.0+0.0i, Variant=w2718) -> (data=w2720:csg, error out=w2722:errorcluster)  [unwired: 1 in]
                      n938 = case shown="No Error" w2722 {
                        tunnel: w2724 -> [w2731 _]
                        tunnel: [w2730 w2732] -> w2723
                        tunnel: w2721 -> [_ w2732]
                        tunnel: w2720 -> [w2726 _]
                        tunnel: [TRUE _] -> w2717
                        frame No Error {
                          n939 = call "SingleComplex (Scalar) to String.vi"("Value (CSG)"=w2726) -> ("Value (String)"=w2725:string)  [unwired: 10 in]
                          n940 = To Variant(anything=w2725) -> (Variant=w2729:variant)
                          n941 = Variant To Flattened String(Variant=w2729) -> (data string=w2728:string)  [unwired: 1 out]
                          n942 = Flattened String To Variant(6:w2728, 7:w2731) -> (3:w2730:variant)  [unwired: 1 in, 1 out]
                        }
                        frame Error {
                        }
                      }
                    }
                    frame 13 {
                      # "CDB (0x0D)"
                      n943 = Variant To Data(type=cdb 0.0+0.0i, Variant=w2734) -> (data=w2736:cdb, error out=w2738:errorcluster)  [unwired: 1 in]
                      n944 = case shown="No Error" w2738 {
                        tunnel: w2740 -> [w2747 _]
                        tunnel: [w2746 w2748] -> w2739
                        tunnel: w2737 -> [_ w2748]
                        tunnel: w2736 -> [w2742 _]
                        tunnel: [TRUE _] -> w2733
                        frame No Error {
                          n945 = call "DoubleComplex (Scalar) to String.vi"("Value (CDB)"=w2742) -> ("Value (String)"=w2741:string)  [unwired: 10 in]
                          n946 = To Variant(anything=w2741) -> (Variant=w2745:variant)
                          n947 = Variant To Flattened String(Variant=w2745) -> (data string=w2744:string)  [unwired: 1 out]
                          n948 = Flattened String To Variant(6:w2744, 7:w2747) -> (3:w2746:variant)  [unwired: 1 in, 1 out]
                        }
                        frame Error {
                        }
                      }
                    }
                    frame 14 {
                      # "CXT (0x0E)"
                      n949 = Variant To Data(type=cxt 0.0+0.0i, Variant=w2750) -> (data=w2752:cxt, error out=w2754:errorcluster)  [unwired: 1 in]
                      n950 = case shown="No Error" w2754 {
                        tunnel: w2756 -> [w2763 _]
                        tunnel: [w2762 w2764] -> w2755
                        tunnel: w2753 -> [_ w2764]
                        tunnel: w2752 -> [w2758 _]
                        tunnel: [TRUE _] -> w2749
                        frame No Error {
                          n951 = call "ExtendedComplex (Scalar) to String.vi"("Value (CXT)"=w2758) -> ("Value (String)"=w2757:string)  [unwired: 10 in]
                          n952 = To Variant(anything=w2757) -> (Variant=w2761:variant)
                          n953 = Variant To Flattened String(Variant=w2761) -> (data string=w2760:string)  [unwired: 1 out]
                          n954 = Flattened String To Variant(6:w2760, 7:w2763) -> (3:w2762:variant)  [unwired: 1 in, 1 out]
                        }
                        frame Error {
                        }
                      }
                    }
                    frame 21 {
                      # "EnumU8 (0x15)"
                      n955 = String To Byte Array(string=w2773) -> (unsigned byte array=w2770:u8[])
                      n956 = Index Array(array=w2770) -> (element=w2766:u8)  [unwired: 1 in]
                      n957 = call "TypeDescriptor_ListElementNames.vi"("type descriptor"=w2769) -> ("element names"=w2768:string[])  [unwired: 7 in, 3 out]
                      n958 = Index Array(array=w2768, index=w2766) -> (element=w2767:string)
                      n959 = To Variant(anything=w2767) -> (Variant=w2772:variant)
                      n960 = Variant To Flattened String(Variant=w2772) -> (data string=w2771:string)  [unwired: 1 out]
                      n961 = Flattened String To Variant(6:w2771, 7:w2775) -> (3:w2774:variant)  [unwired: 1 in, 1 out]
                    }
                  }
                }
              }
            }
            frame 50 {
              # "PATH (0x32)"
              n962 = Variant To Flattened String(Variant=w2788) -> (data string=w2787:string, 1:w2786:i16[])
              n963 = call "TypeDescriptor_GetType.vi"("type descriptor"=w2786) -> ("Type"=w2778:u8, "type descriptor dup"=w2782:i16[])  [unwired: 9 in]
              n964 = Equal?(x=w2779, y=w2778) -> (x = y?=w2780:bool)
              n965 = Compound Arithmetic op=OR(w2780, invert w2777) -> (w2776:bool)
              n966 = case shown="True" w2776 {
                tunnel: w2787 -> [_ w2796]
                tunnel: w2785 -> [w2789 w2795]
                tunnel: [w2789 w2794] -> w2784
                tunnel: w2783 -> [_ w2793]
                tunnel: w2782 -> [_ w2792]
                tunnel: [_ w2791] -> w2781
                tunnel: w2778 -> [_ w2790]
                frame False {
                }
                frame True {
                  n967 = case shown="32" w2790 {
                    tunnel: w2796 -> [_ w2801 w2810]
                    tunnel: w2795 -> [w2797 _ w2804]
                    tunnel: [w2797 w2800 w2806] -> w2794
                    tunnel: w2793 -> [_ w2799 w2812]
                    tunnel: w2792 -> [_ _ w2811]
                    tunnel: [_ TRUE w2802] -> w2791
                    frame Default {
                      # "INCOMPATIBLE DATATYPES"
                    }
                    frame 50 {
                      # "PATH (0x32)"
                      n968 = Flattened String To Variant(6:w2801, 7:w2799) -> (3:w2800:variant)  [unwired: 1 in, 1 out]
                    }
                    frame 48 {
                      # "STRING (0x30)"
                      n969 = Flattened String To Variant(6:w2810, 7:w2811) -> (0:w2807:errorcluster, 3:w2809:variant)  [unwired: 1 in]
                      n970 = Variant To Data(error in=w2807, type="", Variant=w2809) -> (data=w2803:string, error out=w2805:errorcluster)
                      n971 = case shown="No Error" w2805 {
                        tunnel: w2812 -> [w2819 _]
                        tunnel: [w2818 w2820] -> w2806
                        tunnel: w2804 -> [_ w2820]
                        tunnel: w2803 -> [w2814 _]
                        tunnel: [TRUE _] -> w2802
                        frame No Error {
                          n972 = call "String to Path.vi"("common path"=w2814) -> ("specific path"=w2813:path)  [unwired: 10 in]
                          n973 = To Variant(anything=w2813) -> (Variant=w2817:variant)
                          n974 = Variant To Flattened String(Variant=w2817) -> (data string=w2816:string)  [unwired: 1 out]
                          n975 = Flattened String To Variant(6:w2816, 7:w2819) -> (3:w2818:variant)  [unwired: 1 in, 1 out]
                        }
                        frame Error {
                        }
                      }
                    }
                  }
                }
              }
            }
            frame 64 {
              # "ARRAY (0x40)"
              n976 = Variant To Flattened String(Variant=w2828) -> (data string=w2842:string, 1:w2822:i16[])
              n977 = call "TypeDescriptor_GetArrayElementTypeDescriptor.vi"("Array Type Descriptor"=w2827) -> ("Element Type Descriptor"=w2825:i16[], "Array Type Descriptor dup"=w2826:i16[])  [unwired: 9 in]
              n978 = call "TypeDescriptor_GetArrayElementTypeDescriptor.vi"("Array Type Descriptor"=w2822) -> ("Element Type Descriptor"=w2823:i16[])  [unwired: 9 in, 1 out]
              n979 = call "TypeDescriptor_GetType.vi"("type descriptor"=w2822) -> ("Type"=w2836:u8, "type descriptor dup"=w2835:i16[])  [unwired: 9 in]
              n980 = call "TypeDescriptor_GetType.vi"("type descriptor"=w2825) -> ("Type"=w2824:u8)  [unwired: 9 in, 1 out]
              n981 = Equal?(x=w2837, y=w2836) -> (x = y?=w2838:bool)
              n982 = call "TypeDescriptor_GetType.vi"("type descriptor"=w2823) -> ("Type"=w2821:u8)  [unwired: 9 in, 1 out]
              n983 = Equal?(x=w2824, y=w2821) -> (x = y?=w2831:bool)
              n984 = call <vilib>:"TD_Compare Types.vi"("Type descriptor 2"=w2835, "Type descriptor"=w2826) -> ("Types Wireable?"=w2834:bool)  [unwired: 9 in]
              n985 = Compound Arithmetic op=OR(w2838, invert w2830) -> (w2832:bool)
              n986 = Compound Arithmetic op=OR(w2831, invert w2830) -> (w2829:bool)
              n987 = Compound Arithmetic op=AND(w2834, w2832, w2829) -> (w2833:bool)
              n988 = case shown="False" w2833 {
                tunnel: w2842 -> [w2849 _]
                tunnel: w2841 -> [w2847 w2852]
                tunnel: [w2845 w2855] -> w2840
                tunnel: w2826 -> [w2848 _]
                tunnel: w2835 -> [_ _]
                tunnel: [w2843 w2854] -> w2839
                tunnel: w2836 -> [_ _]
                tunnel: w2828 -> [_ w2853]
                frame True {
                  n989 = Flattened String To Variant(6:w2849, 7:w2848) -> (0:w2844:errorcluster, 3:w2846:variant)  [unwired: 1 in]
                  n990 = Select(t=w2847, s=w2844, f=w2846) -> (s? t:f=w2845:variant)
                  n991 = Not(x=w2844) -> (.not. x?=w2843:bool)
                }
                frame False {
                  # "Type Casting id subtypes\nCheck if wireable"
                  n992 = Variant To Data(type=w2852, Variant=w2853) -> (data=w2851:variant, error out=w2850:errorcluster)  [unwired: 1 in]
                  n993 = Select(t=w2852, s=w2850, f=w2851) -> (s? t:f=w2855:variant)
                  n994 = Not(x=w2850) -> (.not. x?=w2854:bool)
                }
              }
            }
            frame 80 {
              # "CLUSTER (0x50)"
              n995 = call "Variant_ExtractClusterElements.vi"("Cluster"=w2857) -> ("Elements"=w2856:variant[])  [unwired: 8 in, 2 out]
              n996 = call "Variant_ExtractClusterElements.vi"("Cluster"=w2868) -> ("name"=w2858:string, "Elements"=w2864:variant[])  [unwired: 8 in, 1 out]
              n997 = for {
                tunnel: w2864 -> [w2874] mode=indexing
                tunnel: [w2879] -> w2863 mode=indexing
                shift-right: [w2878] -> w2859
                shift-left: variant ("variant") -> [w2877]
                tunnel: w2856 -> [w2875] mode=indexing
                n998 = call "Variant_GetName.vi"("Variant"=w2874) -> ("Name"=w2876:string, "Variant dup"=w2879:variant)  [unwired: 8 in, 1 out]
                n999 = Set Variant Attribute(Variant=w2877, name=w2876, value=w2875) -> (Variant out=w2878:variant)  [unwired: 1 in, 2 out]
              }
              n1000 = for {
                tunnel: w2865 -> [w2873]
                tunnel: w2863 -> [w2872] mode=indexing
                tunnel: [w2871] -> w2862 mode=indexing
                tunnel: [w2870] -> w2861 mode=indexing
                tunnel: w2859 -> [w2869]
                n1001 = call "Variant_KVP to Strict Variant (Standard).vi"("KVP"=w2869, "Strict type matching? (F)"=w2873, "Default Value"=w2872) -> ("any found?"=w2870:bool, "Value"=w2871:variant)  [unwired: 5 in, 2 out]
              }
              n1002 = call "Variant_BuildClusterFromElementArray.vi"("name"=w2858, "Elements"=w2862) -> ("Cluster"=w2866:variant)  [unwired: 9 in]
              n1003 = Or Array Elements(Boolean array=w2861) -> (logical OR=w2867:bool)
            }
            frame 112 {
              # "REFNUMS (0x70)"
              n1004 = Variant To Flattened String(Variant=w2894) -> (data string=w2893:string, 1:w2892:i16[])
              n1005 = call "TypeDescriptor_GetType.vi"("type descriptor"=w2892) -> ("Type"=w2884:u8, "type descriptor dup"=w2889:i16[])  [unwired: 9 in]
              n1006 = Equal?(x=w2880, y=w2884) -> (x = y?=w2883:bool)
              n1007 = Index Array(array=w2887, index=2) -> (element=w2886:i16)
              n1008 = Compound Arithmetic op=OR(w2883, invert w2882) -> (w2881:bool)
              n1009 = case shown="True" w2881 {
                tunnel: w2893 -> [_ w2903]
                tunnel: w2891 -> [w2895 w2902]
                tunnel: [w2895 w2901] -> w2890
                tunnel: w2889 -> [_ w2900]
                tunnel: w2887 -> [_ w2899]
                tunnel: w2886 -> [_ w2898]
                tunnel: [_ w2897] -> w2885
                tunnel: w2884 -> [_ w2896]
                frame False {
                }
                frame True {
                  n1010 = case shown="70" w2896 {
                    tunnel: w2903 -> [_ w2908 w2923]
                    tunnel: w2902 -> [w2904 w2906 w2920]
                    tunnel: [w2904 w2907 w2919] -> w2901
                    tunnel: w2899 -> [_ w2909 w2922]
                    tunnel: w2900 -> [_ w2912 _]
                    tunnel: w2898 -> [_ w2911 w2921]
                    tunnel: [_ _ w2918] -> w2897
                    frame Default {
                      # "INCOMPATIBLE DATATYPES"
                    }
                    frame 112 {
                      # "Check if subtype matches"
                      # "REFNUM - CHECK SUBTYPE"
                      n1011 = Index Array(array=w2912, index=2) -> (element=w2910:i16)
                      n1012 = Equal?(x=w2911, y=w2910) -> (x = y?=w2905:bool)
                      n1013 = case shown="True" w2905 {
                        tunnel: w2909 -> [_ w2917]
                        tunnel: w2908 -> [_ w2916]
                        tunnel: [w2914 w2915] -> w2907
                        tunnel: w2906 -> [w2914 _]
                        frame False {
                        }
                        frame True {
                          n1014 = Flattened String To Variant(6:w2916, 7:w2917) -> (3:w2915:variant)  [unwired: 1 in, 1 out]
                        }
                      }
                    }
                    frame 1..8 {
                      # "4-byte types or higher resolution"
                      n1015 = case shown="1, 4, 8, 9, 11, 12, 14, 15, 17, 19" w2921 {
                        tunnel: w2923 -> [_ w2934]
                        tunnel: w2922 -> [_ w2928]
                        tunnel: w2920 -> [w2924 _]
                        tunnel: [w2924 w2926] -> w2919
                        tunnel: [_ TRUE] -> w2918
                        frame Default {
                        }
                        frame 1, 4, 8, 9, 17, 18, 20, 21, 23, 25 {
                          # "Any types that have at least\n4 bytes."
                          n1016 = String To Byte Array(string=w2934) -> (unsigned byte array=w2933:u8[])
                          n1017 = Reverse 1D Array(array=w2933) -> (reversed array=w2932:u8[])
                          n1018 = Array Subset(array=w2932, length=4) -> (w2930:u8[])  [unwired: 1 in]
                          n1019 = Reverse 1D Array(array=w2930) -> (reversed array=w2929:u8[])
                          n1020 = Byte Array To String(unsigned byte array=w2929) -> (string=w2927:string)
                          n1021 = Flattened String To Variant(6:w2927, 7:w2928) -> (3:w2926:variant)  [unwired: 1 in, 1 out]
                        }
                      }
                    }
                  }
                }
              }
            }
          }
        }
      }
    }
  }
  "Value" <- w13
  "name out" <- w14
  "any found?" <- w9
  "all found?" <- w10
